vi "Position_TOTAL_R20.vi"(5 "Distance Between \nCameras  (*unit)":sgl=2.5) -> (12 "dX, dY\nLeft Cam":cluster{"X":sgl[], "Y":sgl[]}={"X"=[-5.750775, -4.1849813, -3.081379, -2.0098581, 0.0], "Y"=[7.9585915, 7.9595685, 7.960258, 7.960927, 0.0]}, 13 "Position Valid":bool=TRUE, 14 "Left Camera Real Coordinates":cluster{"X":sgl, "Y":sgl}={"X"=7.9602513, "Y"=5.592073}, 16 "dX, dY\nRight Cam":cluster{"X":sgl[], "Y":sgl[]}={"X"=[-7.3032045, -5.737411, -4.6338086, -3.5622878, -1.5524296], "Y"=[7.2714148, 7.2723923, 7.2730813, 7.273751, -0.68717635]}, 18 "Robot Coordinates":cluster{"X":sgl, "Y":sgl}={"X"=7.616663, "Y"=6.3682876}, 19 "Orietnation\n(current)":sgl=-23.843685 format="%#_13g")   [LabVIEW 2015]
uses:
  <vilib>/Analysis/NI_AALPro.lvlib
  <vilib>/myRIO/Instrument Drivers/Onboard IO/DIO/DIO.lvlib
  <vilib>/Analysis/coordinate.llb/2D Cartesian Coordinate Rotation (Array).vi
  <vilib>/Instr/_visa.llb/VISA Configure Serial Port (Instr).vi
panel:
  out "Current Cam State - L":T1(ring)
  out "Valid Beacon Sets_":bool[](array[boolean])=[TRUE, TRUE, TRUE, TRUE, FALSE]
  in  "Distance Threshold\nRef Triangles (*unit)":sgl=30.0
  out "dA2 4":sgl=9.6935425 format="%#_13g"
  out "dA2 2":sgl=9.6935425 format="%#_13g"
  out "dA2 3":sgl=9.6935425 format="%#_13g"
  out "Current Cam State - R":T1(ring)
  out "Beacon Scales - Left":sgl[](array[numeric])=[76.306, 116.841255, 157.35043, 195.67218, 0.0]
  out "Beacon Scales - Right":sgl[](array[numeric])=[76.306, 116.841255, 157.35043, 195.67218, 0.0]
  in  "New Orientation \nThreshold":sgl=10.0
  in  "Moving Average\nWindow Length":u8=5
  out "Current Recovery State -L":enum16{"Generic Sweep", "Recovery Search"}(ring)=enum."Recovery Search"
  out "Current Move Delta - L 2":u16
  out "Next Recovery State - Left":enum16{"Generic Sweep", "Recovery Search"}(ring)=enum."Recovery Search"
  out "Next Recovery State - Right":enum16{"Generic Sweep", "Recovery Search"}(ring)=enum."Recovery Search"
  out "Current Recovery State - Right":enum16{"Generic Sweep", "Recovery Search"}(ring)=enum."Recovery Search"
  in  "Initial Recovery State  - Right":enum16{"Generic Sweep", "Recovery Search"}(ring)=enum."Recovery Search"
  in  "Initial Recovery State - L":enum16{"Generic Sweep", "Recovery Search"}(ring)=enum."Recovery Search"
  out "Next Tracking State - Right":enum16{"Track", "Reactive Predict", ""}(ring)
  out "Current Tracking State - Right 2":enum16{"Track", "Reactive Predict", ""}(ring)
  in  "Initial Tracking State - Right":enum16{"Track", "Reactive Predict", ""}(ring)
  out "Last Track Angle - R":sgl=98.61328
  out "Next Tracking State - Left":enum16{"Track", "Reactive Predict", ""}(ring)
  in  "Initial Tracking State - Left":enum16{"Track", "Reactive Predict", ""}(ring)
  out "Current Tracking State - Left":enum16{"Track", "Reactive Predict", ""}(ring)
  in  "Timeout to \nEnable Reactive Predict":u16=5
  out "Tracking Timeout\nCount - R":i32
  in  "Tracking Timeout\nThreshold":i32=10
  out "Tracking Timeout\nCount - L":i32
  in  "Search Direction - in - Right":bool=TRUE
  out "Next Main State - Right":T2(ring)=enum."Tracking"
  in  "Recovery Search\nDirection - R":bool
  out "Recovery Mode Count in Right":i32
  out "Frames Processed\nCount - in Right":i32
  out "Recovery Search\nmove Count - Right":u16
  out "Recovery Search\nAttempt Count - Right":u16
  in  "Mounting Offset - Right":sgl=45.0
  in  "Tracking Angle - Right":sgl=98.60307
  in  "Current Servo Position\n- Right":u16
  out "New Data  Flag\nRight Servo":bool
  in  "Track Angle Valid  - Right":bool=TRUE
  out "Current Main State - Right":T2(ring)=enum."Tracking"
  in  "Initial Main State- Right":T2(ring)
  in  "Recovery Search\nDirection - L 2":bool
  in  "Max Recovery Count\n(Recovery Search) 2":u16
  in  "Max Recovery\nSearch Attempts 2":u16
  in  "Image Lock - Right 2":bool
  out "Last Track Angle - L":sgl=87.24609
  in  "Recovery Search\nDirection - L":bool=TRUE
  out "Next Main State - Left":T2(ring)=enum."Tracking"
  out "Current Move Delta - L":u16
  in  "Max Recovery Count\n(Recovery Search)":u16=10
  in  "Max Recovery\nSearch Attempts":u16=3
  out "Recovery Search\nAttempt Count - in - L":u16
  out "Recovery Search\nmove Count - in - L":u16
  in  "Image Lock - Right":bool=TRUE
  out "Recovery Mode Count - in Left":u16
  in  "Middle Beacon\nCoordinates":cluster{"X":sgl, "Y":sgl}={"X"=0.0, "Y"=2.5}
  in  "Min Num Frames\nper Search":i32=2
  in  "Wait Tick Threshold":i32=10
  out "Frames Processed\nCount - in -L":i32
  in  "Maximum Move \nServo Threshold":i16=300
  in  "Minimum Delta \nServo Threshold":i16=3
  in  "Mounting Offset - Left":sgl=-45.0
  in  "Search Step Size":u16=50
  in  "Search Direction - in - L":bool
  in  "Current Servo Position\n- Left":u16
  in  "Tracking Angle - Left":sgl=87.25689
  out "New Data  Flag\nLeft Servo":bool
  in  "Track Angle Valid - Left":bool=TRUE
  in  "Image Lock - Left":bool=TRUE
  in  "Initial Main State - Left":T2(ring)
  out "Current Main State - Left":T2(ring)=enum."Tracking"
  in  "Position Calc\nTimer":u32=100 caption="Position Calc Timer"
  in  "Fetch Input\n(mSec)":u32=20 caption="Update Camera Input\n(mSec)"
  out "Right Data\nInput Flag\n- Internal":bool=TRUE
  in  "Position Calc\nReady":bool
  out "This Servo \nAngle - Right":sgl=98.90625
  in  "Beacon Angles -R":sgl[](array[numeric])=[111.28093, 105.355774, 98.60307, 92.04714, 103.90625]
  in  "Beacon Angles - L":sgl[](array[numeric])=[101.98467, 94.59042, 87.25689, 80.30646, 91.66016]
  in  "Valid Angles -R":bool[](array[boolean])=[TRUE, TRUE, TRUE, TRUE, FALSE]
  in  "Valid Angles - L":bool[](array[boolean])=[TRUE, TRUE, TRUE, TRUE, FALSE]
  out "Left Data\nInput Flag\n- Internal":bool
  in  "Check Shared Var Timer":u32=50 caption="Main Loop\n Timer (ms)"
  out "Left_Flag 2":bool
  out "Right_Flag 2":bool
  out "Beacons Found\n- Left (Bool Array) 2":bool[](array[boolean])=[TRUE, TRUE, TRUE, TRUE, FALSE]
  out "LEFT Beacon Coord - X px (IN) 2":sgl[](array[numeric])=[76.306, 116.841255, 157.35043, 195.67218, 0.0]
  out "LEFT Beacon Position - Y px (IN) 2":sgl[](array[numeric])=[154.30304, 148.59094, 148.39949, 146.94655, 0.0]
  out "This Servo \nAngle - Left":sgl=86.66016
  in  "Compliance Slope":u8=128
  out "deltaMoveServo\n- R":i16
  out "Move Respond - R":bool
  out "Move Respond - L":bool
  out "Last Position":cluster{"X":sgl, "Y":sgl}={"X"=7.6261, "Y"=6.350474}
  out "Last Orientation":sgl=-23.876373
  in  "Distance\nBetween Beacons \n- Tolerance":sgl=0.35 format="%#_13g"
  in  "Distance\nBetween Beacons":sgl=1.0 format="%#_13g"
  out "dT":dbl=143.499
  out "Position Valid\nHistory":bool[](array[boolean])=[TRUE, FALSE, FALSE, TRUE, TRUE, FALSE, TRUE, TRUE, TRUE, TRUE, TRUE, TRUE, FALSE, TRUE, FALSE]
  out "Orientation\nHistory":sgl[](array[numeric])=[-23.876373, 0.0, 0.0, -23.938759, -24.0458, 0.0, -23.14014, -22.504314, -22.596928, -22.90728, -23.237453, -23.75214, 0.0, -23.808718, 0.0]
  out "Robot Coordinates\nHistory":cluster{sgl, sgl}[](array[cluster])=[{7.6261, 6.350474}, {0.0, 0.0}, {0.0, 0.0}, {7.63815, 6.33973}, {7.6316156, 6.322055}, {0.0, 0.0}, {7.6863523, 6.2558875}, {7.688662, 6.2228284}, {7.6736236, 6.2455945}, {7.6880507, 6.2819676}, {7.6893277, 6.3140097}, {7.668109, 6.3330927}, {0.0, 0.0}, {7.6506357, 6.3142757}, {0.0, 0.0}]
  in  "New Position \nThreshold":sgl=2.5
  out "Orientation Avgd":sgl=-23.876373
  in  "History Size":u8=15
  in  "Max Y (arena)":sgl=15.0
  in  "Max X (arena)":sgl=35.0
  in  "New Position\nWeight":sgl=0.5 format="%#_13g"
  in  "Max Std Dev (3)":sgl=0.2 format="%#_13g"
  in  "Max Std Dev (4)":sgl=0.2 format="%#_13g"
  out "Post Filtering\n- Valid Beacons":bool[](array[boolean])=[FALSE, TRUE, TRUE, TRUE, FALSE]
  out "Robot Coordinates - Avgd":cluster{"X":sgl, "Y":sgl}={"X"=7.6261, "Y"=6.350474}
  out "Real Position in Course 2":cluster{"X":dbl[], "Y":dbl[]}(graph)={"X"=[7.626100046018056], "Y"=[6.35047366782369]}
  out "Position \nLock Status":bool=TRUE
  out "Right Camera Real Coordinate":cluster{"X":sgl, "Y":sgl}={"X"=7.2730746, "Y"=7.1445026}
  out "deltaMoveServo\n- L":i16
  in  "Search Step Size\n(deg)":sgl=15.0 format="%#_13g"
  out "Beacons Found\n- Right (Bool Array)":bool[](array[boolean])=[TRUE, TRUE, TRUE, TRUE, FALSE]
  out "RIGHT Beacon Position - Y px (IN)":sgl[](array[numeric])=[153.02994, 149.48933, 150.4864, 150.33003, 0.0]
  out "RIGHT Beacon Coord - X px (IN)":sgl[](array[numeric])=[91.3685, 123.99656, 161.27843, 197.4523, 0.0]
  in  "Right Servo\nID":string="\u0001"
  in  "Servo Comm\nWait Time - (ms)":i32
  in  "Left Servo\nID":string="\u0000"
  out "dT - Comm Loop":u32=19
  in  "Servo Comm\nLoop Time (ms)":i32=20
  in  "close comms":bool
  in  "Max Read\nTx Attempts":u8=3
  in  "Max Write\nTx Attempts":u8=3
  out "Current R (10bit)":u16=696
  out "Servo Moving - R":bool
  out "Servo Moving - L":bool
  out "Current L (10bit)":u16=347
  in  "SERVO ENABLE":bool=TRUE
  out "Move Servo - L":bool
  out "Move Servo - R":bool
  in  "Servo Goal Position\n - Right":u16=695
  in  "Move Servo\nThreshold (deg)":sgl=2.0 format="%#_13g"
  in  "Servo Algorithm\nCycle Time(ms)":i32=25
  in  "Servo Goal Position\n - Left":u16=349
  in  "Current Angle\n - Left (internal)":sgl=86.66016
  in  "Current Angle\n - Right (internal)":sgl=98.90625
  in  "stop":bool
  in  "Num of Beacons (Total)":i8=5
  out "Angle to Pixel Ratios":T3={"Angle to Pixel\nRatio - Horizontal"=0.18125, "Angle to Pixel\nRatio - Vertical"=0.1875} {"Angle to Pixel\nRatio - Vertical" format="%#_13g"; "Angle to Pixel\nRatio - Horizontal" format="%#_13g"}
  in  "Cam AOV Vertical (deg)":sgl=45.0
  in  "Cam AOV Horizontal (deg)":sgl=58.0
  in  "Image Height (px)":sgl=240.0
  in  "Image Width (px)":sgl=320.0
  out "Beacon Coordinates - Left Image":T4={"Beacon Position - X px"=[76.306, 116.841255, 157.35043, 195.67218, 0.0], "Beacon Position - Y px"=[154.30304, 148.59094, 148.39949, 146.94655, 0.0]}
  out "Beacon Coordinates - Right Image":T4={"Beacon Position - X px"=[91.3685, 123.99656, 161.27843, 197.4523, 0.0], "Beacon Position - Y px"=[153.02994, 149.48933, 150.4864, 150.33003, 0.0]}
  out "Distance to LBF":sgl[](array[numeric])=[0.024284193, 0.015691843, 0.008273765, 0.028971607, 0.03291407]
  out "Local Coordinates - Calculated":cluster{sgl[], sgl[]}(graph)={[-2.0384164, -0.70265853, 0.4090246, 1.3811935, 0.0], [9.602626, 8.751521, 8.536832, 8.085801, 0.0]}
  out "Local Coordinates - Rotated":cluster{dbl[], dbl[]}(graph)={[1.5524295802029098, -5.750774735805926, -4.1849814062260675, -3.0813788557258652, -2.009858210562305, 0.0], [0.6871763361707266, 7.9585912385832795, 7.959568450875426, 7.960257859242679, 7.960927027680405, 0.0]}
  out "All Object Coordinates \n- Local - Rotated":cluster{"X":sgl[], "Y":sgl[]}={"X"=[1.5524296, -5.750775, -4.1849813, -3.081379, -2.0098581, 0.0], "Y"=[0.68717635, 7.9585915, 7.9595685, 7.960258, 7.960927, 0.0]}
  out "Local Coordinates - Normalized":cluster{sgl[], dbl[]}(graph)={[1.6977187, -2.0372734, -0.60508364, 0.4043527, 1.3844445, 0.0], [0.0, 9.605212211608887, 8.972328186035156, 8.526259422302246, 8.093157768249512, 0.0]}
  in  "Max Std Dev (5)":sgl=0.2 format="%#_13g"
  out "All Object Coordinates \n- Local":cluster{"X":sgl[], "Y":sgl[]}={"X"=[1.6977187, -2.0372734, -0.60508364, 0.4043527, 1.3844445, 0.0], "Y"=[0.0, 9.605212, 8.972328, 8.526259, 8.093158, 0.0]}
  out "LOCAL\nBeacon Coordinates\nRelative to Robot":cluster{"dX_beacon":sgl[], "dY_beacon":sgl[]}={"dX_beacon"=[-2.0384164, -0.70265853, 0.4090246, 1.3811935, 0.0], "dY_beacon"=[9.602626, 8.751521, 8.536832, 8.085801, 0.0]}
  in  "Real Beacon\n - Coordinates":cluster{"X":dbl[], "Y":dbl[]}={"X"=[0.0, 0.0, 0.0, 0.0, 0.0, 0.0], "Y"=[0.5, 1.5, 2.5, 3.5, 4.5, 0.0]}
  # "POSITION CALCULATION VARIABLES"
  # "OUTPUT VALUES"
  # "CONFIG VALUES"
  # "FILTER CONFIG VALUES"
  # "FEEDBACK INPUT VALUES"
  # "INPUT VALUES"
  # "INTERMEDIATE VALUES"
  # "IMAGE TO ANGLE VARIABLES"
  # "VISION PROCESSEING INPUTS"
  # "Use moving average for previous orientation thresholds"
  # "INPUTS"
  # "CONFIG"
  # "OUTPUT VALUES"
  # "*********************"
  # "unfiltered"
  # "NEW FILTER VALS"
  # "Inter Beacon Distance Filtering"
  # "SERVO CONTROL VARIABLES"
  # "SERVO CONTROL VARIABLES"
  # "CONFIG"
  # "SHARED VARIABLE INPUTS"
  # "LOCAL VARIABLE INPUTS"
  # "INTERNRAL VARIABLES"
  # "SEARCH ROUTINE VARIABLES"
  # "MISC"
  # "SERVO IDs"
  # "CONTROL DELAYS"
  # "COMM LOOP DELAY"
  # "COMM PROTOCOL"
  # "SETTINGS"
  # "Make function of distance^^"
  # "**** only left side starts search\nat previously known good angle"
  # "LEFT SERVO"
  # "RIGHT SERVO"
  # "Main State Machine"
  # "Recovery State Machine"
  # "Current Track Angle Inputs"
  # "Servo Status Inputs"
  # "Main State Machine Inputs"
  # "Recovery State Machine Inputs"
  # "Current Track Angle Inputs"
  # "Servo Status Inputs"
  # "Recovery State Machine Feedback"
  # "Tracking State Machine Inputs"
  # "Tracking State Machine Inputs"
  # "NOTE: Must be 1 bigger than amount of beacons"
  # "NOTE: Must be 1 bigger than amount of beacons"
types:
  T1 = enum16{"Super Close Range", "Short Range", "Long Range"}
  T2 = enum16{"Start Up Search", "Tracking", "Recovery Mode", ""}
  T3 = cluster{"Angle to Pixel\nRatio - Horizontal":sgl, "Angle to Pixel\nRatio - Vertical":sgl}
  T4 = cluster{"Beacon Position - X px":sgl[], "Beacon Position - Y px":sgl[]}
  T5 = cluster{"Tracking Coordinates":cluster{"X":dbl, "Y":dbl}, "Current Valid":bool, "Current State - Out":enum16{"Sub - 2", "Sub - 3", "Sub - 4", "Normal - 5"}}
  T6 = enum16{"Sub - 2", "Sub - 3", "Sub - 4", "Normal - 5"}
  T7 = cluster{"Array of Double":dbl[], "Array of Double":dbl[]}
  T8 = typedef "DIO.lvlib/DIO Reference.ctl" = cluster{"myRIO Reference":T9, "DIO Channels List":T13}
  T9 = typedef "myRIO Generic Hardware Reference.ctl" = cluster{"myRIO Model":T10, "myRIO Hardware Reference":T11}
  T10 = typedef "Hardware Version Enum.ctl" = enum16{"Unknown", "myRIO-1900", "myRIO-1950", "roboRIO"}
  T11 = typedef "myRIO v1.0 Reference.ctl" = cluster{"Generic FPGA Reference":T12, "Allow multiple opens":bool}
  T12 = typedef "Generic FPGA Reference.ctl" = refnum<k20>
  T13 = typedef "DIO Channels List.ctl" = T14[]
  T14 = typedef "DIO Channels Enum.ctl" = enum16{"Not Connected", "C/DIO0", "C/DIO1", "C/DIO2", "C/DIO3", "C/DIO4", "C/DIO5", "C/DIO6", "C/DIO7", "A/DIO0", "A/DIO1", "A/DIO2", "A/DIO3", "A/DIO4", "A/DIO5", "A/DIO6", "A/DIO7", "A/DIO8", "A/DIO9", "A/DIO10", "A/DIO11", "A/DIO12", "A/DIO13", "A/DIO14", "A/DIO15", "B/DIO0", "B/DIO1", "B/DIO2", "B/DIO3", "B/DIO4", "B/DIO5", "B/DIO6", "B/DIO7", "B/DIO8", "B/DIO9", "B/DIO10", "B/DIO11", "B/DIO12", "B/DIO13", "B/DIO14", "B/DIO15", "LED0", "LED1", "LED2", "LED3", "Button0", "DIO/DIO0", "DIO/DIO1", "DIO/DIO2", "DIO/DIO3", "DIO/DIO4", "DIO/DIO5", "DIO/DIO6", "DIO/DIO7", "DIO/DIO8", "DIO/DIO9", "SPI/CS0", "SPI/CS1", "SPI/CS2", "SPI/CS3", "LED RADIO (Green)", "LED RADIO (Red)", "LED COMM (Green)", "LED COMM (Red)", "LED MODE (Green)", "LED MODE (Red)"}
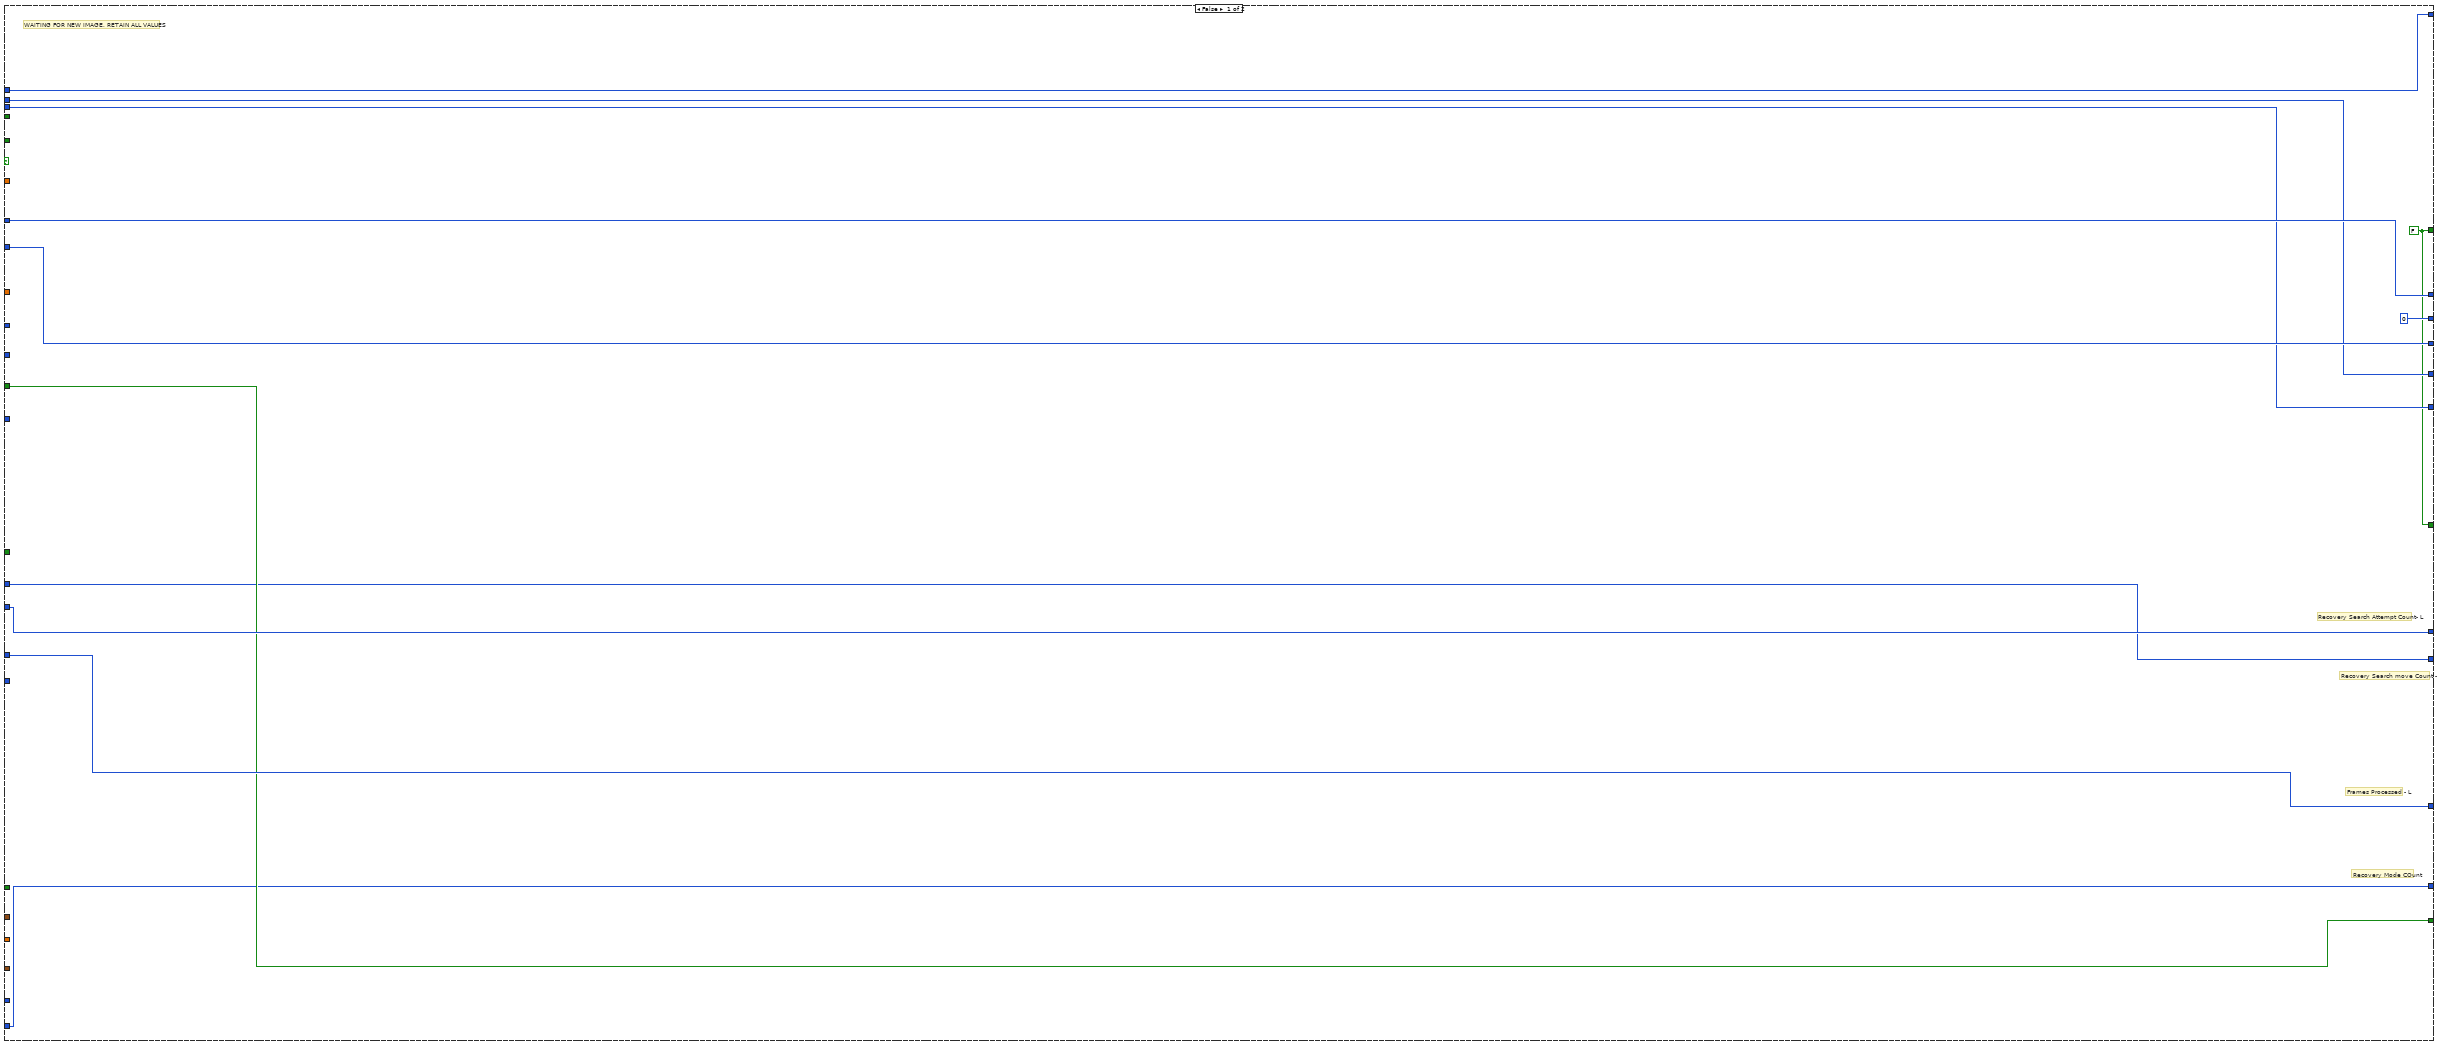
[diagram p2: hidden frame]
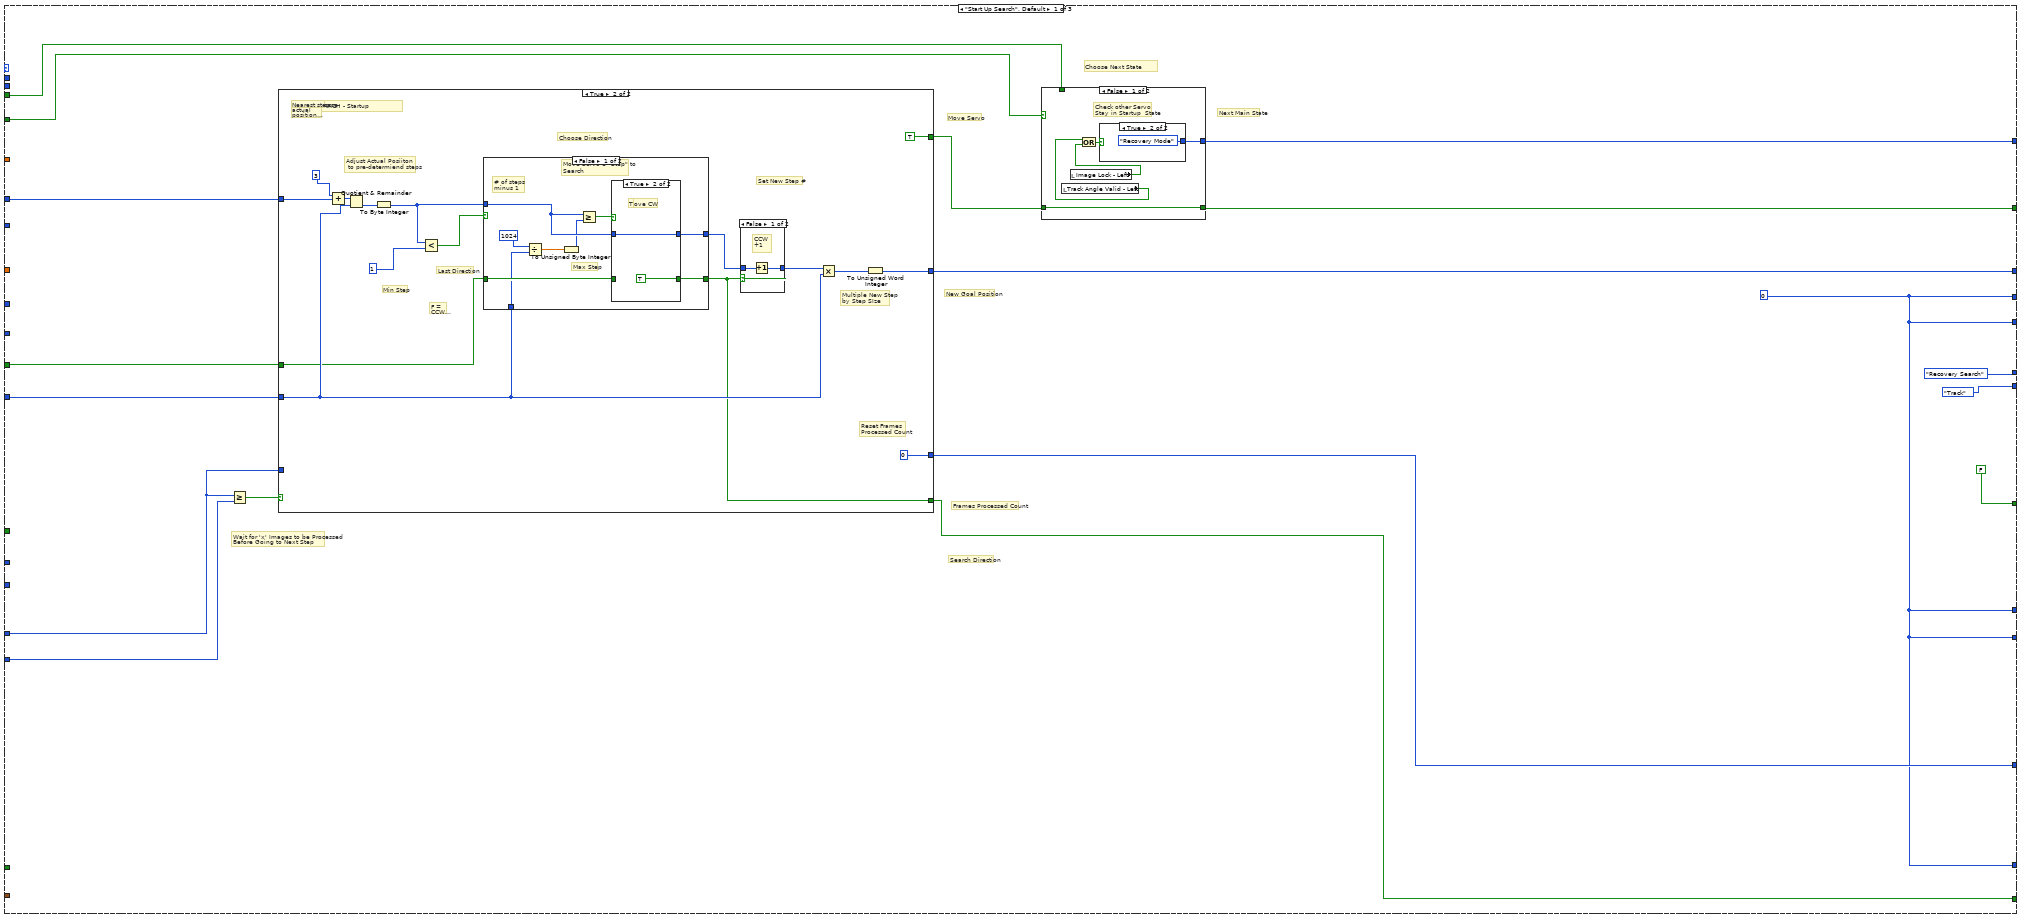
[diagram p3: hidden frame]
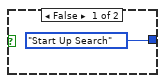
[diagram p4: hidden frame]
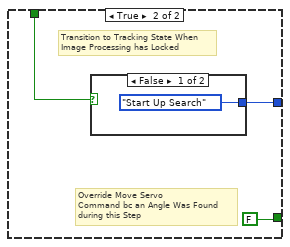
[diagram p5: hidden frame]
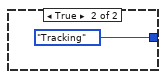
[diagram p6: hidden frame]
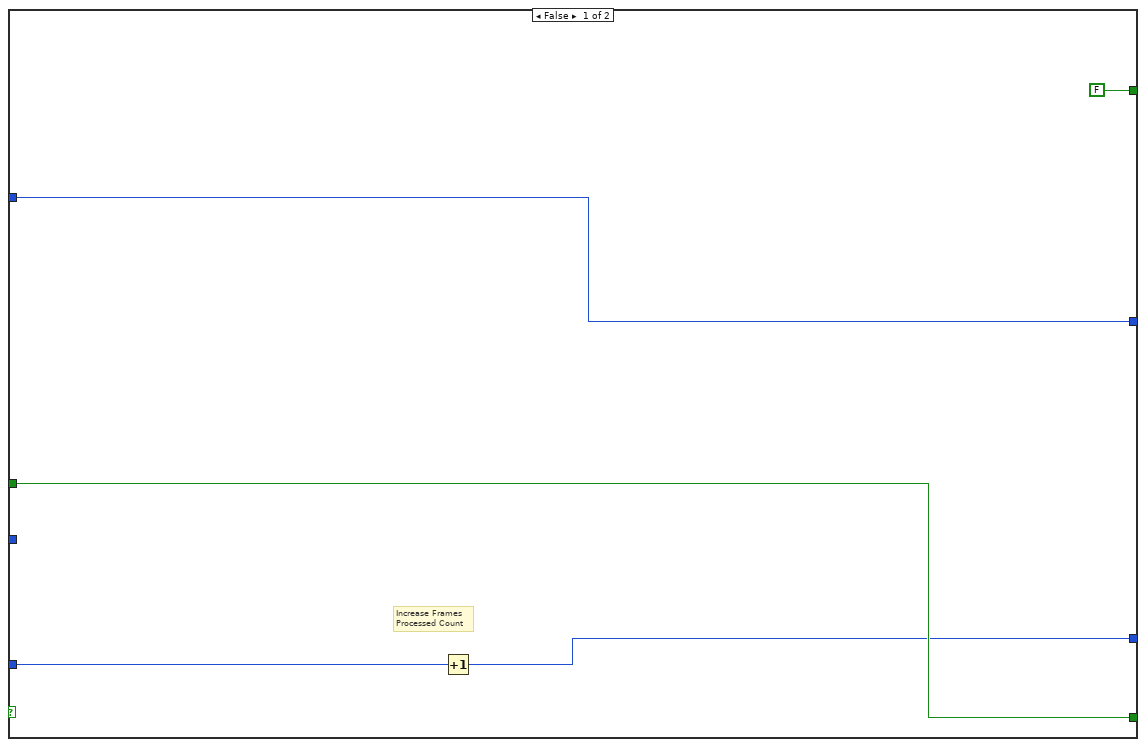
[diagram p7: hidden frame]
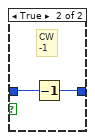
[diagram p8: hidden frame]
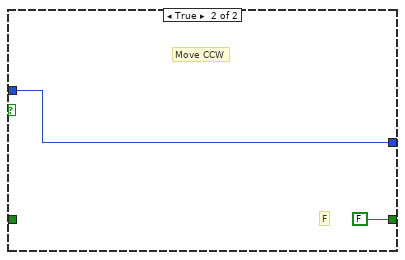
[diagram p10: hidden frame]
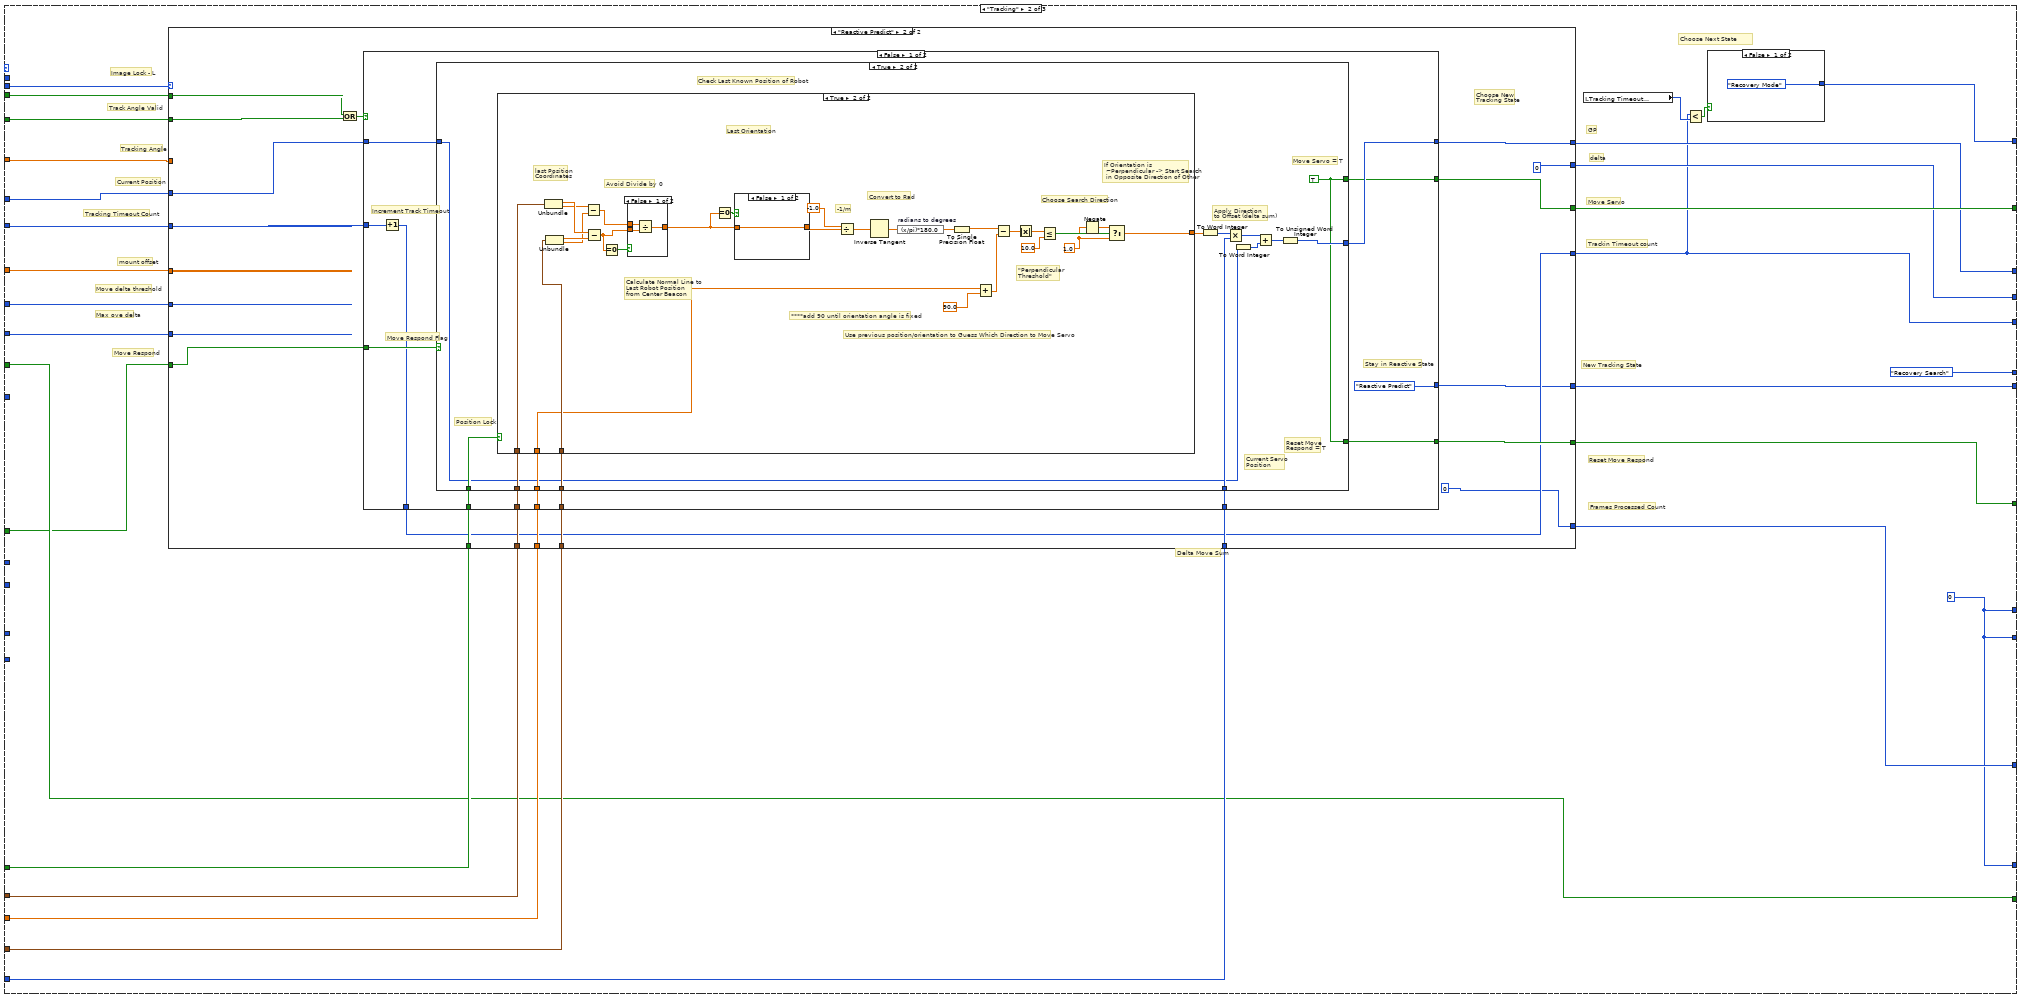
[diagram p11: hidden frame]
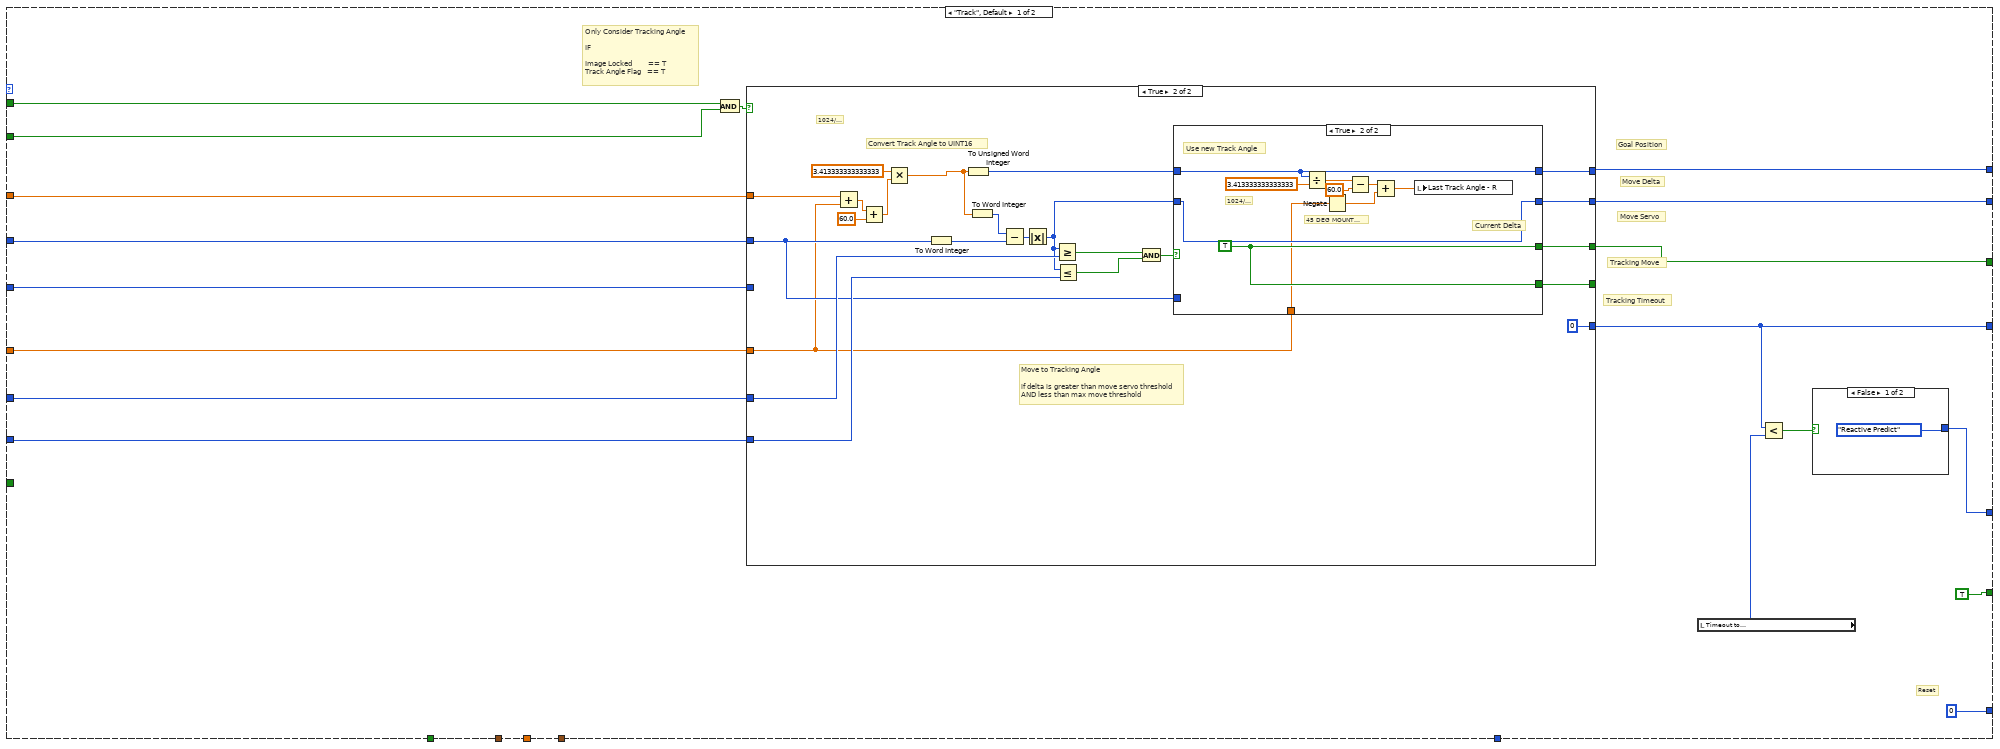
[diagram p12: hidden frame]
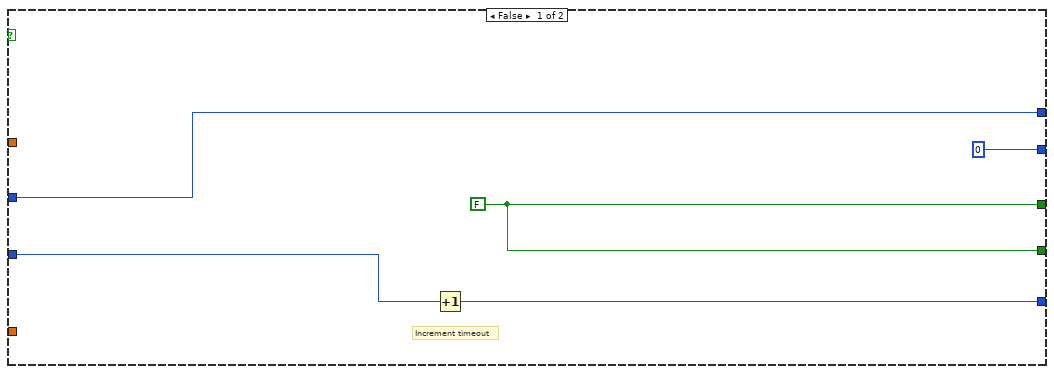
[diagram p13: hidden frame]
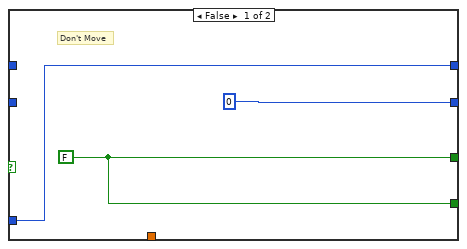
[diagram p14: hidden frame]
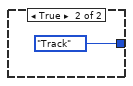
[diagram p15: hidden frame]
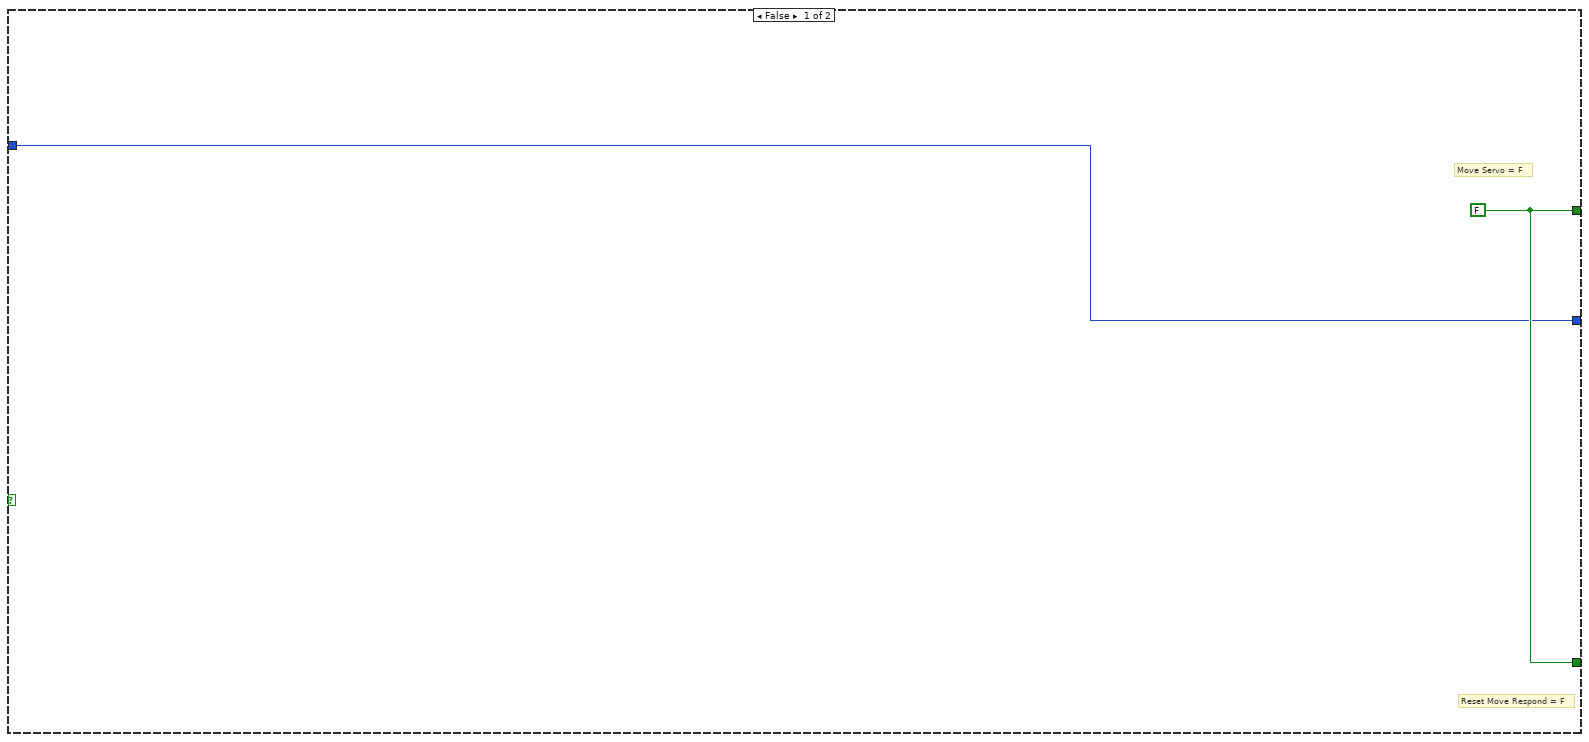
[diagram p16: hidden frame]
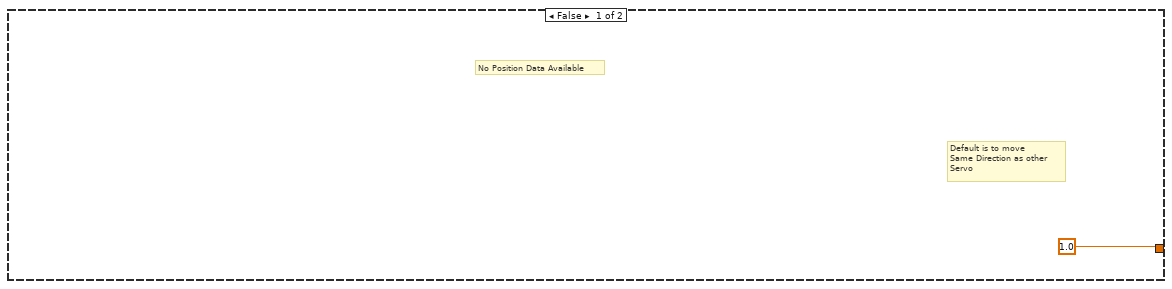
[diagram p17: hidden frame]
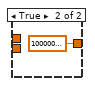
[diagram p18: hidden frame]
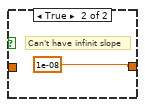
[diagram p19: hidden frame]
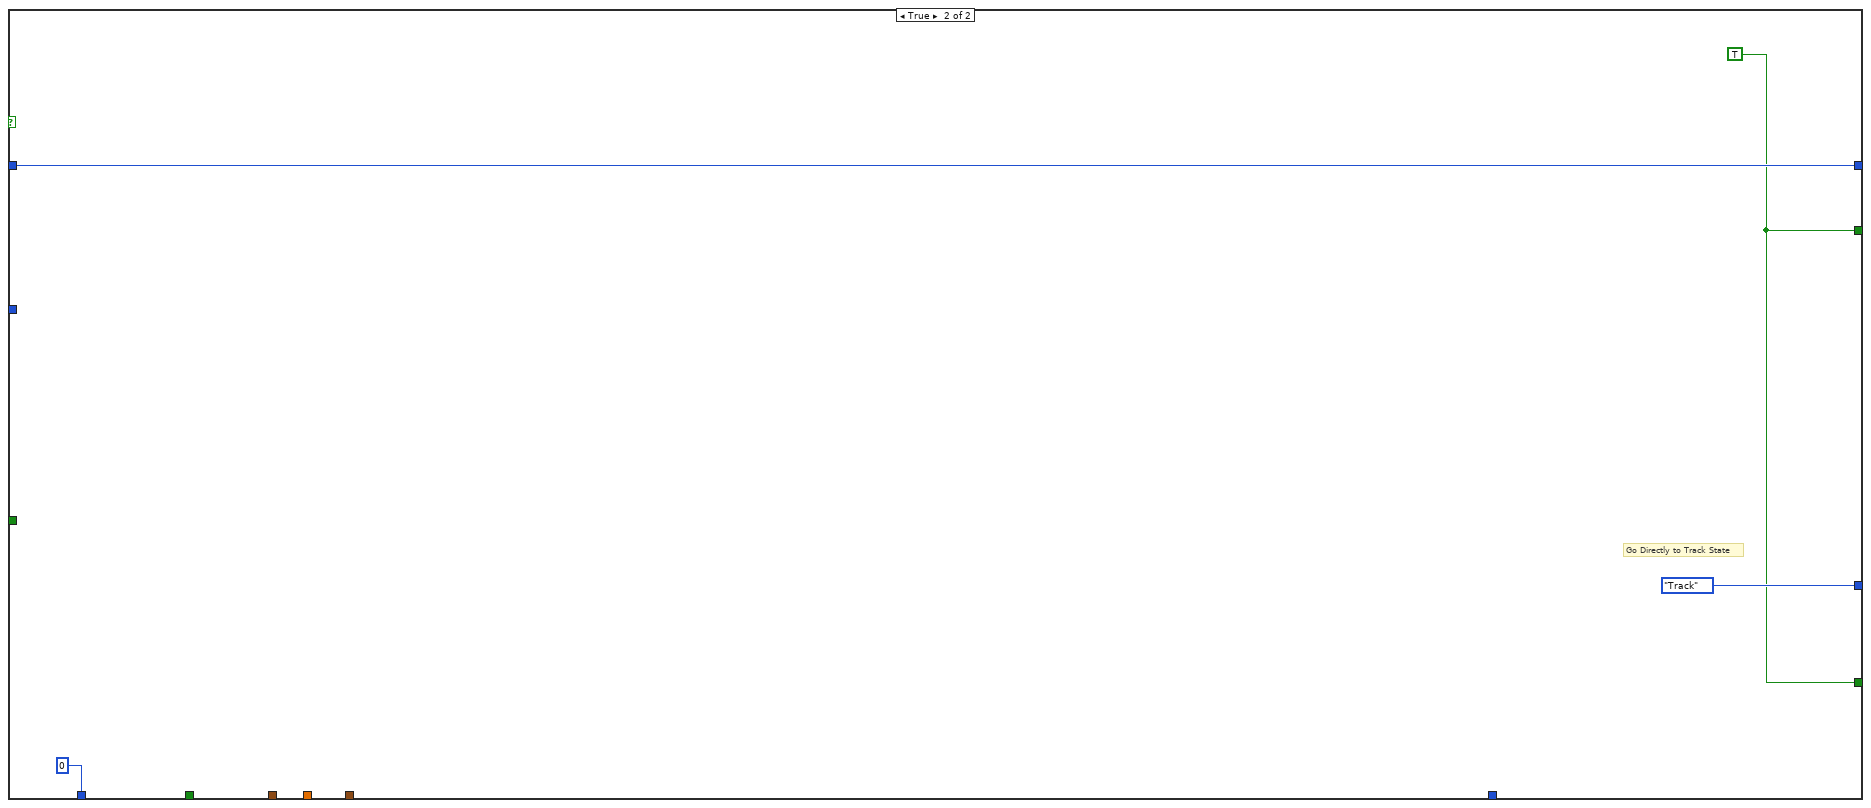
[diagram p20: hidden frame]
diagram:
  (unwired) enum16{"Generic Sweep", "Recovery Search"}."Recovery Search"
  w12 = 0 ("Frames Processed\nCount - in")
  w13 = 0 ("Frames Processed\nCount - in")
  w2 = FALSE
  w34 = sgl 0.0
  # "SERVO CONTROL FLAGS"
  # "***"
  # "Next Tracking State"
  # "Tracking Timeout Count"
  # "Search Direction - L"
  # "Next Recovery State"
  # "Move Respond"
  # "Recovery Mode Count - L"
  # "Delta Move Sum - L"
  # "Wait Tick Count - L"
  # "Frames Processed - L"
  # "Recovery Search move Count - L"
  # "Recovery Search Attempt Count- L"
  # "Next Main State"
  # "Search Direction - L"
  # "Next Recovery State"
  # "INPUTS - Local vars"
  # "Recovery Mode Count - L"
  # "Delta Move Sum - L"
  # "Frames Processed\nLeft"
  # "Move Respond - R"
  # "Initial Search Direction\n- Right"
  # "Move Respond"
  # "Recovery Mode Count - L"
  # "Delta Move Sum - L"
  # "Wait Tick Count - L"
  # "Frames Processed - L"
  # "Recovery Search move Count - L"
  # "Recovery Search Attempt Count- L"
  # "Next Main State"
  # "Settings -- Update in a slow loop"
  # "Recovery Mode Count - L"
  # "Delta Move Sum - L"
  # "Frames Processed\nLeft"
  # "Move Respond - L"
  # "Replace these with\nconstants"
  # "Initial Search Direction\n- Left"
  # "Read Inputs when Available"
  # "# of Physical Beacons"
  # "Right Data Internal Falg"
  # "Left Data Internal Falg"
  # "Initialize Shift Arrays"
  # "Robot Position (cluster)\nShift Array"
  # "Robot Position (cluster)\nShift Array"
  # "Position Valid Shift Array"
  # "Orientation Shift Array"
  # "Position Valid Shift Array"
  # "Orientation Shift Array"
  # "Servo Communication (to Servo- UART))"
  # "Internal Local Variables"
  # "Servo Control Logic"
  # "Local Variables"
  # "Images to Robot Position Calculation Process"
  # "SERVO MOTOR CONTROL"
  # "SERVO MOTOR CONTROL"
  n1 = Divide(x="Cam AOV Horizontal (deg)", y="Image Width (px)") -> (x/y=w25:sgl)
  n2 = Divide(x="Cam AOV Vertical (deg)", y="Image Height (px)") -> (x/y=w26:sgl)
  n3 = Bundle(w25, w26) -> (w20:cluster{sgl, sgl})  [unwired: 1 in]
  "Angle to Pixel Ratios" <- w20
  n4 = disable-structure shown="Disabled" {
    frame Disabled {
      # "Always Read Incoming Flags & Store"
      n5 = while {
        tunnel: "Check Shared Var Timer" -> [w46]
        stop <- FALSE stop-if-true
        n6 = shared-variable "myRIO-1900\\Lib1.lvlib\\RIGHT_FLAG"() -> (→"Right_Flag 2":bool)  [unwired: 1 in, 1 out]
        n7 = shared-variable "myRIO-1900\\Lib1.lvlib\\Left_Flag"() -> (→"Left_Flag 2":bool)  [unwired: 1 in, 1 out]
        n8 = call "Wait8"("Count(mSec)"=w46) -> ()  [unwired: 1 out]
      }
    }
    frame Enabled {
    }
  }
  n9 = while {
    shift-right: [w55] -> _
    shift-left: w2 -> [w60]
    shift-right: [w54] -> _
    shift-left: w2 -> [w58]
    tunnel: w20 -> [w56]
    tunnel: "Num of Beacons (Total)" -> [w57]
    stop <- FALSE stop-if-true
    # "Wait for Both Internal Flags"
    n10 = call "Wait6"("Count(mSec)"="Fetch Input\n(mSec)") -> ()  [unwired: 1 out]
    n11 = shared-variable "RT myRIO Target - Overlord\\Localization_Variables_r0.lvlib\\RIGHT_FLAG"() -> (w51:bool)  [unwired: 1 in, 1 out]
    n12 = shared-variable "RT myRIO Target - Overlord\\Localization_Variables_r0.lvlib\\Left_Flag"() -> (w52:bool)  [unwired: 1 in, 1 out]
    n13 = case shown="True" w51 {
      tunnel: w57 -> [_ w79]
      tunnel: w56 -> [_ w77]
      tunnel: [w61 w67] -> w49
      tunnel: w58 -> [w61 _]
      frame False {
        # "Don't Update Servo Position\nbc we're waiting on new Data to\ncome in and the servo position\nwas set at the previous set of data"
      }
      frame True {
        w67 = TRUE
        # "Store Values"
        # "Raise Internal Flag"
        # "If New Data Available"
        # "From Shift Reg"
        # "Perforrm Indivudual Angle Calculation"
        # "Pull Down Individual Flag"
        n14 = shared-variable "RT myRIO Target - Overlord\\Localization_Variables_r0.lvlib\\RIGHT_BEACON_X_array"() -> (w73:dbl[])  [unwired: 1 in, 1 out]
        "RIGHT Beacon Coord - X px (IN)" <- w73
        n15 = shared-variable "RT myRIO Target - Overlord\\Localization_Variables_r0.lvlib\\Image Lock - R"() -> (w68:bool)  [unwired: 1 in, 1 out]
        n16 = shared-variable "RT myRIO Target - Overlord\\Localization_Variables_r0.lvlib\\RIGHT_BEACON_Scales"() -> (→"Beacon Scales - Right":sgl[])  [unwired: 1 in, 1 out]
        n17 = shared-variable "RT myRIO Target - Overlord\\Localization_Variables_r0.lvlib\\Info - Right"() -> (w65:T5)  [unwired: 1 in, 1 out]
        n18 = shared-variable "RT myRIO Target - Overlord\\Localization_Variables_r0.lvlib\\RIGHT_BEACON_Y_array"() -> (w72:dbl[])  [unwired: 1 in, 1 out]
        "RIGHT Beacon Position - Y px (IN)" <- w72
        n19 = shared-variable "RT myRIO Target - Overlord\\Localization_Variables_r0.lvlib\\RIGHT_BEACON_BOOL_array"() -> (w71:bool[])  [unwired: 1 in, 1 out]
        "Beacons Found\n- Right (Bool Array)" <- w71
        n20 = Unbundle By Name(w65) -> ("Tracking Coordinates"=w64:cluster{"X":dbl, "Y":dbl}, "Current Valid"=w63:bool, "Current State - Out"=→"Current Cam State - R":T6)
        n21 = local write "Image Lock - Right"(w68) -> ()
        n22 = Bundle("Array of Double"=w73, "Array of Double"=w72) -> (w70:T7)  [unwired: 1 in]
        "Beacon Coordinates - Right Image" <- w70
        n23 = shared-variable "RT myRIO Target - Overlord\\Localization_Variables_r0.lvlib\\Right Servo Angle_Image"() -> (w69:dbl)  [unwired: 1 in, 1 out]
        "This Servo \nAngle - Right" <- w69
        n24 = shared-variable "RT myRIO Target - Overlord\\Localization_Variables_r0.lvlib\\RIGHT_FLAG"(FALSE) -> ()  [unwired: 1 in, 1 out]
        n25 = feedback #1() -> (w81:sgl[])  [unwired: 1 in]
        n26 = feedback #2() -> (w80:bool[])  [unwired: 1 in]
        n27 = call "Angle Calc_Individual Process R4.vi"("Angle to Pixel Ratios"=w77, "Previous Angles"=w81, "Num of Beacons"=w79, "Beacon Coordinates - Image"=w70, "Current Servo Angle"=w69, "Beacons Found (Bool Array)"=w71, "Previous Valid Angles"=w80, "Tracking Coordinates"=w64) -> ("Servo Goal Angle"=w76:sgl, "Valid Beacons (Bool Array)\nPosition Calc"=w75:bool[], "Angle Of Beacons \nRelative to Robot"=w74:sgl[])  [unwired: 4 in, 1 out]
        n28 = feedback-in #1(w74) -> ()
        n29 = feedback-in #2(w75) -> ()
        n30 = local write "Beacon Angles -R"(w74) -> ()
        n31 = local write "Tracking Angle - Right"(w76) -> ()
        n32 = local write "Valid Angles -R"(w75) -> ()
        n33 = local write "Track Angle Valid  - Right"(w63) -> ()
        n34 = local write "New Data  Flag\nRight Servo"(w67) -> ()
      }
    }
    "Right Data\nInput Flag\n- Internal" <- w49
    n35 = case shown="True" w52 {
      tunnel: [w82 w88] -> w48
      tunnel: w60 -> [w82 _]
      tunnel: w56 -> [_ w92]
      tunnel: w57 -> [_ w91]
      frame False {
        # "Don't Update Servo Position\nbc we're waiting on new Data to\ncome in and the servo position\nwas set at the previous set of data"
      }
      frame True {
        w88 = TRUE
        # "Store Values"
        # "Raise Internal Flag"
        # "If New Data Available"
        # "Perforrm Indivudual Angle Calculation"
        # "Pull Down Individual Flag"
        n36 = shared-variable ".\\Localization_Variables_r0.lvlib\\LEFT_BEACON_X_array"() -> (w98:dbl[])  [unwired: 1 in, 1 out]
        "LEFT Beacon Coord - X px (IN) 2" <- w98
        n37 = shared-variable "RT myRIO Target - Overlord\\Localization_Variables_r0.lvlib\\LEFT_BEACON_Scales"() -> (→"Beacon Scales - Left":sgl[])  [unwired: 1 in, 1 out]
        n38 = shared-variable "RT myRIO Target - Overlord\\Localization_Variables_r0.lvlib\\LEFT_BEACON_Y_array"() -> (w99:dbl[])  [unwired: 1 in, 1 out]
        "LEFT Beacon Position - Y px (IN) 2" <- w99
        n39 = shared-variable "RT myRIO Target - Overlord\\Localization_Variables_r0.lvlib\\LEFT_BEACON_BOOL_array"() -> (w100:bool[])  [unwired: 1 in, 1 out]
        "Beacons Found\n- Left (Bool Array) 2" <- w100
        n40 = shared-variable "RT myRIO Target - Overlord\\Localization_Variables_r0.lvlib\\Image Lock - L"() -> (w89:bool)  [unwired: 1 in, 1 out]
        n41 = shared-variable "RT myRIO Target - Overlord\\Localization_Variables_r0.lvlib\\Info - Left"() -> (w85:T5)  [unwired: 1 in, 1 out]
        n42 = Unbundle By Name(w85) -> ("Tracking Coordinates"=w84:cluster{"X":dbl, "Y":dbl}, "Current Valid"=w83:bool, "Current State - Out"=→"Current Cam State - L":T6)
        n43 = local write "Image Lock - Left"(w89) -> ()
        n44 = Bundle("Array of Double"=w98, "Array of Double"=w99) -> (w96:T7)  [unwired: 1 in]
        "Beacon Coordinates - Left Image" <- w96
        n45 = shared-variable "RT myRIO Target - Overlord\\Localization_Variables_r0.lvlib\\Left Servo Angle_Image"() -> (w90:dbl)  [unwired: 1 in, 1 out]
        "This Servo \nAngle - Left" <- w90
        n46 = shared-variable "RT myRIO Target - Overlord\\Localization_Variables_r0.lvlib\\Left_Flag"(FALSE) -> ()  [unwired: 1 in, 1 out]
        n47 = feedback #3() -> (w102:sgl[])  [unwired: 1 in]
        n48 = feedback #4() -> (w101:bool[])  [unwired: 1 in]
        n49 = call "Angle Calc_Individual Process R4.vi"("Angle to Pixel Ratios"=w92, "Previous Angles"=w102, "Num of Beacons"=w91, "Beacon Coordinates - Image"=w96, "Current Servo Angle"=w90, "Beacons Found (Bool Array)"=w100, "Previous Valid Angles"=w101, "Tracking Coordinates"=w84) -> ("Servo Goal Angle"=w95:sgl, "Valid Beacons (Bool Array)\nPosition Calc"=w94:bool[], "Angle Of Beacons \nRelative to Robot"=w93:sgl[])  [unwired: 4 in, 1 out]
        n50 = feedback-in #3(w93) -> ()
        n51 = feedback-in #4(w94) -> ()
        n52 = local write "Beacon Angles - L"(w93) -> ()
        n53 = local write "Valid Angles - L"(w94) -> ()
        n54 = local write "Tracking Angle - Left"(w95) -> ()
        n55 = local write "Track Angle Valid - Left"(w83) -> ()
        n56 = local write "New Data  Flag\nLeft Servo"(w88) -> ()
      }
    }
    "Left Data\nInput Flag\n- Internal" <- w48
    n57 = And(x=w48, y=w49) -> (x .and. y?=w59:bool)
    n58 = case shown="True" w59 {
      selector: w59 -> [_ w105]
      tunnel: w48 -> [w104 _]
      tunnel: [w104 w106] -> w55
      tunnel: [w103 w106] -> w54
      tunnel: w49 -> [w103 _]
      frame False {
      }
      frame True {
        w106 = FALSE
        # "Reset Internal Data Flags"
        # "Position Data\nReady Enabled"
        n59 = local write "Position Calc\nReady"(w105) -> ()
      }
    }
  }
  n60 = Bundle(w34, w34) -> (w37:cluster{sgl, sgl})  [unwired: 1 in]
  n61 = Initialize Array(w34, "History Size") -> (w32:sgl[])
  n62 = Initialize Array(w37, "History Size") -> (w33:cluster{sgl, sgl}[])
  n63 = Initialize Array(FALSE, "History Size") -> (w31:bool[])
  n64 = call "Tick Count4"() -> ("Tick Count(uSec)"=w30:u32)
  n65 = while {
    shift-right: [w117] -> _
    shift-left: w32 -> [w114]
    shift-right: [w116] -> _
    shift-left: w31 -> [w115]
    shift-right: [w118] -> _
    shift-left: w33 -> [w109]
    shift-right: [w110] -> _
    shift-left: w30 -> [w111]
    stop <- "stop" stop-if-true
    n66 = call "Wait5"("Count(mSec)"="Position Calc\nTimer") -> ()  [unwired: 1 out]
    n67 = case shown="True" "Position Calc\nReady" {
      selector: "Position Calc\nReady" -> [_ w160]
      tunnel: w109 -> [_ w183]
      tunnel: w109 -> [w127 w177]
      tunnel: w114 -> [w129 w176]
      tunnel: w115 -> [w128 w175]
      tunnel: [w129 w182] -> w117
      tunnel: [w128 w180] -> w116
      tunnel: [w127 w181] -> w118
      tunnel: w115 -> [_ w174]
      tunnel: w114 -> [_ w173]
      tunnel: [w126 w167] -> w112
      tunnel: w111 -> [_ w167]
      tunnel: [FALSE TRUE] -> w113
      tunnel: w109 -> [_ w162]
      frame False {
        n68 = call "Tick Count5"() -> ("Tick Count(uSec)"=w126:u32)
      }
      frame True {
        w138 = T1."Long Range" ("Current Cam State - R")
        # "At least 2+ Avaialbe"
        # "***********do for both"
        # "sTATE"
        # "CALCULATE AVERAGE ORIENTATION"
        # "Update Outputs\nif Current Calc is Invalid\n(shouldn't matter)"
        # "Estimate Orienation Based on Previous Position"
        # "****# of previous in history that must be true\nin order for position to be considered \"locked\""
        # "New Position is Valid if both \nOrientation and Positions\nis within range of previous"
        # "Robot Position\n Shift Array"
        # "Position Valid Shift Array"
        # "Orientation Shift Array"
        # "Orientation Value"
        # "Shift & Insert Current Position Valid"
        # "Position Valid\n(orientation)"
        # "Position Valid\n(position)"
        # "Update Shift Registers"
        # "Shift & Insert Current Calculated Orientation"
        # "Shift & Insert Current Robot Position"
        # "UPDATE FINAL OUTPUT\n VALUES"
        n69 = Not(x=w160) -> (.not. x?=w161:bool)
        n70 = local read "Num of Beacons (Total)"() -> (w145:i8)
        n71 = local write "Position Calc\nReady"(w161) -> ()
        n72 = local read "Current Cam State - L"() -> (w139:T1)
        n73 = local read "Current Cam State - R"() -> (w137:T1)
        n74 = local read "Beacon Scales - Left"() -> (w151:sgl[])
        n75 = local read "Beacon Scales - Right"() -> (w154:sgl[])
        n76 = Equal?(x=w139, y=w138) -> (x = y?=w135:bool)
        n77 = Equal?(x=w137, y=w138) -> (x = y?=w134:bool)
        n78 = And(x=w135, y=w134) -> (x .and. y?=w136:bool)
        n79 = case shown="False" w136 {
          tunnel: "Beacon Angles - L" -> [w494 w619]
          tunnel: w145 -> [w493 w607]
          tunnel: w151 -> [w492 _]
          tunnel: "Beacon Angles -R" -> [w491 w618]
          tunnel: w154 -> [w490 _]
          tunnel: "Valid Angles -R" -> [w489 w623]
          tunnel: "Valid Angles - L" -> [w488 w624]
          tunnel: "Distance Between \nCameras  (*unit)" -> [w487 w620]
          tunnel: [w486 w602] -> w144
          tunnel: [w485 w601] -> w147
          tunnel: [w484 w600] -> w146
          frame False {
            # "System is not in NORMAL (long range) Mode"
            # "Estimate Distance for each Available Beacon Angle\nPER Camera, indivduallly"
            n80 = for {
              N: w493 -> [_]
              tunnel: w488 -> [w499] mode=indexing
              tunnel: w494 -> [w508] mode=indexing
              tunnel: w492 -> [w509] mode=indexing
              tunnel: w489 -> [w498] mode=indexing
              tunnel: w491 -> [w507] mode=indexing
              tunnel: w490 -> [w506] mode=indexing
              tunnel: w487 -> [w505]
              tunnel: [w497] -> w485 mode=indexing
              tunnel: [w496] -> w484 mode=indexing
              tunnel: [w495] -> w486 mode=indexing
              # "dY"
              # "dX"
              # "Valid"
              # "If Both Cameras are using Same Beacon Data,\nAverage the 2 independently esitmated positions"
              # "dY"
              # "dX"
              # "dY"
              # "dX"
              n81 = case shown="True" w499 {
                tunnel: w508 -> [_ w586]
                tunnel: [w573 w577] -> w503
                tunnel: [w573 w578] -> w502
                tunnel: w509 -> [_ w576]
                frame False {
                  w573 = sgl 0.0
                  # "Current Data Set Was Not Valid\nFill with 0\nWill not be used later"
                }
                frame True {
                  # "Estimate Distance"
                  # "Negate dX if A2>90"
                  # "Find LOCAL Coordinate of Each Beacon"
                  # "Current - Valid Data Set"
                  n82 = call "Scaling and Mapping"("Signals"=w576) -> ("Scaled Signals"=w575:dynamicdata)  [unwired: 9 in, 1 out]
                  n83 = To Single Precision Float(number=w575) -> (single precision float=w574:sgl)
                  n84 = Less?(x=w586, y=sgl 90.0) -> (x < y?=w588:bool)
                  n85 = case shown="False" w588 {
                    tunnel: w586 -> [w595 w597]
                    tunnel: [w593 w598] -> w585
                    tunnel: [FALSE TRUE] -> w580
                    frame False {
                      # "Negative Y"
                      # "A2 is > 90"
                      n86 = Subtract(x=w595, y=sgl 90.0) -> (x-y=w593:sgl)
                    }
                    frame True {
                      # "Positive Y"
                      # "A2 is < 90"
                      n87 = Subtract(x=sgl 90.0, y=w597) -> (x-y=w598:sgl)
                    }
                  }
                  "dA2 2" <- w585
                  n88 = expression code="(x/180.0)*pi" "degrees to radians"(w585) -> (w583:sgl)
                  n89 = expression code="(x/180.0)*pi" "degrees to radians"(w585) -> (w584:sgl)
                  n90 = Cosine(x=w583) -> (cos(x)=w581:sgl)
                  n91 = Sine(x=w584) -> (sin(x)=w582:sgl)
                  n92 = Multiply(x=w574, y=w581) -> (x*y=w578:sgl)
                  n93 = Multiply(x=w574, y=w582) -> (x*y=w579:sgl)
                  n94 = case shown="True" w580 {
                    tunnel: w579 -> [w590 w591]
                    tunnel: [w589 w591] -> w577
                    frame False {
                      n95 = Negate(x=w590) -> (-x=w589:sgl)
                    }
                    frame True {
                    }
                  }
                }
              }
              n96 = case shown="True" w498 {
                tunnel: w507 -> [_ w559]
                tunnel: [w544 w546] -> w501
                tunnel: [w544 w545] -> w500
                tunnel: w506 -> [_ w551]
                tunnel: w505 -> [_ w548]
                frame False {
                  w544 = sgl 0.0
                  # "Current Data Set Was Not Valid\nFill with 0\nWill not be used later"
                }
                frame True {
                  # "Add delta for\nRIGHT camera ONLY"
                  # "Estimate Distance"
                  # "Negate dX if A2>90"
                  # "Find LOCAL Coordinate of Each Beacon"
                  # "Current - Valid Data Set"
                  n97 = call "Scaling and Mapping2"("Signals"=w551) -> ("Scaled Signals"=w550:dynamicdata)  [unwired: 9 in, 1 out]
                  n98 = To Single Precision Float(number=w550) -> (single precision float=w549:sgl)
                  n99 = Less?(x=w559, y=sgl 90.0) -> (x < y?=w561:bool)
                  n100 = case shown="False" w561 {
                    tunnel: w559 -> [w568 w570]
                    tunnel: [w566 w571] -> w558
                    tunnel: [FALSE TRUE] -> w553
                    frame False {
                      # "Negative Y"
                      # "A2 is > 90"
                      n101 = Subtract(x=w568, y=sgl 90.0) -> (x-y=w566:sgl)
                    }
                    frame True {
                      # "Positive Y"
                      # "A2 is < 90"
                      n102 = Subtract(x=sgl 90.0, y=w570) -> (x-y=w571:sgl)
                    }
                  }
                  "dA2 3" <- w558
                  n103 = expression code="(x/180.0)*pi" "degrees to radians"(w558) -> (w556:sgl)
                  n104 = expression code="(x/180.0)*pi" "degrees to radians"(w558) -> (w557:sgl)
                  n105 = Cosine(x=w556) -> (cos(x)=w554:sgl)
                  n106 = Sine(x=w557) -> (sin(x)=w555:sgl)
                  n107 = Multiply(x=w549, y=w554) -> (x*y=w545:sgl)
                  n108 = Multiply(x=w549, y=w555) -> (x*y=w552:sgl)
                  n109 = case shown="True" w553 {
                    tunnel: w552 -> [w563 w564]
                    tunnel: [w562 w564] -> w547
                    frame False {
                      n110 = Negate(x=w563) -> (-x=w562:sgl)
                    }
                    frame True {
                    }
                  }
                  n111 = Add(x=w548, y=w547) -> (x+y=w546:sgl)
                }
              }
              n112 = And(x=w499, y=w498) -> (x .and. y?=w504:bool)
              n113 = case shown="False" w504 {
                tunnel: w503 -> [w517 w543]
                tunnel: w502 -> [w514 w542]
                tunnel: w501 -> [w516 w541]
                tunnel: w500 -> [w515 w540]
                tunnel: [w512 w536] -> w497
                tunnel: [w511 w535] -> w496
                tunnel: w499 -> [w513 _]
                tunnel: w498 -> [w518 _]
                tunnel: [w510 TRUE] -> w495
                frame False {
                  n114 = Exclusive Or(1:w518, 2:w513) -> (0:w519:bool)
                  n115 = case shown="True" w519 {
                    tunnel: w517 -> [_ w527]
                    tunnel: w516 -> [_ w524]
                    tunnel: w515 -> [_ w523]
                    tunnel: w514 -> [_ w525]
                    tunnel: w513 -> [_ w529]
                    tunnel: [w520 w528] -> w512
                    tunnel: [w520 w526] -> w511
                    tunnel: [FALSE TRUE] -> w510
                    frame False {
                      w520 = sgl 0.0
                      # "None are valid,"
                    }
                    frame True {
                      # "Only 1 beacon is valid,\nUse the valid beacon"
                      n116 = case shown="False" w529 {
                        tunnel: [w531 w533] -> w528
                        tunnel: w527 -> [_ w533]
                        tunnel: [w530 w532] -> w526
                        tunnel: w525 -> [_ w532]
                        tunnel: w524 -> [w531 _]
                        tunnel: w523 -> [w530 _]
                        frame False {
                          # "Left is invalid,\nRight MUST be valid"
                        }
                        frame True {
                          # "Left is Valid"
                        }
                      }
                    }
                  }
                }
                frame True {
                  w537 = sgl 2.0 ("y")
                  # "Both are Valid"
                  n117 = Add(x=w543, y=w541) -> (x+y=w538:sgl)
                  n118 = Add(x=w542, y=w540) -> (x+y=w539:sgl)
                  n119 = Divide(x=w539, y=w537) -> (x/y=w535:sgl)
                  n120 = Divide(x=w538, y=w537) -> (x/y=w536:sgl)
                }
              }
            }
          }
          frame True {
            # "dY"
            # "dX"
            # "Valid"
            # "Find Local Coordinates"
            # "Valid COunt"
            # "Make sure 2+ Data Sets are Still available"
            # "Check 1st element\nwith rest of elements"
            # "Make Sure all Pointed \nIn Same Direction"
            # "For Each Valid Beacon\nCalculate Distance from Each Camera to Each Beacon"
            # "Find Common Beacons\nAmong Cameras"
            # "Currently will only\ncalculate position if 2+ \nbeacons are available \nfrom both cameras"
            # "System is in Normal (long range) State"
            n121 = And(x=w624, y=w623) -> (x .and. y?=w628:bool[])
            "Valid Beacon Sets_" <- w628
            n122 = Boolean To (0,1)(Boolean=w628) -> (0, 1=w625:i16[])
            n123 = Add Array Elements(numeric array=w625) -> (sum=w626:i16)
            n124 = Greater?(x=w626, y=1) -> (0:w622:bool)
            n125 = for {
              N: w607 -> [_]
              tunnel: w622 -> [w689]
              tunnel: w619 -> [w688] mode=indexing
              tunnel: w618 -> [w687] mode=indexing
              tunnel: w620 -> [w686]
              tunnel: "Distance Threshold\nRef Triangles (*unit)" -> [w685]
              tunnel: [w684] -> w605 mode=indexing
              tunnel: [w683] -> _ mode=indexing
              tunnel: [w682] -> w604 mode=indexing
              tunnel: [w681] -> _ mode=indexing
              tunnel: [w680] -> w606 mode=indexing
              tunnel: [w679] -> w613 mode=indexing
              n126 = case shown="True" w689 {
                tunnel: w688 -> [w694 w704]
                tunnel: w687 -> [w693 w703]
                tunnel: w686 -> [_ w695]
                tunnel: w685 -> [_ w696]
                tunnel: [w694 w702] -> w684
                tunnel: [w693 w701] -> w683
                tunnel: [FALSE w700] -> w682
                tunnel: [w691 w699] -> w681
                tunnel: [w691 w698] -> w680
                tunnel: [0 w697] -> w679
                frame False {
                  w691 = sgl 1.0
                }
                frame True {
                  # "Build Reference Triangle"
                  n127 = call "Position Calc_Build Reference Triangle_R1.vi"("A2_in"=w704, "A3_in"=w703, "S1 (Length Between\n Cameras - inches)"=w695, "Distance\nThreshold"=w696) -> ("S2"=w699:sgl, "S3"=w698:sgl, "Direction"=w697:i8, "A2"=w702:sgl, "A3"=w701:sgl, "Accept"=w700:bool)  [unwired: 6 in]
                }
              }
            }
            n128 = for {
              N: w607 -> [_]
              tunnel: w604 -> [w674] mode=indexing
              tunnel: w613 -> [w678] mode=indexing
              tunnel: [w678] -> w615 mode=indexing if=w674
              shift-right: [w677] -> w609
              shift-left: 0 -> [w675]
              # "Only add to array\nif valid distance"
              n129 = Increment(x=w675) -> (x+1=w676:i32)
              n130 = Select(t=w676, s=w674, f=w675) -> (s? t:f=w677:i32)
            }
            n131 = Index Array(array=w615, index=0) -> (element=w616:i32)
            n132 = Equal?(x=w615, y=w616) -> (x = y?=w617:bool[])
            n133 = And Array Elements(Boolean array=w617) -> (logical AND=w611:bool)
            n134 = Greater?(x=w609, y=1) -> (0:w610:bool)
            n135 = And(x=w611, y=w610) -> (x .and. y?=w603:bool)
            n136 = case shown="True" w603 {
              tunnel: w607 -> [w631 w640]
              tunnel: w606 -> [_ w639]
              tunnel: w605 -> [_ w638]
              tunnel: w604 -> [_ w637]
              tunnel: [w630 w636] -> w602
              tunnel: [w629 w635] -> w601
              tunnel: [w629 w634] -> w600
              frame False {
                # "Build Array for False"
                n137 = for {
                  N: w631 -> [_]
                  tunnel: [sgl 0.0] -> w629 mode=indexing
                  tunnel: [FALSE] -> w630 mode=indexing
                }
              }
              frame True {
                n138 = for {
                  N: w640 -> [_]
                  tunnel: w638 -> [w646] mode=indexing
                  tunnel: w639 -> [w645] mode=indexing
                  tunnel: [w644] -> w635 mode=indexing
                  tunnel: [w643] -> w634 mode=indexing
                  tunnel: [w642] -> w636 mode=indexing
                  tunnel: w637 -> [w641] mode=indexing
                  n139 = case shown="True" w641 {
                    selector: w641 -> [w648 w652]
                    tunnel: w646 -> [_ w660]
                    tunnel: [w647 w650] -> w644
                    tunnel: [w647 w651] -> w643
                    tunnel: w645 -> [_ w649]
                    tunnel: [w648 w652] -> w642
                    frame False {
                      w647 = sgl 0.0
                      # "Current Data Set Was Not Valid\nFill with 0\nWill not be used later"
                    }
                    frame True {
                      # "dY"
                      # "dX"
                      # "Negate dX if A2>90"
                      # "Find LOCAL Coordinate of Each Beacon"
                      # "Current - Valid Data Set"
                      n140 = Less?(x=w660, y=sgl 90.0) -> (x < y?=w662:bool)
                      n141 = case shown="False" w662 {
                        tunnel: w660 -> [w669 w671]
                        tunnel: [w667 w672] -> w659
                        tunnel: [FALSE TRUE] -> w654
                        frame False {
                          # "Negative Y"
                          # "A2 is > 90"
                          n142 = Subtract(x=w669, y=sgl 90.0) -> (x-y=w667:sgl)
                        }
                        frame True {
                          # "Positive Y"
                          # "A2 is < 90"
                          n143 = Subtract(x=sgl 90.0, y=w671) -> (x-y=w672:sgl)
                        }
                      }
                      "dA2 4" <- w659
                      n144 = expression code="(x/180.0)*pi" "degrees to radians"(w659) -> (w657:sgl)
                      n145 = expression code="(x/180.0)*pi" "degrees to radians"(w659) -> (w658:sgl)
                      n146 = Cosine(x=w657) -> (cos(x)=w655:sgl)
                      n147 = Sine(x=w658) -> (sin(x)=w656:sgl)
                      n148 = Multiply(x=w649, y=w655) -> (x*y=w651:sgl)
                      n149 = Multiply(x=w649, y=w656) -> (x*y=w653:sgl)
                      n150 = case shown="True" w654 {
                        tunnel: w653 -> [w664 w665]
                        tunnel: [w663 w665] -> w650
                        frame False {
                          n151 = Negate(x=w664) -> (-x=w663:sgl)
                        }
                        frame True {
                        }
                      }
                    }
                  }
                }
              }
            }
          }
        }
        n152 = Boolean To (0,1)(Boolean=w144) -> (0, 1=w143:i16[])
        n153 = Add Array Elements(numeric array=w143) -> (sum=w142:i16)
        n154 = Greater?(x=w142, y=i16 1) -> (0:w140:bool)
        n155 = case shown="True" w140 {
          tunnel: w183 -> [_ w269]
          tunnel: [0.0 ("f") w268] -> w179
          tunnel: [w186 w267] -> w178
          tunnel: w174 -> [_ w266]
          tunnel: w173 -> [_ w265]
          tunnel: [FALSE w264] -> w165
          tunnel: [FALSE w263] -> w164
          tunnel: w162 -> [_ w262]
          tunnel: [sgl 0.0 w260] -> w155
          tunnel: "Distance Between \nCameras  (*unit)" -> [_ w194]
          tunnel: w147 -> [_ w193]
          tunnel: w146 -> [_ w192]
          tunnel: w144 -> [_ w191]
          tunnel: w145 -> [_ w190]
          frame False {
            w185 = 0.0 ("f")
            n156 = Bundle("f"=w185, "f"=w185) -> (w186:cluster{"f":dbl, "f":dbl})  [unwired: 1 in]
          }
          frame True {
            w232 = sgl 2.0
            w249 = 0
            # "Only Apply This Filtering \nif 3 or More Beacons Still Valid"
            # "Orientation Value"
            # "Orientation Valid"
            # "Y (current)"
            # "X (current)"
            # "Number of Valid\nPrevious Orientations"
            # "Position Valid Shift Array"
            # "More than 1 Previous\nValid Positions"
            # "More than\n2previous position\navailable"
            # "Choose Beacon Set\nwith Lowest Std Dev"
            # "Y value cannot be negative"
            # "Find New # Of Valid Beacons"
            # "Adjust/Normalize\nLocal Beacon Positions\nusing Line of Best fit"
            # "# Valid\nData Sets"
            # "cam, y"
            # "cam, x"
            # "Calculate dX and dY\nfor right cam"
            # "Average dX and dY from each (valid) beacon to find position of each camera\n\nthen average all  positions for each camera find center between"
            # "Convert Slope\nto Radians"
            # "*rotate CCW in rad"
            # "Rotate Coordinate\n System by Slope"
            n157 = Boolean To (0,1)(Boolean=w266) -> (0, 1=w216:i16[])
            n158 = Add Array Elements(numeric array=w216) -> (sum=w209:i16)
            n159 = Greater?(x=w209, y=2) -> (0:w210:bool)
            n160 = Bundle(w193, w192) -> (→"LOCAL\nBeacon Coordinates\nRelative to Robot" →"Local Coordinates - Calculated":cluster{sgl[], sgl[]})  [unwired: 1 in]
            n161 = call "Coordinate_Outlier_Filtering_R2.vi"("Num of Beacons"=w190, "Max Std Dev(all 5)"="Max Std Dev (5)", "X in"=w193, "Valid Data\nSets in"=w191, "Y in"=w192, "Max Std Dev( 4 )"="Max Std Dev (4)", "Max Std Dev (3)"="Max Std Dev (3)") -> ("Y out"=w205:sgl[], "X out"=w206:sgl[], "Valid Beacons\nout"=w203:bool[], "Slope out"=w213:dbl)  [unwired: 3 in, 2 out]
            n162 = Inverse Tangent(1:w213) -> (0:w228:dbl)
            n163 = expression code="(x/pi)*180.0" "radians to degrees"(w228) -> (w212:dbl)
            n164 = Boolean To (0,1)(Boolean=w203) -> (0, 1=w202:i16[])
            n165 = To Single Precision Float(number=w212) -> (single precision float=w260:sgl)
            n166 = case shown="True" w210 {
              tunnel: w266 -> [_ w302]
              tunnel: [w279 w289] -> w263
              tunnel: w265 -> [_ w292]
              tunnel: w260 -> [w280 w285]
              tunnel: [w278 w290] -> w268
              tunnel: w262 -> [_ _]
              frame False {
                # "Since no history available,\ncheck that current is with 0-360"
                # "Use Current Orientation bc \nPrevious are not available"
                # "New Position\nValid"
                n167 = In Range and Coerce(upper limit=sgl 360.0, x=w280, lower limit=sgl -360.0 ("upper limit")) -> (In Range?=w279:bool)  [unwired: 1 out]
                n168 = Select(t=w280, s=w279, f=sgl 0.0) -> (s? t:f=w278:sgl)
              }
              frame True {
                # "Moving Average Out"
                # "Valid Position Ccount\n(up to 2)"
                # "Only Calculate MOving Avg\nif xx% of previous positions were valid"
                n169 = Initialize Array(u8 0, "Moving Average\nWindow Length") -> (w298:u8[])
                n170 = local read "History Size"() -> (w299:u8)
                n171 = while {
                  shift-right: [w327] -> w293
                  shift-left: w298 -> [w329]
                  tunnel: w302 -> [w335] mode=indexing
                  shift-right: [w333] -> w287
                  shift-left: u8 0 -> [w336]
                  tunnel: w299 -> [w334]
                  tunnel: "Moving Average\nWindow Length" -> [w326]
                  i -> [w328]
                  stop <- w330 stop-if-true
                  # "Grab Last 2 Valid Position Indexes"
                  n172 = case shown="True" w335 {
                    tunnel: w336 -> [w338 w340]
                    tunnel: [w338 w343] -> w333
                    tunnel: w329 -> [w337 w342]
                    tunnel: w328 -> [_ w341]
                    tunnel: [w337 w339] -> w327
                    frame False {
                    }
                    frame True {
                      # "Update Index\nto use"
                      # "Increment\nValid Count"
                      n173 = Replace Array Subset(array=w342, new element=w341, index=w340) -> (w339:u8[])
                      n174 = Increment(x=w340) -> (x+1=w343:u8)
                    }
                  }
                  n175 = Greater?(x=w328, y=w334) -> (0:w331:bool)
                  n176 = Greater Or Equal?(x=w333, y=w326) -> (x >= y?=w332:bool)
                  n177 = Or(x=w332, y=w331) -> (x .or. y?=w330:bool)
                }
                n178 = for {
                  N: w287 -> [_]
                  shift-right: [w325] -> w296
                  shift-left: 0.0 -> [w324]
                  tunnel: w293 -> [w323] mode=indexing
                  tunnel: w292 -> [w321]
                  # "Fetch Last Valid Values\nand Sum"
                  n179 = Index Array(array=w321, index=w323) -> (element=w322:sgl)
                  n180 = Add(x=w322, y=w324) -> (x+y=w325:dbl)
                }
                n181 = Increment(x=w287) -> (x+1=w284:u8)
                n182 = Add(x=w285, y=w296) -> (x+y=w286:dbl)
                n183 = To Double Precision Float(number=w284) -> (double precision float=w295:dbl)
                n184 = Divide(x=w286, y=w295) -> (x/y=w291:dbl)
                n185 = Greater Than 0?(x=w284) -> (x > 0?=w288:bool)
                n186 = case shown="True" w288 {
                  tunnel: w291 -> [w305 w311]
                  tunnel: w293 -> [_ w318]
                  tunnel: w292 -> [_ w317]
                  tunnel: [w304 w310] -> w290
                  tunnel: [w303 w313] -> w289
                  frame False {
                    # "No Pevious is Available to Compare\ncheck that current is real angle"
                    n187 = In Range and Coerce(upper limit=sgl 360.0, x=w305, lower limit=sgl -360.0 ("upper limit")) -> (In Range?=w303:bool)  [unwired: 1 out]
                    n188 = Select(t=w305, s=w303, f=sgl 0.0) -> (s? t:f=w304:dbl)
                  }
                  frame True {
                    # "Calculate New, Weighted\nOrientation"
                    # "Check That New Value\nis within Range of Old\n(avg)"
                    # "(X1 - X2)^2"
                    # "Previous"
                    # "Pevious is Available to Compare"
                    n189 = Index Array(array=w318, index=u8 0) -> (element=w319:u8)
                    n190 = Index Array(array=w317, index=w319) -> (element=w316:sgl)
                    n191 = Subtract(x=w316, y=w311) -> (x-y=w315:dbl)
                    n192 = Absolute Value(x=w315) -> (abs(x)=w314:dbl)
                    n193 = Less Or Equal?(x=w314, y="New Orientation \nThreshold") -> (x <= y?=w313:bool)
                    n194 = Select(t=w311, s=w313, f=sgl 0.0) -> (s? t:f=w310:dbl)
                  }
                }
              }
            }
            n195 = Add Array Elements(numeric array=w202) -> (sum=w201:i16)
            n196 = Greater?(x=w201, y=i16 2) -> (0:w199:bool)
            n197 = case shown="True" w199 {
              tunnel: w190 -> [_ w277]
              tunnel: w203 -> [w270 w276]
              tunnel: w206 -> [_ w275]
              tunnel: w205 -> [_ w274]
              tunnel: [w270 w273] -> w204
              tunnel: "Distance\nBetween Beacons" -> [_ w272]
              tunnel: "Distance\nBetween Beacons \n- Tolerance" -> [_ w271]
              frame False {
                # "Don't apply filtering,\nnot enough data points"
              }
              frame True {
                # "This will filter beacons if they are calculate to be \ntoo close to each other. The beacon(s) that is\n discarded is chosen based distance between each/every\nbeacon,. Capable of filtering as long as 1/2 of sample\nset has uniform distances (between beacons)."
                # "Validate Distance Between\nEach Beacon"
                n198 = call "Beacon_Filtering_Inter_Beacon_Distance_R1.vi"("Num of Beacons"=w277, "Inter Beacon\nReal Distance"=w272, "X in"=w275, "Inter Beacon\ndelta Threshold"=w271, "Y in"=w274, "Valid Data\nSets in"=w276) -> ("Beacons Valid - Out"=w273:bool[])  [unwired: 9 in]
              }
            }
            "Post Filtering\n- Valid Beacons" <- w204
            n199 = Increment(x=w190) -> (x+1=w250:i8)
            n200 = for {
              N: w250 -> [_]
              tunnel: [w474] -> w251 mode=indexing
              tunnel: w206 -> [w470]
              tunnel: w205 -> [w473]
              tunnel: [w472] -> w252 mode=indexing
              tunnel: w194 -> [w469]
              i -> [w471]
              # "Build Array's of Coordinates\nFor All Objects"
              n201 = Greater Than 0?(x=w471) -> (x > 0?=w475:bool)
              n202 = case shown="True" w475 {
                tunnel: [w477 w483] -> w474
                tunnel: w470 -> [w480 _]
                tunnel: w473 -> [w479 _]
                tunnel: [w476 0.0] -> w472
                tunnel: w471 -> [w481 _]
                tunnel: w469 -> [_ w483]
                frame True {
                  # "Rest of Array is\nBeacon Coordinates"
                  n203 = Decrement(x=w481) -> (x-1=w478:i32)
                  n204 = Index Array(array=w480, index=w478) -> (element=w477:sgl)
                  n205 = Index Array(array=w479, index=w478) -> (element=w476:sgl)
                }
                frame False {
                  # "First object is the\nother Camera\n\nthis coordinate\nis simply:\nx = 0\ny = distance btween cams"
                }
              }
            }
            n206 = Bundle(w251, w252) -> (→"All Object Coordinates \n- Local" →"Local Coordinates - Normalized":cluster{sgl[], dbl[]})  [unwired: 1 in]
            n207 = expression code="(x/180.0)*pi" "degrees to radians"(w268) -> (w211:dbl)
            n208 = call-poly <vilib>:"2D Cartesian Coordinate Rotation.vi"("theta"=w211, "Y"=w252, "X"=w251) -> ("Y Out"=w229:dbl[], "X Out"=w230:dbl[])  [unwired: 6 in, 1 out]
            n209 = Bundle("X Out"=w230, "Y Out"=w229) -> (→"All Object Coordinates \n- Local - Rotated" →"Local Coordinates - Rotated":cluster{"X Out":dbl[], "Y Out":dbl[]})  [unwired: 1 in]
            n210 = Index Array(array=w229, index=w249) -> (element=w225:dbl)
            n211 = Index Array(array=w230, index=w249) -> (element=w248:dbl)
            n212 = for {
              N: w190 -> [_]
              tunnel: w229 -> [w465]
              tunnel: w230 -> [w466]
              tunnel: w248 -> [w464]
              tunnel: w225 -> [w463]
              tunnel: [w462] -> w222 mode=indexing
              tunnel: [w461] -> w221 mode=indexing
              tunnel: [w460] -> w196 mode=indexing
              tunnel: [w459] -> w223 mode=indexing
              i -> [w468]
              n213 = Increment(x=w468) -> (x+1=w467:i32)
              n214 = Index Array(array=w465, index=w467) -> (element=w459:dbl)
              n215 = Index Array(array=w466, index=w467) -> (element=w460:dbl)
              n216 = Subtract(x=w459, y=w463) -> (x-y=w461:dbl)
              n217 = Subtract(x=w460, y=w464) -> (x-y=w462:dbl)
            }
            n218 = Bundle(w222, w221) -> (→"dX, dY\nRight Cam":cluster{dbl[], dbl[]})  [unwired: 1 in]
            n219 = Bundle(w196, w223) -> (→"dX, dY\nLeft Cam":cluster{dbl[], dbl[]})  [unwired: 1 in]
            n220 = Unbundle("Real Beacon\n - Coordinates") -> ("X"=w246:dbl[], "Y"=w226:dbl[])
            n221 = Boolean To (0,1)(Boolean=w204) -> (0, 1=w224:i16[])
            n222 = for {
              N: w190 -> [_]
              tunnel: w204 -> [w445] mode=indexing
              tunnel: w246 -> [w442] mode=indexing
              tunnel: w226 -> [w441] mode=indexing
              tunnel: w196 -> [w444] mode=indexing
              tunnel: w223 -> [w440] mode=indexing
              tunnel: w222 -> [w443] mode=indexing
              tunnel: w221 -> [w439] mode=indexing
              tunnel: [w438] -> w245 mode=indexing
              tunnel: [w437] -> w244 mode=indexing
              tunnel: [w436] -> w243 mode=indexing
              tunnel: [w435] -> w242 mode=indexing
              n223 = case shown="True" w445 {
                tunnel: w444 -> [_ w458]
                tunnel: w443 -> [_ w457]
                tunnel: w442 -> [_ w448]
                tunnel: w441 -> [_ w447]
                tunnel: w440 -> [_ w456]
                tunnel: w439 -> [_ w449]
                tunnel: [w446 w454] -> w438
                tunnel: [w446 w453] -> w437
                tunnel: [w446 w452] -> w436
                tunnel: [w446 w451] -> w435
                frame False {
                  w446 = sgl 0.0
                  # "Add Nothing"
                }
                frame True {
                  # "realX = beaconX + dY\nrealY = beaconY + (-dx)"
                  # "Right Cam"
                  # "Left Cam"
                  # "dX = -dX\nSwap dX, dY"
                  # "Translate to Real Coordinates\nOnly Apply for Valid Beacons"
                  n224 = Negate(x=w458) -> (-x=w455:dbl)
                  n225 = Negate(x=w457) -> (-x=w450:dbl)
                  n226 = Add(x=w448, y=w456) -> (x+y=w454:dbl)
                  n227 = Add(x=w447, y=w455) -> (x+y=w453:dbl)
                  n228 = Add(x=w448, y=w449) -> (x+y=w452:dbl)
                  n229 = Add(x=w447, y=w450) -> (x+y=w451:dbl)
                }
              }
            }
            n230 = Add Array Elements(numeric array=w224) -> (sum=w227:i16)
            n231 = Add Array Elements(numeric array=w245) -> (sum=w241:dbl)
            n232 = Add Array Elements(numeric array=w244) -> (sum=w240:dbl)
            n233 = Add Array Elements(numeric array=w243) -> (sum=w239:dbl)
            n234 = Add Array Elements(numeric array=w242) -> (sum=w238:dbl)
            n235 = Divide(x=w241, y=w227) -> (x/y=w237:dbl)
            n236 = Divide(x=w240, y=w227) -> (x/y=w235:dbl)
            n237 = Divide(x=w239, y=w227) -> (x/y=w236:dbl)
            n238 = Divide(x=w238, y=w227) -> (x/y=w234:dbl)
            n239 = Bundle(w237, w235) -> (→"Left Camera Real Coordinates":cluster{dbl, dbl})  [unwired: 1 in]
            n240 = Bundle(w236, w234) -> (→"Right Camera Real Coordinate":cluster{dbl, dbl})  [unwired: 1 in]
            n241 = Add(x=w237, y=w236) -> (x+y=w233:dbl)
            n242 = Add(x=w235, y=w234) -> (x+y=w231:dbl)
            n243 = local read "Moving Average\nWindow Length"() -> (w195:u8)
            n244 = Divide(x=w233, y=w232) -> (x/y=w215:dbl)
            n245 = Divide(x=w231, y=w232) -> (x/y=w214:dbl)
            n246 = case shown="True" w210 {
              tunnel: w266 -> [_ w380]
              tunnel: w209 -> [_ _]
              tunnel: w215 -> [w348 w358]
              tunnel: [w349 w371] -> w264
              tunnel: w269 -> [_ w355]
              tunnel: w214 -> [w347 w357]
              tunnel: [w346 w379] -> w267
              tunnel: "Max X (arena)" -> [w345 w370]
              tunnel: "Max Y (arena)" -> [w344 w369]
              tunnel: w195 -> [_ w361]
              frame False {
                # "New Position\nValid"
                # "Since no history available,\ncheck that current is within\nthe bounds of the arena size"
                # "Use Current Position bc \nPrevious are not available"
                n247 = In Range and Coerce(upper limit=w345, x=w348, lower limit=sgl 0.0 ("upper limit")) -> (In Range?=w351:bool)  [unwired: 1 out]
                n248 = In Range and Coerce(upper limit=w344, x=w347, lower limit=sgl 0.0 ("upper limit")) -> (In Range?=w350:bool)  [unwired: 1 out]
                n249 = Bundle(w348, w347) -> (w346:cluster{dbl, dbl})  [unwired: 1 in]
                n250 = And(x=w351, y=w350) -> (x .and. y?=w349:bool)
              }
              frame True {
                w368 = 0.0
                # "If needed, make seperate FOR Loop for \nY only... Using more previous values than X"
                # "New Y"
                # "New X"
                # "Only consider if velocity is\ngreater than certain speed"
                # "Valid Position Ccount\n(up to 2)"
                # "Weighted Robot \nCoordinates"
                # "Position\nValid\n(current)"
                # "Only Calculate MOving Avg\nif xx% of previous positions were valid"
                n251 = Initialize Array(u8 0, w361) -> (w375:u8[])
                n252 = local read "History Size"() -> (w376:u8)
                n253 = while {
                  shift-right: [w419] -> w356
                  shift-left: w375 -> [w421]
                  tunnel: w380 -> [w426] mode=indexing
                  shift-right: [w424] -> w367
                  shift-left: u8 0 -> [w427]
                  tunnel: w376 -> [w425]
                  tunnel: [w418] -> _
                  tunnel: w361 -> [w417]
                  i -> [w420]
                  stop <- w422 stop-if-true
                  # "Grab Last 3 Valid Position Indexes"
                  n254 = case shown="True" w426 {
                    tunnel: w427 -> [w429 w431]
                    tunnel: [w429 w434] -> w424
                    tunnel: w421 -> [w428 w433]
                    tunnel: w420 -> [_ w432]
                    tunnel: [w428 w430] -> w419
                    frame False {
                    }
                    frame True {
                      # "Update Index\nto use"
                      # "Increment\nValid Count"
                      n255 = Replace Array Subset(array=w433, new element=w432, index=w431) -> (w430:u8[])
                      n256 = Increment(x=w431) -> (x+1=w434:u8)
                    }
                  }
                  n257 = Greater?(x=w420, y=w425) -> (0:w423:bool)
                  n258 = Greater Or Equal?(x=w424, y=w417) -> (x >= y?=w418:bool)
                  n259 = Or(x=w418, y=w423) -> (x .or. y?=w422:bool)
                }
                n260 = for {
                  N: w367 -> [_]
                  shift-right: [w389] -> w365
                  shift-left: w368 -> [w388]
                  shift-right: [w387] -> w364
                  shift-left: w368 -> [w386]
                  tunnel: w356 -> [w384] mode=indexing
                  tunnel: w355 -> [w382]
                  # "Fetch Last Valid Values\nand Sum"
                  n261 = Index Array(array=w382, index=w384) -> (element=w383:cluster{sgl, sgl})
                  n262 = Unbundle(w383) -> (w385:sgl, w381:sgl)
                  n263 = Add(x=w381, y=w386) -> (x+y=w387:dbl)
                  n264 = Add(x=w385, y=w388) -> (x+y=w389:dbl)
                }
                n265 = Increment(x=w367) -> (x+1=w354:u8)
                n266 = Add(x=w358, y=w365) -> (x+y=w360:dbl)
                n267 = To Single Precision Float(number=w354) -> (single precision float=w366:sgl)
                n268 = Add(x=w357, y=w364) -> (x+y=w359:dbl)
                n269 = Divide(x=w360, y=w366) -> (x/y=w363:dbl)
                n270 = Divide(x=w359, y=w366) -> (x/y=w362:dbl)
                n271 = Greater Than 0?(x=w354) -> (x > 0?=w374:bool)
                n272 = case shown="True" w374 {
                  tunnel: w363 -> [w394 w401]
                  tunnel: w362 -> [w393 w400]
                  tunnel: w356 -> [_ w413]
                  tunnel: w355 -> [_ w412]
                  tunnel: [w391 w401] -> w373
                  tunnel: [w390 w400] -> w372
                  tunnel: [w395 w402] -> w371
                  tunnel: w370 -> [w397 _]
                  tunnel: w369 -> [w396 _]
                  frame False {
                    w392 = sgl 0.0 ("upper limit")
                    # "Check that within bounds of arena"
                    # "No Pevious is Available to Compare"
                    n273 = In Range and Coerce(upper limit=w397, x=w394, lower limit=w392) -> (In Range?=w399:bool)  [unwired: 1 out]
                    n274 = In Range and Coerce(upper limit=w396, x=w393, lower limit=w392) -> (In Range?=w398:bool)  [unwired: 1 out]
                    n275 = And(x=w399, y=w398) -> (x .and. y?=w395:bool)
                    n276 = Select(t=w394, s=w395, f=w392) -> (s? t:f=w391:dbl)
                    n277 = Select(t=w393, s=w395, f=w392) -> (s? t:f=w390:dbl)
                  }
                  frame True {
                    # "New"
                    # "(Y1 - Y2)^2"
                    # "(X1 - X2)^2"
                    # "Previous"
                    # "Pevious is Available to Compare"
                    n278 = Index Array(array=w413, index=u8 0) -> (element=w415:u8)
                    n279 = Index Array(array=w412, index=w415) -> (element=w414:cluster{sgl, sgl})
                    n280 = Unbundle(w414) -> (w404:sgl, w403:sgl)
                    n281 = Subtract(x=w404, y=w401) -> (x-y=w409:dbl)
                    n282 = Subtract(x=w400, y=w403) -> (x-y=w408:dbl)
                    n283 = Square(x=w409) -> (x^2=w407:dbl)
                    n284 = Square(x=w408) -> (x^2=w406:dbl)
                    n285 = Add(x=w407, y=w406) -> (x+y=w410:dbl)
                    n286 = Square Root(x=w410) -> (sqrt(x)=w405:dbl)
                    n287 = Less Or Equal?(x=w405, y="New Position \nThreshold") -> (x <= y?=w402:bool)
                  }
                }
                n288 = Bundle("upper limit"=w373, "upper limit"=w372) -> (w379:cluster{"upper limit":dbl, "upper limit":dbl})  [unwired: 1 in]
              }
            }
            n289 = Bundle(w215, w214) -> (→"Robot Coordinates":cluster{dbl, dbl})  [unwired: 1 in]
            n290 = Less Than 0?(x=w214) -> ()  [unwired: 1 out]
          }
        }
        "Orietnation\n(current)" <- w155
        n291 = And(x=w165, y=w164) -> (x .and. y?=w168:bool)
        "Position Valid" <- w168
        n292 = Exclusive Or(1:w164, 2:w165) -> (0:w163:bool)
        n293 = case shown="True" w168 {
          tunnel: [w711 w714] -> w131
          tunnel: [w712 w713] -> w133
          tunnel: w179 -> [_ w714]
          tunnel: w178 -> [_ w713]
          tunnel: w163 -> [_ _]
          frame False {
            w711 = sgl 0.0 ("f")
            n294 = Bundle("f"=w711, "f"=w711) -> (w712:cluster{"f":sgl, "f":sgl})  [unwired: 1 in]
          }
          frame True {
            # "For Servos"
            "Last Orientation" <- w714
            "Last Position" <- w713
          }
        }
        "Robot Coordinates - Avgd" <- w133
        "Orientation Avgd" <- w131
        n295 = local read "History Size"() -> (w157:u8)
        n296 = Decrement(x=w157) -> (x-1=w158:u8)
        n297 = for {
          N: w157 -> [_]
          shift-right: [w752] -> w181
          shift-left: w177 -> [w751]
          tunnel: w133 -> [w750]
          tunnel: w158 -> [w749]
          i -> [w748]
          n298 = Subtract(x=w749, y=w748) -> (x-y=w747:i32)
          n299 = Equal To 0?(x=w747) -> (x = 0?=w746:bool)
          n300 = case shown="False" w746 {
            tunnel: w747 -> [w754 w759]
            tunnel: w751 -> [w757 w760]
            tunnel: [w755 w761] -> w752
            tunnel: w750 -> [_ w758]
            frame False {
              n301 = Decrement(x=w754) -> (x-1=w753:i32)
              n302 = Index Array(array=w757, index=w753) -> (element=w756:cluster{sgl, sgl})
              n303 = Replace Array Subset(array=w757, new element=w756, index=w754) -> (w755:cluster{sgl, sgl}[])
            }
            frame True {
              n304 = Replace Array Subset(array=w760, new element=w758, index=w759) -> (w761:cluster{sgl, sgl}[])
            }
          }
        }
        n305 = Decrement(x=w157) -> (x-1=w159:u8)
        n306 = for {
          N: w157 -> [_]
          shift-right: [w736] -> w182
          shift-left: w176 -> [w735]
          tunnel: w131 -> [w734]
          tunnel: w159 -> [w733]
          i -> [w732]
          n307 = Subtract(x=w733, y=w732) -> (x-y=w730:i32)
          n308 = Equal To 0?(x=w730) -> (x = 0?=w731:bool)
          n309 = case shown="False" w731 {
            tunnel: w730 -> [w738 w743]
            tunnel: w735 -> [w741 w744]
            tunnel: [w739 w745] -> w736
            tunnel: w734 -> [_ w742]
            frame False {
              # "Shift"
              n310 = Decrement(x=w738) -> (x-1=w737:i32)
              n311 = Index Array(array=w741, index=w737) -> (element=w740:sgl)
              n312 = Replace Array Subset(array=w741, new element=w740, index=w738) -> (w739:sgl[])
            }
            frame True {
              # "insert new"
              n313 = Replace Array Subset(array=w744, new element=w742, index=w743) -> (w745:sgl[])
            }
          }
        }
        n314 = Decrement(x=w157) -> (x-1=w156:u8)
        n315 = for {
          N: w157 -> [_]
          shift-right: [w721] -> w180
          shift-left: w175 -> [w720]
          tunnel: w168 -> [w719]
          tunnel: w156 -> [w718]
          i -> [w717]
          n316 = Subtract(x=w718, y=w717) -> (x-y=w715:i32)
          n317 = Equal To 0?(x=w715) -> (x = 0?=w716:bool)
          n318 = case shown="False" w716 {
            tunnel: w720 -> [w726 w728]
            tunnel: [w724 w729] -> w721
            tunnel: w719 -> [_ w727]
            tunnel: w715 -> [w722 _]
            frame False {
              n319 = Decrement(x=w722) -> (x-1=w723:i32)
              n320 = Index Array(array=w726, index=w723) -> (element=w725:bool)
              n321 = Replace Array Subset(array=w726, new element=w725, index=w722) -> (w724:bool[])
            }
            frame True {
              n322 = Replace Array Subset(array=w728, new element=w727) -> (w729:bool[])  [unwired: 1 in]
            }
          }
        }
        n323 = Boolean To (0,1)(Boolean=w180) -> (0, 1=w172:i16[])
        n324 = Add Array Elements(numeric array=w172) -> (sum=w170:i16)
        n325 = Greater Or Equal?(x=w170, y=i16 2) -> (x >= y?=→"Position \nLock Status":bool)
        n326 = case shown="True" w168 {
          tunnel: w133 -> [_ w710]
          frame False {
          }
          frame True {
            # "update debug graph\nif current is valid"
            n327 = Unbundle(w710) -> ("upper limit"=w709:dbl, "upper limit"=w708:dbl)
            n328 = Build Array(w708) -> (w706:dbl[])
            n329 = Build Array(w709) -> (w707:dbl[])
            n330 = Bundle(w707, w706) -> (→"Real Position in Course 2":cluster{dbl[], dbl[]})  [unwired: 1 in]
          }
        }
        n331 = Unbundle(w133) -> ("upper limit"=w132:dbl, "upper limit"=w130:dbl)
        n332 = shared-variable "RT myRIO Target - Overlord\\Localization_Variables_r0.lvlib\\loc_x"(w132) -> ()  [unwired: 1 in, 1 out]
        n333 = shared-variable "RT myRIO Target - Overlord\\Localization_Variables_r0.lvlib\\loc_y"(w130) -> ()  [unwired: 1 in, 1 out]
        n334 = shared-variable "RT myRIO Target - Overlord\\Localization_Variables_r0.lvlib\\loc_theta"(w131) -> ()  [unwired: 1 in, 1 out]
      }
    }
    n335 = case shown="True" w113 {
      tunnel: w112 -> [_ w120]
      frame False {
      }
      frame True {
        n336 = call "Tick Count3"() -> ("Tick Count(uSec)"=w121:u32)
        n337 = Subtract(x=w121, y=w120) -> (x-y=w124:u32)
        n338 = Divide(x=w124, y=u32 1000 ("x")) -> (x/y=→"dT":dbl)
      }
    }
    n339 = call "Tick Count6"() -> ("Tick Count(uSec)"=w110:u32)
    "Robot Coordinates\nHistory" <- w109
    "Orientation\nHistory" <- w114
    "Position Valid\nHistory" <- w115
  }
  n340 = disable-structure shown="Enabled" {
    disable-tunnel: [w764 _] -> _
    disable-tunnel: ["Search Step Size\n(deg)" _] -> _
    frame Enabled {
      n341 = Multiply(x=3.413333333333333, y="Search Step Size\n(deg)") -> (x*y=w762:dbl)
      n342 = To Unsigned Word Integer(number=w762) -> (unsigned 16bit integer=w764:u16)
    }
    frame Disabled {
    }
  }
  n343 = Multiply(x="Move Servo\nThreshold (deg)", y=3.413333333333333) -> (x*y=w18:dbl)
  n344 = To Unsigned Word Integer(number=w18) -> ()  [unwired: 1 out]
  n345 = call "Tick Count8"() -> ()  [unwired: 1 out]
  n346 = flat-sequence {
    tunnel: [w768] -> w42
    tunnel: [w767] -> w41
    tunnel: [w772] -> w40
    tunnel: ["Left Servo\nID"] -> w29
    tunnel: ["Right Servo\nID"] -> w28
    tunnel: ["Compliance Slope"] -> w27
    tunnel: [w812] -> w39
    tunnel: [w811] -> w38
    tunnel: w42 -> [w810]
    tunnel: w41 -> [w809]
    tunnel: w40 -> [w808]
    tunnel: w29 -> [w806]
    tunnel: w28 -> [w805]
    tunnel: w27 -> [w804]
    tunnel: w39 -> [w1085]
    tunnel: w38 -> [w1084]
    frame #0 {
      # "BAUD RATE"
      # "Initialize UART and DIO"
      n347 = call-poly "VISA Configure Serial Port"("VISA resource name"=refnum<visa-resource-name> "ASRL1::INSTR", "Enable Termination\nChar (T)"=FALSE ("Enable Termination\nChar (T)"), "baud rate (9600)"=u32 115200) -> ("VISA resource name out"=w768:refnum<visa-resource-name>)  [unwired: 11 in, 1 out]
      n348 = call <vilib>:"Smart Open.vi"("Channel Names"=tag[] ["A/DIO2"]) -> ("DIO Ref Out"=w767:T8)  [unwired: 9 in, 1 out]
      n349 = flat-sequence {
        tunnel: w768 -> [w780]
        tunnel: w767 -> [w779]
        tunnel: "Left Servo\nID" -> [w781]
        tunnel: [w778] -> w769
        tunnel: "Compliance Slope" -> [w777]
        tunnel: "Right Servo\nID" -> [w794]
        tunnel: w769 -> [w793]
        tunnel: "Compliance Slope" -> [w792]
        tunnel: w768 -> [w791]
        tunnel: w767 -> [w790]
        frame #0 {
          w778 = 3
          n350 = while {
            tunnel: w778 -> [w787]
            tunnel: w780 -> [w785]
            tunnel: w779 -> [w784]
            tunnel: w781 -> [w783]
            tunnel: w777 -> [w782]
            i -> [w788]
            stop <- w786 stop-if-true
            n351 = call "Set_Compliance_Slope_R2.vi"("Compliance Slope"=w782, "DIO Ref Out"=w784, "VISA resource name"=w785, "Servo ID"=w783) -> ()  [unwired: 6 in, 2 out]
            n352 = Increment(x=w788) -> (x+1=w789:i32)
            n353 = Greater Or Equal?(x=w789, y=w787) -> (x >= y?=w786:bool)
          }
        }
        frame #1 {
          n354 = while {
            tunnel: w793 -> [w800]
            tunnel: w794 -> [w798]
            tunnel: w791 -> [w797]
            tunnel: w790 -> [w796]
            tunnel: w792 -> [w795]
            i -> [w801]
            stop <- w799 stop-if-true
            n355 = call "Set_Compliance_Slope_R2.vi"("Compliance Slope"=w795, "DIO Ref Out"=w796, "VISA resource name"=w797, "Servo ID"=w798) -> ()  [unwired: 6 in, 2 out]
            n356 = Increment(x=w801) -> (x+1=w802:i32)
            n357 = Greater Or Equal?(x=w802, y=w800) -> (x >= y?=w799:bool)
          }
        }
      }
      n358 = call "Tick Count"() -> ("Tick Count(uSec)"=w772:u32)
    }
    frame #1 {
      # "Service Count"
      n359 = while {
        shift-right: [w815] -> _
        shift-left: w808 -> [w832]
        tunnel: "Max Write\nTx Attempts" -> [w827]
        tunnel: "Max Read\nTx Attempts" -> [w826]
        shift-right: [w822] -> w812
        shift-left: w810 -> [w825]
        shift-right: [w821] -> w811
        shift-left: w809 -> [w824]
        tunnel: w806 -> [w820]
        tunnel: w805 -> [w819]
        tunnel: w804 -> [w818]
        shift-right: [w816] -> _
        shift-left: u16 0 -> [w817]
        stop <- "close comms" stop-if-true
        # "Loop Timer"
        n360 = local read "SERVO ENABLE"() -> (w814:bool)
        n361 = call "Tick Count2"() -> ("Tick Count(uSec)"=w815:u32)
        n362 = Subtract(x=w815, y=w832) -> (x-y=w831:u32)
        n363 = call "Wait4"("Count(mSec)"="Servo Comm\nLoop Time (ms)") -> ()  [unwired: 1 out]
        n364 = Divide(x=w831, y=u32 1000) -> (x/y=→"dT - Comm Loop":dbl)
        n365 = case shown="True" w814 {
          tunnel: w827 -> [_ w841]
          tunnel: w826 -> [_ w872]
          tunnel: w825 -> [w835 w836]
          tunnel: w824 -> [w834 w865]
          tunnel: [w835 w838] -> w822
          tunnel: [w834 w837] -> w821
          tunnel: w820 -> [_ w844]
          tunnel: w819 -> [_ w843]
          tunnel: w818 -> [_ w842]
          tunnel: w817 -> [_ w840]
          tunnel: [u16 100 w839] -> w816
          frame False {
            # "Restart at same value\nUsed to Periodically update \nCompliance Slope"
          }
          frame True {
            n366 = flat-sequence {
              tunnel: [w878] -> w876
              tunnel: [w879] -> w875
              tunnel: [w877] -> w874
              tunnel: w872 -> [w880]
              tunnel: [w882] -> w863
              tunnel: [w881] -> w861
              tunnel: w836 -> [w882]
              tunnel: w865 -> [w881]
              tunnel: w844 -> [w877]
              tunnel: w876 -> [w900]
              tunnel: w875 -> [w901]
              tunnel: w874 -> [w899]
              tunnel: [w899] -> w873
              tunnel: [w898] -> w866
              tunnel: [w897] -> w864
              tunnel: w863 -> [w897]
              tunnel: [w896] -> w862
              tunnel: w861 -> [w896]
              tunnel: w873 -> [w922]
              tunnel: w841 -> [w921]
              tunnel: w866 -> [w916]
              tunnel: w864 -> [w918]
              tunnel: w862 -> [w917]
              tunnel: [w918] -> w859
              tunnel: [w917] -> w857
              tunnel: [w955] -> w860
              tunnel: w859 -> [w955]
              tunnel: [w954] -> w858
              tunnel: w857 -> [w954]
              tunnel: ["Servo Comm\nWait Time - (ms)"] -> w849
              tunnel: w872 -> [w962]
              tunnel: [w961] -> w871
              tunnel: [w960] -> w870
              tunnel: [w956] -> w868
              tunnel: w860 -> [w959]
              tunnel: w858 -> [w958]
              tunnel: [w959] -> w856
              tunnel: [w958] -> w853
              tunnel: [w957] -> w850
              tunnel: w849 -> [w957]
              tunnel: w843 -> [w956]
              tunnel: w871 -> [w982]
              tunnel: w870 -> [w981]
              tunnel: [w980] -> w869
              tunnel: w868 -> [w980]
              tunnel: [w979] -> w867
              tunnel: w856 -> [w978]
              tunnel: [w978] -> w855
              tunnel: [w977] -> w854
              tunnel: w853 -> [w977]
              tunnel: w850 -> [w976]
              tunnel: [w976] -> w848
              tunnel: w869 -> [w1004]
              tunnel: w867 -> [w1002]
              tunnel: w841 -> [w1003]
              tunnel: w855 -> [w1001]
              tunnel: w854 -> [w1000]
              tunnel: [w1001] -> w852
              tunnel: [w1000] -> w851
              tunnel: w848 -> [w997]
              tunnel: [w997] -> w847
              tunnel: w852 -> [w1037]
              tunnel: w851 -> [w1036]
              tunnel: w847 -> [w1035]
              tunnel: [w1037] -> w846
              tunnel: [w1036] -> w845
              tunnel: w846 -> [w1041]
              tunnel: w845 -> [w1040]
              tunnel: w844 -> [w1046]
              tunnel: w843 -> [w1045]
              tunnel: w842 -> [w1044]
              tunnel: w840 -> [w1039]
              tunnel: w841 -> [w1043]
              tunnel: [w1042] -> w839
              tunnel: [w1041] -> w838
              tunnel: [w1040] -> w837
              frame #0 {
                n367 = while {
                  tunnel: [w895] -> w878
                  tunnel: w877 -> [w894]
                  tunnel: [w887] -> w879
                  tunnel: w880 -> [w885]
                  tunnel: w882 -> [w884]
                  tunnel: w881 -> [w883]
                  i -> [w886]
                  stop <- w888 stop-if-true
                  # "Attemp to Read Until\nMax Read Tx Attemps Limit"
                  n368 = call "ReadServo_R3.vi"("DIO Ref In"=w883, "VISA resource name out"=w884, "Servo ID"=w894) -> ("Error"=w891:u8, "Valid Checksum"=w892:bool, "Current Position"=w895:u64)  [unwired: 6 in]
                  n369 = Increment(x=w886) -> (x+1=w889:i32)
                  n370 = Equal To 0?(x=w891) -> (x = 0?=w893:bool)
                  n371 = Greater Or Equal?(x=w889, y=w885) -> (x >= y?=w890:bool)
                  n372 = And(x=w892, y=w893) -> (x .and. y?=w887:bool)
                  n373 = Or(x=w887, y=w890) -> (x .or. y?=w888:bool)
                }
              }
              frame #1 {
                # "Read Position First"
                n374 = local read "Servo Goal Position\n - Left"() -> (w898:u16)
                n375 = case shown="True" w901 {
                  tunnel: w900 -> [_ w906]
                  tunnel: w898 -> [_ w904]
                  frame False {
                  }
                  frame True {
                    # "Convert Received Position to Angle Relative to Robot"
                    # "45 DEG MOUNT OFFSET"
                    # "1024/300"
                    n376 = local write "Current L (10bit)"(w906) -> ()
                    n377 = To Word Integer(number=w906) -> (16bit integer=w910:i16)
                    n378 = To Word Integer(number=w904) -> (16bit integer=w909:i16)
                    n379 = Subtract(x=w909, y=w910) -> (x-y=w908:i16)
                    n380 = Divide(x=w906, y=3.413333333333333) -> (x/y=w914:dbl)
                    n381 = Absolute Value(x=w908) -> (abs(x)=w907:i16)
                    n382 = Subtract(x=w914, y=sgl 60.0) -> (x-y=w912:dbl)
                    n383 = Greater?(x=w907, y=u16 5) -> (0:w903:bool)
                    n384 = Add(x=w912, y=sgl 45.0) -> (x+y=w902:dbl)
                    n385 = local write "Move Servo - L"(w903) -> ()
                    n386 = local write "Servo Moving - L"(w903) -> ()
                    n387 = local write "Current Angle\n - Left (internal)"(w902) -> ()
                    n388 = shared-variable "RT myRIO Target - Overlord\\Localization_Variables_r0.lvlib\\Left Servo Angle_Current"(w902) -> ()  [unwired: 1 in, 1 out]
                  }
                }
              }
              frame #2 {
                n389 = local read "Move Servo - L"() -> (w919:bool)
                n390 = case shown="True" w919 {
                  tunnel: w922 -> [_ w937]
                  tunnel: w916 -> [_ w924]
                  tunnel: [TRUE w935] -> w920
                  tunnel: w921 -> [_ w927]
                  tunnel: w918 -> [_ w926]
                  tunnel: w917 -> [_ w925]
                  frame False {
                    # "Only Send if Current Position is far enough"
                  }
                  frame True {
                    w933 = 1
                    # "High Byte"
                    # "Low Byte"
                    n391 = Type Cast(type="", x=w924) -> (*(type *) &x=w934:string)
                    n392 = local write "Servo Moving - L"(TRUE) -> ()
                    n393 = String Subset(string=w934, offset (0)=1, length (rest)=w933) -> (substring=w929:string)
                    n394 = String Subset(string=w934, offset (0)=0, length (rest)=w933) -> (substring=w928:string)
                    n395 = while {
                      tunnel: w937 -> [w951]
                      tunnel: [w943] -> w935
                      tunnel: w929 -> [w947]
                      tunnel: w928 -> [w946]
                      tunnel: w927 -> [w940]
                      tunnel: w926 -> [w939]
                      tunnel: w925 -> [w938]
                      i -> [w941]
                      stop <- w942 stop-if-true
                      # "Attemp to Write Until\nMax Write Tx Attemps Limit"
                      n396 = call "MoveServo_R3.vi"("DIO Ref Out"=w938, "VISA resource name out"=w939, "GP - Low Byte"=w947, "GP - High Byte"=w946, "Servo ID"=w951) -> ("Valid Checksum"=w948:bool, "Error"=w950:u64)  [unwired: 5 in]
                      n397 = Equal To 0?(x=w950) -> (x = 0?=w949:bool)
                      n398 = And(x=w948, y=w949) -> (x .and. y?=w943:bool)
                      n399 = Increment(x=w941) -> (x+1=w945:i32)
                      n400 = Greater Or Equal?(x=w945, y=w940) -> (x >= y?=w944:bool)
                      n401 = Or(x=w943, y=w944) -> (x .or. y?=w942:bool)
                    }
                  }
                }
                n402 = case shown="True" w920 {
                  frame False {
                  }
                  frame True {
                    # "Update Servo flag"
                    n403 = local write "Move Servo - L"(FALSE) -> ()
                  }
                }
              }
              frame #3 {
                n404 = call "Wait2"("Count(mSec)"="Servo Comm\nWait Time - (ms)") -> ()  [unwired: 1 out]
              }
              frame #4 {
                n405 = while {
                  tunnel: [w975] -> w961
                  tunnel: w956 -> [w974]
                  tunnel: [w967] -> w960
                  tunnel: w962 -> [w965]
                  tunnel: w959 -> [w964]
                  tunnel: w958 -> [w963]
                  i -> [w966]
                  stop <- w968 stop-if-true
                  # "Attemp to Read Until\nMax Read Tx Attemps Limit"
                  n406 = call "ReadServo_R3.vi"("DIO Ref In"=w963, "VISA resource name out"=w964, "Servo ID"=w974) -> ("Error"=w971:u8, "Valid Checksum"=w972:bool, "Current Position"=w975:u64)  [unwired: 6 in]
                  n407 = Increment(x=w966) -> (x+1=w969:i32)
                  n408 = Equal To 0?(x=w971) -> (x = 0?=w973:bool)
                  n409 = Greater Or Equal?(x=w969, y=w965) -> (x >= y?=w970:bool)
                  n410 = And(x=w972, y=w973) -> (x .and. y?=w967:bool)
                  n411 = Or(x=w967, y=w970) -> (x .or. y?=w968:bool)
                }
              }
              frame #5 {
                n412 = local read "Servo Goal Position\n - Right"() -> (w979:u16)
                n413 = case shown="True" w981 {
                  tunnel: w982 -> [_ w986]
                  tunnel: w979 -> [_ w985]
                  frame False {
                    # "Don't update current position"
                  }
                  frame True {
                    # "Convert Received Position to Angle Relative to Robot"
                    # "45 DEG MOUNT OFFSET"
                    # "1024/300"
                    n414 = local write "Current R (10bit)"(w986) -> ()
                    n415 = Divide(x=w986, y=3.413333333333333) -> (x/y=w995:dbl)
                    n416 = Subtract(x=w995, y=sgl 60.0) -> (x-y=w993:dbl)
                    n417 = Subtract(x=w993, y=sgl 45.0) -> (x-y=w983:dbl)
                    n418 = To Word Integer(number=w985) -> (16bit integer=w990:i16)
                    n419 = To Word Integer(number=w986) -> (16bit integer=w991:i16)
                    n420 = shared-variable "RT myRIO Target - Overlord\\Localization_Variables_r0.lvlib\\Right Servo Angle_Current"(w983) -> ()  [unwired: 1 in, 1 out]
                    n421 = local write "Current Angle\n - Right (internal)"(w983) -> ()
                    n422 = Subtract(x=w990, y=w991) -> (x-y=w989:i16)
                    n423 = Absolute Value(x=w989) -> (abs(x)=w988:i16)
                    n424 = Greater?(x=w988, y=u16 5) -> (0:w984:bool)
                    n425 = local write "Move Servo - R"(w984) -> ()
                    n426 = local write "Servo Moving - R"(w984) -> ()
                  }
                }
              }
              frame #6 {
                n427 = local read "Move Servo - R"() -> (w998:bool)
                n428 = case shown="True" w998 {
                  tunnel: w1002 -> [_ w1007]
                  tunnel: w1004 -> [_ w1014]
                  tunnel: [TRUE w1015] -> w999
                  tunnel: w1003 -> [_ w1010]
                  tunnel: w1001 -> [_ w1009]
                  tunnel: w1000 -> [_ w1008]
                  frame False {
                  }
                  frame True {
                    w1017 = 1
                    # "High Byte"
                    # "Low Byte"
                    n429 = Type Cast(type="", x=w1007) -> (*(type *) &x=w1016:string)
                    n430 = local write "Servo Moving - R"(TRUE) -> ()
                    n431 = String Subset(string=w1016, offset (0)=1, length (rest)=w1017) -> (substring=w1013:string)
                    n432 = String Subset(string=w1016, offset (0)=0, length (rest)=w1017) -> (substring=w1012:string)
                    n433 = while {
                      tunnel: [w1026] -> w1015
                      tunnel: w1014 -> [w1031]
                      tunnel: w1013 -> [w1030]
                      tunnel: w1012 -> [w1029]
                      tunnel: w1010 -> [w1024]
                      tunnel: w1009 -> [w1022]
                      tunnel: w1008 -> [w1021]
                      i -> [w1025]
                      stop <- w1023 stop-if-true
                      # "Attemp to Write Until\nMax Write Tx Attemps Limit"
                      n434 = call "MoveServo_R3.vi"("DIO Ref Out"=w1021, "VISA resource name out"=w1022, "GP - Low Byte"=w1030, "GP - High Byte"=w1029, "Servo ID"=w1031) -> ("Valid Checksum"=w1033:bool, "Error"=w1032:u64)  [unwired: 5 in]
                      n435 = Increment(x=w1025) -> (x+1=w1027:i32)
                      n436 = Greater Or Equal?(x=w1027, y=w1024) -> (x >= y?=w1028:bool)
                      n437 = Equal To 0?(x=w1032) -> (x = 0?=w1034:bool)
                      n438 = And(x=w1033, y=w1034) -> (x .and. y?=w1026:bool)
                      n439 = Or(x=w1026, y=w1028) -> (x .or. y?=w1023:bool)
                    }
                  }
                }
                n440 = case shown="True" w999 {
                  frame False {
                  }
                  frame True {
                    # "Update Servo flag"
                    n441 = local write "Move Servo - R"(FALSE) -> ()
                  }
                }
              }
              frame #7 {
                n442 = call "Wait3"("Count(mSec)"=w1035) -> ()  [unwired: 1 out]
              }
              frame #8 {
                # "Increment Service Count"
                # "Update Compliance Slope\nEvery x loops"
                n443 = Equal?(x=w1039, y=u16 1000) -> (x = y?=w1048:bool)
                n444 = case shown="True" w1048 {
                  tunnel: w1044 -> [_ w1058]
                  tunnel: w1041 -> [_ w1057]
                  tunnel: w1040 -> [_ w1056]
                  tunnel: w1041 -> [_ w1055]
                  tunnel: w1040 -> [_ w1054]
                  tunnel: w1046 -> [_ w1053]
                  tunnel: w1045 -> [_ w1052]
                  tunnel: w1039 -> [w1049 _]
                  tunnel: [w1049 u16 0] -> w1047
                  tunnel: w1043 -> [_ w1050]
                  frame False {
                  }
                  frame True {
                    # "Reset Service\nCount"
                    n445 = flat-sequence {
                      tunnel: w1057 -> [w1063]
                      tunnel: w1056 -> [w1062]
                      tunnel: w1053 -> [w1064]
                      tunnel: [w1060] -> w1059
                      tunnel: w1058 -> [w1061]
                      tunnel: w1050 -> [w1060]
                      tunnel: w1052 -> [w1076]
                      tunnel: w1059 -> [w1075]
                      tunnel: w1058 -> [w1074]
                      tunnel: w1055 -> [w1073]
                      tunnel: w1054 -> [w1072]
                      frame #0 {
                        n446 = while {
                          tunnel: w1060 -> [w1071]
                          tunnel: w1063 -> [w1069]
                          tunnel: w1062 -> [w1068]
                          tunnel: w1064 -> [w1067]
                          tunnel: w1061 -> [w1066]
                          i -> [w1065]
                          stop <- w1070 stop-if-true
                          n447 = call "Set_Compliance_Slope_R2.vi"("Compliance Slope"=w1066, "DIO Ref Out"=w1068, "VISA resource name"=w1069, "Servo ID"=w1067) -> ()  [unwired: 6 in, 2 out]
                          n448 = Greater Or Equal?(x=w1065, y=w1071) -> (x >= y?=w1070:bool)
                        }
                      }
                      frame #1 {
                        n449 = while {
                          tunnel: w1075 -> [w1083]
                          tunnel: w1076 -> [w1081]
                          tunnel: w1073 -> [w1080]
                          tunnel: w1072 -> [w1079]
                          tunnel: w1074 -> [w1078]
                          i -> [w1077]
                          stop <- w1082 stop-if-true
                          n450 = call "Set_Compliance_Slope_R2.vi"("Compliance Slope"=w1078, "DIO Ref Out"=w1079, "VISA resource name"=w1080, "Servo ID"=w1081) -> ()  [unwired: 6 in, 2 out]
                          n451 = Greater Or Equal?(x=w1077, y=w1083) -> (x >= y?=w1082:bool)
                        }
                      }
                    }
                  }
                }
                n452 = Increment(x=w1047) -> (x+1=w1042:u16)
              }
            }
          }
        }
      }
    }
    frame #2 {
      n453 = VISA Close(VISA resource name=w1085) -> ()  [unwired: 1 in, 1 out]
      n454 = call <vilib>:"Close.vi"("DIO Ref In"=w1084) -> ()  [unwired: 10 in, 1 out]
    }
  }
  n455 = while {
    stop <- FALSE stop-if-true
    n456 = call "Wait9"("Count(mSec)"=u32 1000) -> ()  [unwired: 1 out]
  }
  n457 = while {
    shift-right: [w1146] -> _
    shift-left: "Initial Main State - Left" -> [w1171]
    shift-right: [w1138] -> _
    shift-left: "Search Direction - in - L" -> [w1165]
    shift-right: [w1137] -> _
    shift-left: FALSE -> [w1164]
    shift-right: [w1140] -> _
    shift-left: w13 -> [w1139]
    shift-right: [w1141] -> _
    shift-left: w13 -> [w1158]
    shift-right: [w1142] -> _
    shift-left: w13 -> [w1163]
    shift-right: [w1143] -> _
    shift-left: w13 -> [w1157]
    shift-right: [w1144] -> _
    shift-left: w13 -> [w1156]
    shift-right: [w1089] -> _
    shift-left: "Search Direction - in - Right" -> [w1113]
    shift-right: [w1134] -> _
    shift-left: FALSE -> [w1111]
    shift-right: [w1135] -> _
    shift-left: w12 -> [w1102]
    shift-right: [w1090] -> _
    shift-left: w12 -> [w1101]
    shift-right: [w1091] -> _
    shift-left: w12 -> [w1108]
    shift-right: [w1092] -> _
    shift-left: w12 -> [w1110]
    shift-right: [w1093] -> _
    shift-left: w12 -> [w1109]
    shift-right: [w1100] -> _
    shift-left: "Initial Main State- Right" -> [w1125]
    shift-right: [w1130] -> _
    shift-left: 0 -> [w1132]
    shift-right: [w1097] -> _
    shift-left: 0 -> [w1117]
    shift-right: [w1129] -> _
    shift-left: "Initial Tracking State - Left" -> [w1131]
    shift-right: [w1095] -> _
    shift-left: "Initial Tracking State - Right" -> [w1123]
    shift-right: [w1096] -> _
    shift-left: "Initial Recovery State  - Right" -> [w1124]
    shift-right: [w1127] -> _
    shift-left: "Initial Recovery State - L" -> [w1128]
    stop <- FALSE stop-if-true
    w1150 = T2."Tracking" ("Next Main State")
    # "Wait for New"
    # "ADD TRACKING TIMEOUT COUNT**********************"
    # "Service Track Angle Flag"
    # "Add Logic to Have Search Directions\nopposite if Both Searching"
    # "REMOVE LAST GOAL POSITION WITH cURRENT"
    # "Go to Current State"
    # "Add Logic to Have Search Directions\nopposite if Both Searching"
    # "Manuallly Reset\nRespond Var"
    # "Manuallly Reset\nRespond Var"
    # "Update Comm Process Variables"
    # "Both Tracking"
    # "Current delta - L"
    # "delta move sum - R"
    # "delta move sum - L"
    # "Current delta - R"
    # "Service Move Respond Variables"
    n458 = local read "Min Num Frames\nper Search"() -> (w1136:i32)
    n459 = local read "Minimum Delta \nServo Threshold"() -> (w1155:i16)
    n460 = local read "Maximum Move \nServo Threshold"() -> (w1154:i16)
    n461 = local read "Middle Beacon\nCoordinates"() -> (w1103:cluster{"X":sgl, "Y":sgl})
    n462 = local read "Position \nLock Status"() -> (w1162:bool)
    n463 = local read "Position \nLock Status"() -> (w1106:bool)
    n464 = local read "Search Step Size"() -> (w1153:u16)
    n465 = local read "Last Orientation"() -> (w1160:sgl)
    n466 = local read "Last Orientation"() -> (w1104:sgl)
    n467 = local read "Last Position"() -> (w1161:cluster{"X":sgl, "Y":sgl})
    n468 = local read "Last Position"() -> (w1105:cluster{"X":sgl, "Y":sgl})
    n469 = local read "Min Num Frames\nper Search"() -> (w1107:i32)
    n470 = call "Wait"("Count(mSec)"="Servo Algorithm\nCycle Time(ms)") -> ()  [unwired: 1 out]
    n471 = local read "Minimum Delta \nServo Threshold"() -> (w1115:i16)
    n472 = local read "Maximum Move \nServo Threshold"() -> (w1114:i16)
    n473 = local read "Search Step Size"() -> (w1112:u16)
    n474 = local read "New Data  Flag\nRight Servo"() -> (w1120:bool)
    n475 = local read "New Data  Flag\nLeft Servo"() -> (w1126:bool)
    n476 = local read "Image Lock - Right"() -> (w1122:bool)
    n477 = local read "Image Lock - Left"() -> (w1170:bool)
    n478 = local read "Tracking Angle - Right"() -> (w1119:sgl)
    n479 = local read "Tracking Angle - Left"() -> (w1168:sgl)
    n480 = local read "Current R (10bit)"() -> (w1118:u16)
    n481 = local read "Current L (10bit)"() -> (w1167:u16)
    n482 = case shown="True" w1120 {
      tunnel: [w1198 w1236] -> w1088
      tunnel: [w1192 w1235] -> w1099
      tunnel: w1125 -> [w1193 w1234]
      tunnel: w1122 -> [_ w1233]
      tunnel: "Track Angle Valid  - Right" -> [_ w1232]
      tunnel: w1119 -> [_ w1231]
      tunnel: w1118 -> [w1198 w1230]
      tunnel: "Mounting Offset - Right" -> [_ w1229]
      tunnel: w1113 -> [w1189 w1228]
      tunnel: w1111 -> [_ w1227]
      tunnel: w1108 -> [w1190 w1226]
      tunnel: w1106 -> [_ w1225]
      tunnel: w1105 -> [_ w1224]
      tunnel: w1104 -> [_ w1223]
      tunnel: w1103 -> [_ w1222]
      tunnel: w1101 -> [w1188 w1221]
      tunnel: w1110 -> [w1187 w1220]
      tunnel: w1109 -> [w1191 w1219]
      tunnel: w1115 -> [_ w1218]
      tunnel: w1114 -> [_ w1217]
      tunnel: w1112 -> [_ w1216]
      tunnel: [0 w1215] -> w1098
      tunnel: [w1193 w1214] -> w1100
      tunnel: [w1192 w1213] -> w1094
      tunnel: [w1191 w1212] -> w1093
      tunnel: [w1187 w1211] -> w1092
      tunnel: [w1190 w1210] -> w1091
      tunnel: [w1188 w1209] -> w1090
      tunnel: w1102 -> [_ w1208]
      tunnel: [w1189 w1207] -> w1089
      tunnel: w1107 -> [_ w1206]
      tunnel: w1117 -> [w1196 w1205]
      tunnel: w1123 -> [w1195 w1204]
      tunnel: [w1196 w1203] -> w1097
      tunnel: [w1195 w1202] -> w1095
      tunnel: w1124 -> [w1194 w1201]
      tunnel: [w1194 w1200] -> w1096
      frame False {
        w1192 = FALSE
        # "Recovery Mode COunt"
        # "Frames Processed - L"
        # "Recovery Search move Count - L"
        # "Recovery Search Attempt Count- L"
        # "WAITING FOR NEW IMAGE, RETAIN ALL VALUES"
      }
      frame True {
        w1238 = u16 1023
        w1241 = u16 0
        # "New Tracking State"
        # "Tracking Timeout Count"
        # "Next Main State"
        # "Next Recovery State"
        # "Reset Respond"
        # "Search Direction"
        # "Recovery Count"
        # "Recovery Search move Count"
        # "Recovery Search Attempt Count"
        # "Frames Processed"
        # "Apply Floor/Ceiling to Goal Position"
        # "Current move Delta"
        # "Service Track Angle Flag"
        # "Move Servo"
        # "Goal Position"
        # "Go to Current State"
        n483 = case shown="\"Recovery Mode\"" w1234 {
          tunnel: w1230 -> [w1260 w1337 w1515]
          tunnel: w1231 -> [_ w1339 _]
          tunnel: w1216 -> [w1259 _ w1510]
          tunnel: w1228 -> [w1258 w1319 w1504]
          tunnel: [w1257 w1335 w1514] -> w1242
          tunnel: [w1255 w1336 w1513] -> w1235
          tunnel: w1232 -> [w1253 w1330 w1491]
          tunnel: [w1252 w1332 w1500] -> w1214
          tunnel: w1233 -> [w1251 w1331 w1490]
          tunnel: w1229 -> [_ w1340 w1511]
          tunnel: w1218 -> [_ w1338 _]
          tunnel: [w1245 w1334 w1495] -> w1215
          tunnel: w1217 -> [_ w1333 _]
          tunnel: w1226 -> [w1250 _ w1505]
          tunnel: [enum16{"Generic Sweep", "Recovery Search"}."Recovery Search" enum16{"Generic Sweep", "Recovery Search"}."Recovery Search" w1512] -> w1200
          tunnel: w1221 -> [_ _ w1509]
          tunnel: w1201 -> [_ _ w1492]
          tunnel: w1227 -> [_ w1316 w1521]
          tunnel: w1208 -> [_ w1321 w1516]
          tunnel: w1223 -> [_ w1323 w1518]
          tunnel: w1224 -> [_ w1324 w1519]
          tunnel: w1225 -> [_ w1325 w1520]
          tunnel: w1222 -> [_ w1322 w1517]
          tunnel: [FALSE w1318 w1493] -> w1213
          tunnel: w1206 -> [w1249 _ w1503]
          tunnel: [w1245 w1313 w1502] -> w1209
          tunnel: [w1245 w1313 w1508] -> w1212
          tunnel: [w1245 w1313 w1507] -> w1211
          tunnel: [w1248 w1314 w1506] -> w1210
          tunnel: w1220 -> [_ _ w1498]
          tunnel: w1219 -> [_ _ w1497]
          tunnel: [w1246 w1319 w1496] -> w1207
          tunnel: w1205 -> [_ w1329 _]
          tunnel: [w1245 w1320 w1495] -> w1203
          tunnel: w1204 -> [_ w1326 _]
          tunnel: [enum16{"Track", "Reactive Predict", ""}."Track" ("Initial Tracking State - Right") w1317 enum16{"Track", "Reactive Predict", ""}."Track" ("Initial Tracking State - Right")] -> w1202
          frame "Start Up Search", Default {
            w1245 = u16 0
            # "Search Direction"
            # "Wait for 'x' Images to be Processed\nBefore Going to Next Step"
            # "Next Main State"
            # "New Goal Position"
            # "Move Servo"
            # "Choose Next State"
            # "Frames Processed Count"
            n484 = Greater Or Equal?(x=w1250, y=w1249) -> (x >= y?=w1256:bool)
            n485 = case shown="True" w1256 {
              tunnel: w1260 -> [w1275 w1287]
              tunnel: w1259 -> [_ w1285]
              tunnel: w1258 -> [w1274 w1284]
              tunnel: [w1275 w1281] -> w1257
              tunnel: [w1273 0] -> w1248
              tunnel: [FALSE TRUE] -> w1254
              tunnel: w1250 -> [w1276 _]
              tunnel: [w1274 w1278] -> w1246
              frame False {
                # "Increase Frames\nProcessed Count"
                n486 = Increment(x=w1276) -> (x+1=w1273:i32)
              }
              frame True {
                # "Reset Frames\nProcessed Count"
                # "SWEEP SEARCH - Startup"
                # "Multiple New Step\nby Step SIze"
                # "F = CCW\nT = CW"
                # "Last Direction"
                # "Min Step"
                # "add 10 in case\nactual position\nis lower than GP"
                # "Set New Step #"
                # "Choose Direction"
                # "Nearest step"
                # "Adjust Actual Posiiton\n to pre-determiend steps"
                # "Move Servo 1 \"Step\" to\nSearch"
                n487 = Add(x=3, y=w1287) -> (x+y=w1293:i32)
                n488 = Quotient & Remainder(x=w1293, y=w1285) -> (floor(x/y)=w1291:i32)  [unwired: 1 out]
                n489 = To Byte Integer(number=w1291) -> (8bit integer=w1282:i8)
                n490 = Less?(x=w1282, y=1) -> (x < y?=w1288:bool)
                n491 = case shown="False" w1288 {
                  tunnel: w1282 -> [w1304 w1312]
                  tunnel: [w1306 FALSE] -> w1278
                  tunnel: [w1305 w1312] -> w1290
                  tunnel: w1284 -> [w1303 _]
                  tunnel: w1285 -> [w1301 _]
                  frame False {
                    # "Max Step"
                    # "# of steps\nminus 1"
                    n492 = Divide(x=1024, y=w1301) -> (x/y=w1298:dbl)
                    n493 = To Unsigned Byte Integer(number=w1298) -> (unsigned 8bit integer=w1299:u8)
                    n494 = Greater Or Equal?(x=w1304, y=w1299) -> (x >= y?=w1300:bool)
                    n495 = case shown="True" w1300 {
                      tunnel: [w1307 TRUE] -> w1306
                      tunnel: [w1308 w1309] -> w1305
                      tunnel: w1304 -> [w1308 w1309]
                      tunnel: w1303 -> [w1307 _]
                      frame False {
                        # "No Need to\nChange Direction"
                      }
                      frame True {
                        # "T"
                        # "Move CW"
                      }
                    }
                  }
                  frame True {
                    # "F"
                    # "Move CCW"
                  }
                }
                n496 = case shown="False" w1278 {
                  tunnel: w1290 -> [w1295 w1296]
                  tunnel: [w1294 w1297] -> w1286
                  frame False {
                    # "CCW\n+1"
                    n497 = Increment(x=w1295) -> (x+1=w1294:i8)
                  }
                  frame True {
                    # "CW\n-1"
                    n498 = Decrement(x=w1296) -> (x-1=w1297:i8)
                  }
                }
                n499 = Multiply(x=w1286, y=w1285) -> (x*y=w1283:u16)
                n500 = To Unsigned Word Integer(number=w1283) -> (unsigned 16bit integer=w1281:u16)
              }
            }
            n501 = case shown="False" w1253 {
              tunnel: [w1264 FALSE] -> w1255
              tunnel: w1254 -> [w1264 _]
              tunnel: [w1265 w1270] -> w1252
              tunnel: w1251 -> [_ w1268]
              frame False {
                # "Check other Servo\nStay in Startup  State"
                n502 = local read "Track Angle Valid - Left"() -> (w1261:bool)
                n503 = local read "Image Lock - Left"() -> (w1262:bool)
                n504 = Or(x=w1261, y=w1262) -> (x .or. y?=w1263:bool)
                n505 = case shown="True" w1263 {
                  tunnel: [T2."Start Up Search" ("Next Main State") T2."Recovery Mode" ("Next Main State")] -> w1265
                  frame False {
                  }
                  frame True {
                  }
                }
              }
              frame True {
                # "Override Move Servo\nCommand bc an Angle Was Found\nduring this Step"
                # "Transition to Tracking State When\nImage Processing has Locked"
                n506 = case shown="False" w1268 {
                  tunnel: [T2."Start Up Search" ("Next Main State") T2."Tracking" ("Next Main State")] -> w1270
                  frame False {
                  }
                  frame True {
                  }
                }
              }
            }
          }
          frame "Tracking" {
            w1313 = 0
            # "Frames Processed Count"
            # "Image Lock - L"
            # "Track Angle Valid"
            # "Tracking Angle"
            # "Tracking Timeout Count"
            # "Max ove delta"
            # "Move delta threshold"
            # "mount offset"
            # "Current Position"
            # "Move Respond"
            # "Trackin Timeout count"
            # "Move Servo"
            # "delta"
            # "GP"
            # "Reset Move Respond"
            # "New Tracking State"
            # "Delta Move Sum"
            # "Choose Next State"
            n507 = case shown="\"Reactive Predict\"" w1326 {
              tunnel: w1340 -> [w1358 _]
              tunnel: w1339 -> [w1357 _]
              tunnel: w1338 -> [w1356 _]
              tunnel: w1337 -> [w1355 w1413]
              tunnel: [w1354 w1411] -> w1336
              tunnel: [w1353 w1419] -> w1335
              tunnel: [w1352 0] -> w1334
              tunnel: w1333 -> [w1351 _]
              tunnel: w1331 -> [w1350 w1403]
              tunnel: w1330 -> [w1349 w1406]
              tunnel: w1329 -> [w1348 w1408]
              tunnel: w1325 -> [_ w1418]
              tunnel: w1324 -> [_ w1417]
              tunnel: w1323 -> [_ w1416]
              tunnel: w1322 -> [_ w1415]
              tunnel: w1316 -> [_ w1414]
              tunnel: w1321 -> [_ w1412]
              tunnel: [TRUE w1409] -> w1318
              tunnel: [w1345 w1407] -> w1320
              tunnel: [w1343 w1405] -> w1317
              tunnel: [0 0] -> w1314
              frame "Track", Default {
                # "Reset"
                # "Tracking Timeout"
                # "Move Delta"
                # "Goal Position"
                # "Tracking Move"
                # "Move Servo"
                # "Only Consider Tracking Angle\n\nIF\n\nImage Locked        == T\nTrack Angle Flag   == T"
                n508 = And(x=w1350, y=w1349) -> (x .and. y?=w1342:bool)
                n509 = case shown="True" w1342 {
                  tunnel: w1358 -> [_ w1364]
                  tunnel: w1357 -> [_ w1382]
                  tunnel: w1356 -> [_ w1379]
                  tunnel: w1355 -> [w1361 w1369]
                  tunnel: [w1361 w1378] -> w1353
                  tunnel: [w1363 w1377] -> w1354
                  tunnel: [w1363 w1376] -> _
                  tunnel: [u16 0 w1375] -> w1352
                  tunnel: w1351 -> [_ w1371]
                  tunnel: w1348 -> [w1360 _]
                  tunnel: [w1359 0] -> w1345
                  frame False {
                    w1363 = FALSE
                    # "Increment timeout"
                    n510 = Increment(x=w1360) -> (x+1=w1359:i32)
                  }
                  frame True {
                    # "Convert Track Angle to UINT16"
                    # "1024/300"
                    # "Move to Tracking Angle \n\nif delta is greater than move servo threshold\nAND less than max move threshold"
                    n511 = Add(x=w1382, y=w1364) -> (x+y=w1385:sgl)
                    n512 = Add(x=w1385, y=sgl 60.0) -> (x+y=w1384:sgl)
                    n513 = Multiply(x=3.413333333333333, y=w1384) -> (x*y=w1365:dbl)
                    n514 = To Word Integer(number=w1369) -> (16bit integer=w1367:i16)
                    n515 = To Unsigned Word Integer(number=w1365) -> (unsigned 16bit integer=w1381:u16)
                    n516 = To Word Integer(number=w1365) -> (16bit integer=w1380:i16)
                    n517 = Subtract(x=w1380, y=w1367) -> (x-y=w1370:i16)
                    n518 = Absolute Value(x=w1370) -> (abs(x)=w1366:i16)
                    n519 = Greater Or Equal?(x=w1366, y=w1379) -> (x >= y?=w1373:bool)
                    n520 = Less Or Equal?(x=w1366, y=w1371) -> (x <= y?=w1372:bool)
                    n521 = And(x=w1373, y=w1372) -> (x .and. y?=w1374:bool)
                    n522 = case shown="True" w1374 {
                      tunnel: w1381 -> [_ w1393]
                      tunnel: [w1388 w1393] -> w1378
                      tunnel: [w1389 w1399] -> w1377
                      tunnel: [w1389 w1399] -> w1376
                      tunnel: w1369 -> [w1388 _]
                      tunnel: w1366 -> [_ w1398]
                      tunnel: [u16 0 w1398] -> w1375
                      tunnel: w1364 -> [_ w1392]
                      frame False {
                        w1389 = FALSE
                        # "Don't Move"
                      }
                      frame True {
                        w1399 = TRUE
                        # "45 DEG MOUNT OFFSET"
                        # "1024/300"
                        # "Current Delta"
                        # "Use new Track Angle"
                        n523 = Divide(x=w1393, y=3.413333333333333) -> (x/y=w1395:dbl)
                        n524 = Negate(x=w1392) -> (-x=w1391:sgl)
                        n525 = Subtract(x=w1395, y=sgl 60.0) -> (x-y=w1397:dbl)
                        n526 = Add(x=w1397, y=w1391) -> (x+y=w1390:dbl)
                        n527 = local write "Last Track Angle - R"(w1390) -> ()
                      }
                    }
                  }
                }
                n528 = local read "Timeout to \nEnable Reactive Predict"() -> (w1346:u16)
                n529 = Less?(x=w1345, y=w1346) -> (x < y?=w1344:bool)
                n530 = case shown="False" w1344 {
                  tunnel: [enum16{"Track", "Reactive Predict", ""}."Reactive Predict" ("Initial Tracking State - Right") enum16{"Track", "Reactive Predict", ""}."Track" ("Initial Tracking State - Right")] -> w1343
                  frame False {
                  }
                  frame True {
                  }
                }
              }
              frame "Reactive Predict" {
                # "Choose New\nTracking State"
                n531 = Or(x=w1403, y=w1406) -> (x .or. y?=w1402:bool)
                n532 = case shown="False" w1402 {
                  tunnel: [w1432 w1484] -> w1419
                  tunnel: w1418 -> [w1431 _]
                  tunnel: w1417 -> [w1430 _]
                  tunnel: w1416 -> [w1429 _]
                  tunnel: w1415 -> [w1428 _]
                  tunnel: w1414 -> [w1427 _]
                  tunnel: w1412 -> [w1426 _]
                  tunnel: [w1425 w1483] -> w1411
                  tunnel: [w1424 w1483] -> w1409
                  tunnel: w1408 -> [w1423 _]
                  tunnel: [w1422 0] -> w1407
                  tunnel: [enum16{"Track", "Reactive Predict", ""}."Reactive Predict" ("Initial Tracking State - Right") enum16{"Track", "Reactive Predict", ""}."Track" ("Initial Tracking State - Right")] -> w1405
                  tunnel: w1413 -> [w1420 w1484]
                  frame False {
                    # "Stay in Reactive State"
                    # "Increment Track Timeout"
                    # "Move Respond Flag"
                    n533 = Increment(x=w1423) -> (x+1=w1422:i32)
                    n534 = case shown="True" w1427 {
                      tunnel: w1431 -> [_ w1447]
                      tunnel: w1430 -> [_ w1446]
                      tunnel: w1429 -> [_ w1445]
                      tunnel: w1428 -> [_ w1444]
                      tunnel: w1426 -> [_ w1441]
                      tunnel: [w1433 w1437] -> w1432
                      tunnel: [w1434 w1436] -> w1425
                      tunnel: [w1434 w1436] -> w1424
                      tunnel: w1420 -> [w1433 w1435]
                      frame False {
                        w1434 = FALSE
                        # "Reset Move Respond = F"
                        # "Move Servo = F"
                      }
                      frame True {
                        w1436 = TRUE
                        # "Position Lock"
                        # "Current Servo\nPosition"
                        # "Reset Move\nRespond = T"
                        # "Move Servo = T"
                        # "Apply Direction \nto Offset (delta sum)"
                        # "Check Last Known Position of Robot"
                        n535 = case shown="True" w1447 {
                          tunnel: w1446 -> [_ w1475]
                          tunnel: w1445 -> [_ w1450]
                          tunnel: w1444 -> [_ w1451]
                          tunnel: [sgl 1.0 ("y") w1449] -> w1443
                          frame False {
                            # "No Position Data Available"
                            # "Default is to move\nSame Direction as other\nServo"
                          }
                          frame True {
                            w1456 = sgl 1.0 ("y")
                            # "Use previous position/orientation to Guess Which Direction to Move Servo"
                            # "Choose Search Direction"
                            # "\"Perpendicular \nThreshold\""
                            # "If Orientation is\n ~Perpendicular -> Start Search\n in Opposite Direction of Other"
                            # "****add 90 until orientation angle is fixed"
                            # "Last Orientation"
                            # "Convert to Rad"
                            # "Avoid Divide by 0"
                            # "-1/m"
                            # "Calculate Normal Line to \nLast Robot Position\nfrom Center Beacon"
                            # "last Position \nCoordinates"
                            n536 = Unbundle(w1475) -> ("X"=w1455:sgl, "Y"=w1454:sgl)
                            n537 = Unbundle(w1451) -> ("X"=w1453:sgl, "Y"=w1452:sgl)
                            n538 = Subtract(x=w1454, y=w1452) -> (x-y=w1471:sgl)
                            n539 = Subtract(x=w1455, y=w1453) -> (x-y=w1469:sgl)
                            n540 = Equal To 0?(x=w1469) -> (x = 0?=w1470:bool)
                            n541 = case shown="False" w1470 {
                              tunnel: w1471 -> [w1478 _]
                              tunnel: w1469 -> [w1477 _]
                              tunnel: [w1476 1000000000000000.0] -> w1468
                              frame False {
                                n542 = Divide(x=w1478, y=w1477) -> (x/y=w1476:sgl)
                              }
                              frame True {
                              }
                            }
                            n543 = Equal To 0?(x=w1468) -> (x = 0?=w1473:bool)
                            n544 = case shown="False" w1473 {
                              tunnel: [w1480 1e-08] -> w1472
                              tunnel: w1468 -> [w1480 _]
                              frame False {
                              }
                              frame True {
                                # "Can't have infinit slope"
                              }
                            }
                            n545 = Divide(x=-1.0, y=w1472) -> (x/y=w1467:dbl)
                            n546 = Inverse Tangent(1:w1467) -> (0:w1465:dbl)
                            n547 = expression code="(x/pi)*180.0" "radians to degrees"(w1465) -> (w1466:dbl)
                            n548 = To Single Precision Float(number=w1466) -> (single precision float=w1463:sgl)
                            n549 = Add(x=w1450, y=sgl 90.0) -> (x+y=w1462:sgl)
                            n550 = Subtract(x=w1463, y=w1462) -> (x-y=w1461:sgl)
                            n551 = Absolute Value(x=w1461) -> (abs(x)=w1460:sgl)
                            n552 = Less Or Equal?(x=w1460, y=sgl 10.0) -> (x <= y?=w1458:bool)
                            n553 = Negate(x=w1456) -> (-x=w1457:sgl)
                            n554 = Select(t=w1457, s=w1458, f=w1456) -> (s? t:f=w1449:sgl)
                          }
                        }
                        n555 = To Word Integer(number=w1443) -> (16bit integer=w1442:i16)
                        n556 = Multiply(x=w1442, y=w1441) -> (x*y=w1440:i32)
                        n557 = To Word Integer(number=w1435) -> (16bit integer=w1439:i16)
                        n558 = Add(x=w1440, y=w1439) -> (x+y=w1438:i32)
                        n559 = To Unsigned Word Integer(number=w1438) -> (unsigned 16bit integer=w1437:u16)
                      }
                    }
                  }
                  frame True {
                    w1483 = TRUE
                    # "Go Directly to Track State"
                  }
                }
              }
            }
            n560 = local read "Tracking Timeout\nThreshold"() -> (w1327:i32)
            n561 = Less?(x=w1320, y=w1327) -> (x < y?=w1328:bool)
            n562 = case shown="False" w1328 {
              tunnel: [T2."Recovery Mode" ("Next Main State") T2."Tracking" ("Next Main State")] -> w1332
              frame False {
              }
              frame True {
              }
            }
          }
          frame "Recovery Mode" {
            w1495 = u16 0
            # "Increment Recovery Mode Count"
            # "Recovvery Mode\nCount"
            # "Frames Processed"
            # "Choose Next Main State"
            # "Reset recovery count"
            # "Recovery move\nCount"
            # "Recovery Search\nAttempt count"
            # "Move Servo = T"
            # "delta move sum"
            # "Robot Position Valid"
            n563 = local read "Image Lock - Left"() -> (w1499:bool)
            n564 = Or(x=w1490, y=w1491) -> (x .or. y?=w1489:bool)
            n565 = case shown="\"Recovery Search\"" w1492 {
              tunnel: w1521 -> [_ _]
              tunnel: w1520 -> [_ _]
              tunnel: w1519 -> [_ _]
              tunnel: w1518 -> [_ _]
              tunnel: w1517 -> [_ _]
              tunnel: w1516 -> [_ _]
              tunnel: w1515 -> [w1549 w1635]
              tunnel: [w1541 w1633] -> w1514
              tunnel: [w1538 w1627] -> w1513
              tunnel: [FALSE FALSE] -> w1493
              tunnel: [w1543 w1624] -> w1512
              tunnel: w1509 -> [w1547 _]
              tunnel: w1511 -> [w1550 _]
              tunnel: w1510 -> [w1548 w1630]
              tunnel: [w1540 w1623] -> w1507
              tunnel: [w1539 w1623] -> w1508
              tunnel: w1499 -> [w1537 _]
              tunnel: [w1528 w1634] -> w1506
              tunnel: w1505 -> [w1526 w1618]
              tunnel: w1504 -> [w1531 w1631]
              tunnel: w1503 -> [w1527 w1629]
              tunnel: w1490 -> [_ _]
              tunnel: w1491 -> [_ w1626]
              tunnel: [FALSE w1625] -> w1501
              tunnel: w1498 -> [w1535 _]
              tunnel: w1497 -> [w1534 _]
              tunnel: [w1531 w1622] -> w1496
              frame "Recovery Search" {
                # "Wait for 2 Images to be Processed\nBefore Going to Next Step"
                # "Choose Next Reovery State"
                # "Recovery Search \nAttempt Count"
                # "Move Servo"
                # "Goal Position"
                # "Recovery Search\nmove Count"
                # "Attempt Recovery Search if Other Servo has Valid Angle"
                n566 = local read "Last Track Angle - L"() -> (w1530:sgl)
                n567 = Greater Or Equal?(x=w1526, y=w1527) -> (x >= y?=w1529:bool)
                n568 = case shown="True" w1529 {
                  tunnel: w1550 -> [_ w1570]
                  tunnel: [w1555 w1569] -> w1539
                  tunnel: w1549 -> [w1558 w1568]
                  tunnel: w1548 -> [_ w1567]
                  tunnel: [w1556 w1566] -> w1540
                  tunnel: [w1558 w1565] -> w1541
                  tunnel: [FALSE w1564] -> w1538
                  tunnel: w1535 -> [w1556 w1563]
                  tunnel: w1534 -> [w1555 w1562]
                  tunnel: w1537 -> [_ w1561]
                  tunnel: w1530 -> [_ w1560]
                  tunnel: [w1553 0 ("Frames Processed\nCount - in")] -> w1528
                  tunnel: w1526 -> [w1554 _]
                  frame False {
                    # "Increment Frames Processed"
                    # "WAIT"
                    n569 = Increment(x=w1554) -> (x+1=w1553:i32)
                  }
                  frame True {
                    n570 = case shown="True" w1561 {
                      tunnel: w1560 -> [_ w1583]
                      tunnel: w1563 -> [w1571 w1579]
                      tunnel: w1570 -> [_ w1584]
                      tunnel: [w1574 w1582] -> w1565
                      tunnel: [w1572 w1581] -> w1569
                      tunnel: w1562 -> [w1572 w1580]
                      tunnel: w1568 -> [w1574 w1578]
                      tunnel: w1567 -> [_ w1577]
                      tunnel: [FALSE TRUE] -> w1564
                      tunnel: [w1571 w1575] -> w1566
                      frame False {
                        # "Don't Move bc Other Servo Doesn't Have Image Lock"
                      }
                      frame True {
                        # "Move Servo = T"
                        n571 = Greater Than 0?(x=w1579) -> (x > 0?=w1585:bool)
                        n572 = case shown="False" w1585 {
                          tunnel: w1584 -> [w1592 _]
                          tunnel: w1583 -> [w1586 _]
                          tunnel: [w1591 w1602] -> w1582
                          tunnel: [w1589 w1608] -> w1581
                          tunnel: w1580 -> [w1590 w1608]
                          tunnel: w1579 -> [w1588 w1605]
                          tunnel: [w1587 w1607] -> w1575
                          tunnel: w1578 -> [_ w1603]
                          tunnel: w1577 -> [_ w1600]
                          frame False {
                            # "Increment move count to transition\nto Pan mode"
                            # "Increment Recovery Search Attempt Count"
                            # "1024/300"
                            # "Move Parallel to Other Servo"
                            n573 = Increment(x=w1590) -> (x+1=w1589:i32)
                            n574 = Add(x=w1586, y=w1592) -> (x+y=w1598:sgl)
                            n575 = Add(x=w1598, y=sgl 60.0) -> (x+y=w1597:sgl)
                            n576 = Multiply(x=3.413333333333333, y=w1597) -> (x*y=w1595:dbl)
                            n577 = Add(x=0.5, y=w1595) -> (x+y=w1593:dbl)
                            n578 = To Unsigned Word Integer(number=w1593) -> (unsigned 16bit integer=w1591:u16)
                            n579 = Increment(x=w1588) -> (x+1=w1587:i32)
                          }
                          frame True {
                            # "Apply Direction"
                            # "Step SIze"
                            # "Current Position"
                            # "Attempt to Pan in Steps Towards other Servo"
                            # "Could be same or function of \nregular search step size"
                            # "Max # of Pan\nMoves"
                            # "Pan Towards Other Servo"
                            n580 = Greater Or Equal?(x=w1605, y=u16 20) -> (x >= y?=w1606:bool)
                            n581 = case shown="False" w1606 {
                              tunnel: w1605 -> [w1616 _]
                              tunnel: [w1615 u16 0] -> w1607
                              frame False {
                                # "Increment Pan Count"
                                n582 = Increment(x=w1616) -> (x+1=w1615:i32)
                              }
                              frame True {
                                # "Reset move count"
                              }
                            }
                            n583 = local read "Recovery Search\nDirection - R"() -> (w1601:bool)
                            n584 = case shown="False" w1601 {
                              tunnel: w1603 -> [w1610 w1614]
                              tunnel: w1600 -> [w1611 w1613]
                              tunnel: [w1609 w1612] -> w1602
                              frame False {
                                # "CCW"
                                n585 = Add(x=w1610, y=w1611) -> (x+y=w1609:u16)
                              }
                              frame True {
                                # "CW"
                                n586 = Subtract(x=w1614, y=w1613) -> (x-y=w1612:u16)
                              }
                            }
                          }
                        }
                      }
                    }
                  }
                }
                n587 = local read "Max Recovery Count\n(Recovery Search)"() -> (w1532:u16)
                n588 = local read "Max Recovery\nSearch Attempts"() -> (w1533:u16)
                n589 = Less Or Equal?(x=w1539, y=w1533) -> (x <= y?=w1545:bool)
                n590 = Less Or Equal?(x=w1547, y=w1532) -> (x <= y?=w1546:bool)
                n591 = And(x=w1545, y=w1546) -> (x .and. y?=w1544:bool)
                n592 = case shown="True" w1544 {
                  tunnel: [enum16{"Generic Sweep", "Recovery Search"}."Generic Sweep" enum16{"Generic Sweep", "Recovery Search"}."Recovery Search"] -> w1543
                  frame False {
                  }
                  frame True {
                  }
                }
              }
              frame "Generic Sweep" {
                w1623 = u16 0
                # "Angle Valid?"
                # "Choose Next Recovery State"
                # "Wait for 2 Images to be Processed\nBefore Going to Next Step"
                # "New Goal Position"
                # "Move Servo"
                # "Frames Processed Count"
                n593 = Greater Or Equal?(x=w1618, y=w1629) -> (x >= y?=w1636:bool)
                n594 = case shown="True" w1636 {
                  tunnel: w1635 -> [w1652 w1664]
                  tunnel: w1630 -> [_ w1662]
                  tunnel: w1631 -> [w1651 w1661]
                  tunnel: [w1652 w1658] -> w1633
                  tunnel: [w1650 0] -> w1634
                  tunnel: [FALSE TRUE] -> w1628
                  tunnel: w1618 -> [w1653 _]
                  tunnel: [w1651 w1655] -> w1622
                  frame False {
                    # "Increment Frames Processed"
                    n595 = Increment(x=w1653) -> (x+1=w1650:i32)
                  }
                  frame True {
                    # "Reset Frames\nProcessed Count"
                    # "SWEEP SEARCH - Startup"
                    # "Multiple New Step\nby Step SIze"
                    # "F = CCW\nT = CW"
                    # "Last Direction"
                    # "Min Step"
                    # "add 10 in case\nactual position\nis lower than GP"
                    # "Set New Step #"
                    # "Choose Direction"
                    # "Nearest step"
                    # "Adjust Actual Posiiton\n to pre-determiend steps"
                    # "Move Servo 1 \"Step\" to\nSearch"
                    n596 = Add(x=5, y=w1664) -> (x+y=w1670:i32)
                    n597 = Quotient & Remainder(x=w1670, y=w1662) -> (floor(x/y)=w1668:i32)  [unwired: 1 out]
                    n598 = To Byte Integer(number=w1668) -> (8bit integer=w1659:i8)
                    n599 = Less?(x=w1659, y=1) -> (x < y?=w1665:bool)
                    n600 = case shown="False" w1665 {
                      tunnel: w1659 -> [w1681 w1689]
                      tunnel: [w1683 FALSE] -> w1655
                      tunnel: [w1682 w1689] -> w1667
                      tunnel: w1661 -> [w1680 _]
                      tunnel: w1662 -> [w1678 _]
                      frame False {
                        # "Max Step"
                        # "# of steps\nminus 1"
                        n601 = Divide(x=1024, y=w1678) -> (x/y=w1675:dbl)
                        n602 = To Unsigned Byte Integer(number=w1675) -> (unsigned 8bit integer=w1676:u8)
                        n603 = Greater Or Equal?(x=w1681, y=w1676) -> (x >= y?=w1677:bool)
                        n604 = case shown="True" w1677 {
                          tunnel: [w1684 TRUE] -> w1683
                          tunnel: [w1685 w1686] -> w1682
                          tunnel: w1681 -> [w1685 w1686]
                          tunnel: w1680 -> [w1684 _]
                          frame False {
                            # "No Need to\nChange Direction"
                          }
                          frame True {
                            # "T"
                            # "Move CW"
                          }
                        }
                      }
                      frame True {
                        # "F"
                        # "Move CCW"
                      }
                    }
                    n605 = case shown="True" w1655 {
                      tunnel: w1667 -> [w1672 w1673]
                      tunnel: [w1671 w1674] -> w1663
                      frame False {
                        # "CCW\n+1"
                        n606 = Increment(x=w1672) -> (x+1=w1671:i8)
                      }
                      frame True {
                        # "CW\n-1"
                        n607 = Decrement(x=w1673) -> (x-1=w1674:i8)
                      }
                    }
                    n608 = Multiply(x=w1663, y=w1662) -> (x*y=w1660:u16)
                    n609 = To Unsigned Word Integer(number=w1660) -> (unsigned 16bit integer=w1658:u16)
                  }
                }
                n610 = local read "Track Angle Valid - Left"() -> (w1621:bool)
                n611 = local read "Image Lock - Left"() -> (w1620:bool)
                n612 = Or(x=w1620, y=w1621) -> (x .or. y?=w1619:bool)
                n613 = case shown="False" w1626 {
                  tunnel: [w1639 w1649] -> w1627
                  tunnel: w1628 -> [w1640 _]
                  tunnel: [w1641 enum16{"Generic Sweep", "Recovery Search"}."Generic Sweep"] -> w1624
                  tunnel: [w1638 w1649] -> w1625
                  tunnel: w1619 -> [w1637 _]
                  frame False {
                    # "Is other servo tracking?"
                    n614 = case shown="True" w1637 {
                      tunnel: [enum16{"Generic Sweep", "Recovery Search"}."Generic Sweep" enum16{"Generic Sweep", "Recovery Search"}."Recovery Search"] -> w1641
                      tunnel: w1640 -> [w1644 _]
                      tunnel: [w1644 FALSE] -> w1639
                      tunnel: [FALSE TRUE] -> w1638
                      frame False {
                        # "Stay in Sweep"
                      }
                      frame True {
                        # "G o to Recovery Search  State"
                      }
                    }
                  }
                  frame True {
                    w1649 = FALSE
                    # "Override Move Servo\nCommand bc an Angle Was Found\nduring this Step"
                    # "Stay In Sweep\nLet Main State Machine transition\ninto Tracking"
                  }
                }
              }
            }
            n615 = Increment(x=w1509) -> (x+1=w1488:i32)
            n616 = case shown="True" w1501 {
              tunnel: w1488 -> [w1524 _]
              tunnel: [w1524 0] -> w1502
              frame False {
              }
              frame True {
              }
            }
            n617 = case shown="False" w1489 {
              tunnel: [T2."Recovery Mode" ("Next Main State") T2."Tracking" ("Next Main State")] -> w1500
              frame False {
              }
              frame True {
              }
            }
          }
        }
        "Current Move Delta - L 2" <- w1215
        n618 = Less?(x=w1242, y=w1241) -> (x < y?=w1240:bool)
        n619 = local write "New Data  Flag\nRight Servo"(FALSE) -> ()
        n620 = Select(t=w1241, s=w1240, f=w1242) -> (s? t:f=w1237:u16)
        n621 = Greater?(x=w1237, y=w1238) -> (0:w1239:bool)
        n622 = Select(t=w1238, s=w1239, f=w1237) -> (s? t:f=w1236:u16)
      }
    }
    "Next Main State - Right" <- w1100
    "Next Tracking State - Right" <- w1095
    "Next Recovery State - Right" <- w1096
    n623 = case shown="True" w1126 {
      tunnel: [w1701 w1739] -> w1173
      tunnel: [w1695 w1738] -> w1172
      tunnel: w1171 -> [w1696 w1737]
      tunnel: w1170 -> [_ w1736]
      tunnel: "Track Angle Valid - Left" -> [_ w1735]
      tunnel: w1168 -> [_ w1734]
      tunnel: w1167 -> [w1701 w1733]
      tunnel: "Mounting Offset - Left" -> [_ w1732]
      tunnel: w1165 -> [w1692 w1731]
      tunnel: w1164 -> [_ w1730]
      tunnel: w1163 -> [w1693 w1729]
      tunnel: w1162 -> [_ w1728]
      tunnel: w1161 -> [_ w1727]
      tunnel: w1160 -> [_ w1726]
      tunnel: "Middle Beacon\nCoordinates" -> [_ w1725]
      tunnel: w1158 -> [w1691 w1724]
      tunnel: w1157 -> [w1690 w1723]
      tunnel: w1156 -> [w1694 w1722]
      tunnel: w1155 -> [_ w1721]
      tunnel: w1154 -> [_ w1720]
      tunnel: w1153 -> [_ w1719]
      tunnel: [0 w1718] -> w1147
      tunnel: [w1696 w1717] -> w1146
      tunnel: [w1695 w1716] -> w1145
      tunnel: [w1694 w1715] -> w1144
      tunnel: [w1690 w1714] -> w1143
      tunnel: [w1693 w1713] -> w1142
      tunnel: [w1691 w1712] -> w1141
      tunnel: w1139 -> [_ w1711]
      tunnel: [w1692 w1710] -> w1138
      tunnel: w1136 -> [_ w1709]
      tunnel: w1132 -> [w1699 w1708]
      tunnel: w1131 -> [w1698 w1707]
      tunnel: [w1699 w1706] -> w1130
      tunnel: [w1698 w1705] -> w1129
      tunnel: w1128 -> [w1697 w1704]
      tunnel: [w1697 w1703] -> w1127
      frame False {
        w1695 = FALSE
        # "Recovery Mode COunt"
        # "Frames Processed - L"
        # "Recovery Search move Count - L"
        # "Recovery Search Attempt Count- L"
        # "WAITING FOR NEW IMAGE, RETAIN ALL VALUES"
      }
      frame True {
        w1741 = u16 1023
        w1744 = u16 0
        # "New Tracking State"
        # "Tracking Timeout Count"
        # "Next Main State"
        # "Next Recovery State"
        # "Reset Respond"
        # "Search Direction"
        # "Recovery Count"
        # "Recovery Search move Count"
        # "Recovery Search Attempt Count"
        # "Frames Processed"
        # "Apply Floor/Ceiling to Goal Position"
        # "Current move Delta"
        # "Service Track Angle Flag"
        # "Move Servo"
        # "Goal Position"
        # "Go to Current State"
        n624 = case shown="\"Recovery Mode\"" w1737 {
          tunnel: w1733 -> [w1763 w1840 w2018]
          tunnel: w1734 -> [_ w1842 _]
          tunnel: w1719 -> [w1762 _ w2013]
          tunnel: w1731 -> [w1761 w1822 w2007]
          tunnel: [w1760 w1838 w2017] -> w1745
          tunnel: [w1758 w1839 w2016] -> w1738
          tunnel: w1735 -> [w1756 w1833 w1994]
          tunnel: [w1755 w1835 w2003] -> w1717
          tunnel: w1736 -> [w1754 w1834 w1993]
          tunnel: w1732 -> [_ w1843 w2014]
          tunnel: w1721 -> [_ w1841 _]
          tunnel: [w1748 w1837 w1998] -> w1718
          tunnel: w1720 -> [_ w1836 _]
          tunnel: w1729 -> [w1753 _ w2008]
          tunnel: [enum16{"Generic Sweep", "Recovery Search"}."Recovery Search" enum16{"Generic Sweep", "Recovery Search"}."Recovery Search" w2015] -> w1703
          tunnel: w1724 -> [_ _ w2012]
          tunnel: w1704 -> [_ _ w1995]
          tunnel: w1730 -> [_ w1819 w2024]
          tunnel: w1711 -> [_ w1824 w2019]
          tunnel: w1726 -> [_ w1826 w2021]
          tunnel: w1727 -> [_ w1827 w2022]
          tunnel: w1728 -> [_ w1828 w2023]
          tunnel: w1725 -> [_ w1825 w2020]
          tunnel: [FALSE w1821 w1996] -> w1716
          tunnel: w1709 -> [w1752 _ w2006]
          tunnel: [w1748 w1816 w2005] -> w1712
          tunnel: [w1748 w1816 w2011] -> w1715
          tunnel: [w1748 w1816 w2010] -> w1714
          tunnel: [w1751 w1817 w2009] -> w1713
          tunnel: w1723 -> [_ _ w2001]
          tunnel: w1722 -> [_ _ w2000]
          tunnel: [w1749 w1822 w1999] -> w1710
          tunnel: w1708 -> [_ w1832 _]
          tunnel: [w1748 w1823 w1998] -> w1706
          tunnel: w1707 -> [_ w1829 _]
          tunnel: [enum16{"Track", "Reactive Predict", ""}."Track" ("Initial Tracking State - Right") w1820 enum16{"Track", "Reactive Predict", ""}."Track" ("Initial Tracking State - Right")] -> w1705
          frame "Start Up Search", Default {
            w1748 = u16 0
            # "Search Direction"
            # "Wait for 'x' Images to be Processed\nBefore Going to Next Step"
            # "Next Main State"
            # "New Goal Position"
            # "Move Servo"
            # "Choose Next State"
            # "Frames Processed Count"
            n625 = Greater Or Equal?(x=w1753, y=w1752) -> (x >= y?=w1759:bool)
            n626 = case shown="True" w1759 {
              tunnel: w1763 -> [w1778 w1790]
              tunnel: w1762 -> [_ w1788]
              tunnel: w1761 -> [w1777 w1787]
              tunnel: [w1778 w1784] -> w1760
              tunnel: [w1776 0] -> w1751
              tunnel: [FALSE TRUE] -> w1757
              tunnel: w1753 -> [w1779 _]
              tunnel: [w1777 w1781] -> w1749
              frame False {
                # "Increase Frames\nProcessed Count"
                n627 = Increment(x=w1779) -> (x+1=w1776:i32)
              }
              frame True {
                # "Reset Frames\nProcessed Count"
                # "SWEEP SEARCH - Startup"
                # "Multiple New Step\nby Step SIze"
                # "F = CCW\nT = CW"
                # "Last Direction"
                # "Min Step"
                # "add 10 in case\nactual position\nis lower than GP"
                # "Set New Step #"
                # "Choose Direction"
                # "Nearest step"
                # "Adjust Actual Posiiton\n to pre-determiend steps"
                # "Move Servo 1 \"Step\" to\nSearch"
                n628 = Add(x=3, y=w1790) -> (x+y=w1796:i32)
                n629 = Quotient & Remainder(x=w1796, y=w1788) -> (floor(x/y)=w1794:i32)  [unwired: 1 out]
                n630 = To Byte Integer(number=w1794) -> (8bit integer=w1785:i8)
                n631 = Less?(x=w1785, y=1) -> (x < y?=w1791:bool)
                n632 = case shown="False" w1791 {
                  tunnel: w1785 -> [w1807 w1815]
                  tunnel: [w1809 FALSE] -> w1781
                  tunnel: [w1808 w1815] -> w1793
                  tunnel: w1787 -> [w1806 _]
                  tunnel: w1788 -> [w1804 _]
                  frame False {
                    # "Max Step"
                    # "# of steps\nminus 1"
                    n633 = Divide(x=1024, y=w1804) -> (x/y=w1801:dbl)
                    n634 = To Unsigned Byte Integer(number=w1801) -> (unsigned 8bit integer=w1802:u8)
                    n635 = Greater Or Equal?(x=w1807, y=w1802) -> (x >= y?=w1803:bool)
                    n636 = case shown="True" w1803 {
                      tunnel: [w1810 TRUE] -> w1809
                      tunnel: [w1811 w1812] -> w1808
                      tunnel: w1807 -> [w1811 w1812]
                      tunnel: w1806 -> [w1810 _]
                      frame False {
                        # "No Need to\nChange Direction"
                      }
                      frame True {
                        # "T"
                        # "Move CW"
                      }
                    }
                  }
                  frame True {
                    # "F"
                    # "Move CCW"
                  }
                }
                n637 = case shown="False" w1781 {
                  tunnel: w1793 -> [w1798 w1799]
                  tunnel: [w1797 w1800] -> w1789
                  frame False {
                    # "CCW\n+1"
                    n638 = Increment(x=w1798) -> (x+1=w1797:i8)
                  }
                  frame True {
                    # "CW\n-1"
                    n639 = Decrement(x=w1799) -> (x-1=w1800:i8)
                  }
                }
                n640 = Multiply(x=w1789, y=w1788) -> (x*y=w1786:u16)
                n641 = To Unsigned Word Integer(number=w1786) -> (unsigned 16bit integer=w1784:u16)
              }
            }
            n642 = case shown="False" w1756 {
              tunnel: [w1767 FALSE] -> w1758
              tunnel: w1757 -> [w1767 _]
              tunnel: [w1768 w1773] -> w1755
              tunnel: w1754 -> [_ w1771]
              frame False {
                # "Check other Servo\nStay in Startup  State"
                n643 = local read "Track Angle Valid  - Right"() -> (w1764:bool)
                n644 = local read "Image Lock - Right"() -> (w1765:bool)
                n645 = Or(x=w1764, y=w1765) -> (x .or. y?=w1766:bool)
                n646 = case shown="True" w1766 {
                  tunnel: [T2."Start Up Search" ("Next Main State") T2."Recovery Mode" ("Next Main State")] -> w1768
                  frame False {
                  }
                  frame True {
                  }
                }
              }
              frame True {
                # "Override Move Servo\nCommand bc an Angle Was Found\nduring this Step"
                # "Transition to Tracking State When\nImage Processing has Locked"
                n647 = case shown="False" w1771 {
                  tunnel: [T2."Start Up Search" ("Next Main State") T2."Tracking" ("Next Main State")] -> w1773
                  frame False {
                  }
                  frame True {
                  }
                }
              }
            }
          }
          frame "Tracking" {
            w1816 = 0
            # "Frames Processed Count"
            # "Image Lock - L"
            # "Track Angle Valid"
            # "Tracking Angle"
            # "Tracking Timeout Count"
            # "Max ove delta"
            # "Move delta threshold"
            # "mount offset"
            # "Current Position"
            # "Move Respond"
            # "Trackin Timeout count"
            # "Move Servo"
            # "delta"
            # "GP"
            # "Reset Move Respond"
            # "New Tracking State"
            # "Delta Move Sum"
            # "Choose Next State"
            n648 = case shown="\"Track\", Default" w1829 {
              tunnel: w1843 -> [w1861 _]
              tunnel: w1842 -> [w1860 _]
              tunnel: w1841 -> [w1859 _]
              tunnel: w1840 -> [w1858 w1916]
              tunnel: [w1857 w1914] -> w1839
              tunnel: [w1856 w1922] -> w1838
              tunnel: [w1855 0] -> w1837
              tunnel: w1836 -> [w1854 _]
              tunnel: w1834 -> [w1853 w1906]
              tunnel: w1833 -> [w1852 w1909]
              tunnel: w1832 -> [w1851 w1911]
              tunnel: w1828 -> [_ w1921]
              tunnel: w1827 -> [_ w1920]
              tunnel: w1826 -> [_ w1919]
              tunnel: w1825 -> [_ w1918]
              tunnel: w1819 -> [_ w1917]
              tunnel: w1824 -> [_ w1915]
              tunnel: [TRUE w1912] -> w1821
              tunnel: [w1848 w1910] -> w1823
              tunnel: [w1846 w1908] -> w1820
              tunnel: [0 0] -> w1817
              frame "Track", Default {
                # "Reset"
                # "Tracking Timeout"
                # "Move Delta"
                # "Goal Position"
                # "Tracking Move"
                # "Move Servo"
                # "Only Consider Tracking Angle\n\nIF\n\nImage Locked        == T\nTrack Angle Flag   == T"
                n649 = And(x=w1853, y=w1852) -> (x .and. y?=w1845:bool)
                n650 = case shown="True" w1845 {
                  tunnel: w1861 -> [_ w1867]
                  tunnel: w1860 -> [_ w1885]
                  tunnel: w1859 -> [_ w1882]
                  tunnel: w1858 -> [w1864 w1872]
                  tunnel: [w1864 w1881] -> w1856
                  tunnel: [w1866 w1880] -> w1857
                  tunnel: [w1866 w1879] -> _
                  tunnel: [u16 0 w1878] -> w1855
                  tunnel: w1854 -> [_ w1874]
                  tunnel: w1851 -> [w1863 _]
                  tunnel: [w1862 0] -> w1848
                  frame False {
                    w1866 = FALSE
                    # "Increment timeout"
                    n651 = Increment(x=w1863) -> (x+1=w1862:i32)
                  }
                  frame True {
                    # "Convert Track Angle to UINT16"
                    # "1024/300"
                    # "Move to Tracking Angle \n\nif delta is greater than move servo threshold\nAND less than max move threshold"
                    n652 = Add(x=w1885, y=w1867) -> (x+y=w1888:sgl)
                    n653 = Add(x=w1888, y=sgl 60.0) -> (x+y=w1887:sgl)
                    n654 = Multiply(x=3.413333333333333, y=w1887) -> (x*y=w1868:dbl)
                    n655 = To Word Integer(number=w1872) -> (16bit integer=w1870:i16)
                    n656 = To Unsigned Word Integer(number=w1868) -> (unsigned 16bit integer=w1884:u16)
                    n657 = To Word Integer(number=w1868) -> (16bit integer=w1883:i16)
                    n658 = Subtract(x=w1883, y=w1870) -> (x-y=w1873:i16)
                    n659 = Absolute Value(x=w1873) -> (abs(x)=w1869:i16)
                    n660 = Greater Or Equal?(x=w1869, y=w1882) -> (x >= y?=w1876:bool)
                    n661 = Less Or Equal?(x=w1869, y=w1874) -> (x <= y?=w1875:bool)
                    n662 = And(x=w1876, y=w1875) -> (x .and. y?=w1877:bool)
                    n663 = case shown="True" w1877 {
                      tunnel: w1884 -> [_ w1896]
                      tunnel: [w1891 w1896] -> w1881
                      tunnel: [w1892 w1902] -> w1880
                      tunnel: [w1892 w1902] -> w1879
                      tunnel: w1872 -> [w1891 _]
                      tunnel: w1869 -> [_ w1901]
                      tunnel: [u16 0 w1901] -> w1878
                      tunnel: w1867 -> [_ w1895]
                      frame False {
                        w1892 = FALSE
                        # "Don't Move"
                      }
                      frame True {
                        w1902 = TRUE
                        # "45 DEG MOUNT OFFSET"
                        # "1024/300"
                        # "Current Delta"
                        # "Use new Track Angle"
                        n664 = Divide(x=w1896, y=3.413333333333333) -> (x/y=w1898:dbl)
                        n665 = Negate(x=w1895) -> (-x=w1894:sgl)
                        n666 = Subtract(x=w1898, y=sgl 60.0) -> (x-y=w1900:dbl)
                        n667 = Add(x=w1900, y=w1894) -> (x+y=w1893:dbl)
                        n668 = local write "Last Track Angle - L"(w1893) -> ()
                      }
                    }
                  }
                }
                n669 = local read "Timeout to \nEnable Reactive Predict"() -> (w1849:u16)
                n670 = Less?(x=w1848, y=w1849) -> (x < y?=w1847:bool)
                n671 = case shown="True" w1847 {
                  tunnel: [enum16{"Track", "Reactive Predict", ""}."Reactive Predict" ("Initial Tracking State - Right") enum16{"Track", "Reactive Predict", ""}."Track" ("Initial Tracking State - Right")] -> w1846
                  frame False {
                  }
                  frame True {
                  }
                }
              }
              frame "Reactive Predict" {
                # "Choose New\nTracking State"
                n672 = Or(x=w1906, y=w1909) -> (x .or. y?=w1905:bool)
                n673 = case shown="False" w1905 {
                  tunnel: [w1935 w1987] -> w1922
                  tunnel: w1921 -> [w1934 _]
                  tunnel: w1920 -> [w1933 _]
                  tunnel: w1919 -> [w1932 _]
                  tunnel: w1918 -> [w1931 _]
                  tunnel: w1917 -> [w1930 _]
                  tunnel: w1915 -> [w1929 _]
                  tunnel: [w1928 w1986] -> w1914
                  tunnel: [w1927 w1986] -> w1912
                  tunnel: w1911 -> [w1926 _]
                  tunnel: [w1925 0] -> w1910
                  tunnel: [enum16{"Track", "Reactive Predict", ""}."Reactive Predict" ("Initial Tracking State - Right") enum16{"Track", "Reactive Predict", ""}."Track" ("Initial Tracking State - Right")] -> w1908
                  tunnel: w1916 -> [w1923 w1987]
                  frame False {
                    # "Stay in Reactive State"
                    # "Increment Track Timeout"
                    # "Move Respond Flag"
                    n674 = Increment(x=w1926) -> (x+1=w1925:i32)
                    n675 = case shown="True" w1930 {
                      tunnel: w1934 -> [_ w1950]
                      tunnel: w1933 -> [_ w1949]
                      tunnel: w1932 -> [_ w1948]
                      tunnel: w1931 -> [_ w1947]
                      tunnel: w1929 -> [_ w1944]
                      tunnel: [w1936 w1940] -> w1935
                      tunnel: [w1937 w1939] -> w1928
                      tunnel: [w1937 w1939] -> w1927
                      tunnel: w1923 -> [w1936 w1938]
                      frame False {
                        w1937 = FALSE
                        # "Reset Move Respond = F"
                        # "Move Servo = F"
                      }
                      frame True {
                        w1939 = TRUE
                        # "Position Lock"
                        # "Current Servo\nPosition"
                        # "Reset Move\nRespond = T"
                        # "Move Servo = T"
                        # "Apply Direction \nto Offset (delta sum)"
                        # "Check Last Known Position of Robot"
                        n676 = case shown="True" w1950 {
                          tunnel: w1949 -> [_ w1978]
                          tunnel: w1948 -> [_ w1953]
                          tunnel: w1947 -> [_ w1954]
                          tunnel: [sgl 1.0 ("y") w1952] -> w1946
                          frame False {
                            # "No Position Data Available"
                            # "Default is to move\nSame Direction as other\nServo"
                          }
                          frame True {
                            w1959 = sgl 1.0 ("y")
                            # "Use previous position/orientation to Guess Which Direction to Move Servo"
                            # "Choose Search Direction"
                            # "\"Perpendicular \nThreshold\""
                            # "If Orientation is\n ~Perpendicular -> Start Search\n in Opposite Direction of Other"
                            # "****add 90 until orientation angle is fixed"
                            # "Last Orientation"
                            # "Convert to Rad"
                            # "Avoid Divide by 0"
                            # "-1/m"
                            # "Calculate Normal Line to \nLast Robot Position\nfrom Center Beacon"
                            # "last Position \nCoordinates"
                            n677 = Unbundle(w1978) -> ("X"=w1958:sgl, "Y"=w1957:sgl)
                            n678 = Unbundle(w1954) -> ("X"=w1956:sgl, "Y"=w1955:sgl)
                            n679 = Subtract(x=w1957, y=w1955) -> (x-y=w1974:sgl)
                            n680 = Subtract(x=w1958, y=w1956) -> (x-y=w1972:sgl)
                            n681 = Equal To 0?(x=w1972) -> (x = 0?=w1973:bool)
                            n682 = case shown="False" w1973 {
                              tunnel: w1974 -> [w1981 _]
                              tunnel: w1972 -> [w1980 _]
                              tunnel: [w1979 1000000000000000.0] -> w1971
                              frame False {
                                n683 = Divide(x=w1981, y=w1980) -> (x/y=w1979:sgl)
                              }
                              frame True {
                              }
                            }
                            n684 = Equal To 0?(x=w1971) -> (x = 0?=w1976:bool)
                            n685 = case shown="False" w1976 {
                              tunnel: [w1983 1e-08] -> w1975
                              tunnel: w1971 -> [w1983 _]
                              frame False {
                              }
                              frame True {
                                # "Can't have infinit slope"
                              }
                            }
                            n686 = Divide(x=-1.0, y=w1975) -> (x/y=w1970:dbl)
                            n687 = Inverse Tangent(1:w1970) -> (0:w1968:dbl)
                            n688 = expression code="(x/pi)*180.0" "radians to degrees"(w1968) -> (w1969:dbl)
                            n689 = To Single Precision Float(number=w1969) -> (single precision float=w1966:sgl)
                            n690 = Add(x=w1953, y=sgl 90.0) -> (x+y=w1965:sgl)
                            n691 = Subtract(x=w1966, y=w1965) -> (x-y=w1964:sgl)
                            n692 = Absolute Value(x=w1964) -> (abs(x)=w1963:sgl)
                            n693 = Less Or Equal?(x=w1963, y=sgl 10.0) -> (x <= y?=w1961:bool)
                            n694 = Negate(x=w1959) -> (-x=w1960:sgl)
                            n695 = Select(t=w1960, s=w1961, f=w1959) -> (s? t:f=w1952:sgl)
                          }
                        }
                        n696 = To Word Integer(number=w1946) -> (16bit integer=w1945:i16)
                        n697 = Multiply(x=w1945, y=w1944) -> (x*y=w1943:i32)
                        n698 = To Word Integer(number=w1938) -> (16bit integer=w1942:i16)
                        n699 = Add(x=w1943, y=w1942) -> (x+y=w1941:i32)
                        n700 = To Unsigned Word Integer(number=w1941) -> (unsigned 16bit integer=w1940:u16)
                      }
                    }
                  }
                  frame True {
                    w1986 = TRUE
                    # "Go Directly to Track State"
                  }
                }
              }
            }
            n701 = local read "Tracking Timeout\nThreshold"() -> (w1830:i32)
            n702 = Less?(x=w1823, y=w1830) -> (x < y?=w1831:bool)
            n703 = case shown="False" w1831 {
              tunnel: [T2."Recovery Mode" ("Next Main State") T2."Tracking" ("Next Main State")] -> w1835
              frame False {
              }
              frame True {
              }
            }
          }
          frame "Recovery Mode" {
            w1998 = u16 0
            # "***Compltetly resets as of R17, used to just reset to \"Max Recovery Count - 1\""
            # "Increment Recoveyr Mode Count"
            # "Frames Processed"
            # "Choose Next Main State"
            # "Reset recovery count"
            # "Recovery move\nCount"
            # "Recovery Search\nAttempt count"
            # "Move Servo = T"
            # "delta move sum"
            # "Robot Position Valid"
            n704 = local read "Image Lock - Right"() -> (w2002:bool)
            n705 = Or(x=w1993, y=w1994) -> (x .or. y?=w1992:bool)
            n706 = case shown="\"Recovery Search\"" w1995 {
              tunnel: w2024 -> [_ _]
              tunnel: w2023 -> [_ _]
              tunnel: w2022 -> [_ _]
              tunnel: w2021 -> [_ _]
              tunnel: w2020 -> [_ _]
              tunnel: w2019 -> [_ _]
              tunnel: w2018 -> [w2052 w2138]
              tunnel: [w2044 w2136] -> w2017
              tunnel: [w2041 w2130] -> w2016
              tunnel: [FALSE FALSE] -> w1996
              tunnel: [w2046 w2127] -> w2015
              tunnel: w2012 -> [w2050 _]
              tunnel: w2014 -> [w2053 _]
              tunnel: w2013 -> [w2051 w2133]
              tunnel: [w2043 w2126] -> w2010
              tunnel: [w2042 w2126] -> w2011
              tunnel: w2002 -> [w2040 _]
              tunnel: [w2031 w2137] -> w2009
              tunnel: w2008 -> [w2029 w2121]
              tunnel: w2007 -> [w2034 w2134]
              tunnel: w2006 -> [w2030 w2132]
              tunnel: w1993 -> [_ _]
              tunnel: w1994 -> [_ w2129]
              tunnel: [FALSE w2128] -> w2004
              tunnel: w2001 -> [w2038 _]
              tunnel: w2000 -> [w2037 _]
              tunnel: [w2034 w2125] -> w1999
              frame "Recovery Search" {
                # "Wait for 2 Images to be Processed\nBefore Going to Next Step"
                # "Choose Next Reovery State"
                # "Recovery Search \nAttempt Count"
                # "Move Servo"
                # "Goal Position"
                # "Recovery Search\nmove Count"
                # "Attempt Recovery Search if Other Servo has Valid Angle"
                n707 = local read "Last Track Angle - R"() -> (w2033:sgl)
                n708 = Greater Or Equal?(x=w2029, y=w2030) -> (x >= y?=w2032:bool)
                n709 = case shown="True" w2032 {
                  tunnel: w2053 -> [_ w2073]
                  tunnel: [w2058 w2072] -> w2042
                  tunnel: w2052 -> [w2061 w2071]
                  tunnel: w2051 -> [_ w2070]
                  tunnel: [w2059 w2069] -> w2043
                  tunnel: [w2061 w2068] -> w2044
                  tunnel: [FALSE w2067] -> w2041
                  tunnel: w2038 -> [w2059 w2066]
                  tunnel: w2037 -> [w2058 w2065]
                  tunnel: w2040 -> [_ w2064]
                  tunnel: w2033 -> [_ w2063]
                  tunnel: [w2056 0 ("Frames Processed\nCount - in")] -> w2031
                  tunnel: w2029 -> [w2057 _]
                  frame False {
                    # "Increment Frames Processed"
                    # "WAIT"
                    n710 = Increment(x=w2057) -> (x+1=w2056:i32)
                  }
                  frame True {
                    n711 = case shown="True" w2064 {
                      tunnel: w2063 -> [_ w2086]
                      tunnel: w2066 -> [w2074 w2082]
                      tunnel: w2073 -> [_ w2087]
                      tunnel: [w2077 w2085] -> w2068
                      tunnel: [w2075 w2084] -> w2072
                      tunnel: w2065 -> [w2075 w2083]
                      tunnel: w2071 -> [w2077 w2081]
                      tunnel: w2070 -> [_ w2080]
                      tunnel: [FALSE TRUE] -> w2067
                      tunnel: [w2074 w2078] -> w2069
                      frame False {
                        # "Don't Move bc Other Servo Doesn't Have Image Lock"
                      }
                      frame True {
                        # "Move Servo = T"
                        n712 = Greater Than 0?(x=w2082) -> (x > 0?=w2088:bool)
                        n713 = case shown="False" w2088 {
                          tunnel: w2087 -> [w2095 _]
                          tunnel: w2086 -> [w2089 _]
                          tunnel: [w2094 w2105] -> w2085
                          tunnel: [w2092 w2111] -> w2084
                          tunnel: w2083 -> [w2093 w2111]
                          tunnel: w2082 -> [w2091 w2108]
                          tunnel: [w2090 w2110] -> w2078
                          tunnel: w2081 -> [_ w2106]
                          tunnel: w2080 -> [_ w2103]
                          frame False {
                            # "Increment move count to transition\nto Pan mode"
                            # "Increment Recovery Search Attempt Count"
                            # "1024/300"
                            # "Move Parallel to Other Servo"
                            n714 = Increment(x=w2093) -> (x+1=w2092:i32)
                            n715 = Add(x=w2089, y=w2095) -> (x+y=w2101:sgl)
                            n716 = Add(x=w2101, y=sgl 60.0) -> (x+y=w2100:sgl)
                            n717 = Multiply(x=3.413333333333333, y=w2100) -> (x*y=w2098:dbl)
                            n718 = Add(x=0.5, y=w2098) -> (x+y=w2096:dbl)
                            n719 = To Unsigned Word Integer(number=w2096) -> (unsigned 16bit integer=w2094:u16)
                            n720 = Increment(x=w2091) -> (x+1=w2090:i32)
                          }
                          frame True {
                            # "Apply Direction"
                            # "Step SIze"
                            # "Current Position"
                            # "Attempt to Pan in Steps Towards other Servo"
                            # "Could be same or function of \nregular search step size"
                            # "Max # of Pan\nMoves"
                            # "Pan Towards Other Servo"
                            n721 = Greater Or Equal?(x=w2108, y=u16 20) -> (x >= y?=w2109:bool)
                            n722 = case shown="False" w2109 {
                              tunnel: w2108 -> [w2119 _]
                              tunnel: [w2118 u16 0] -> w2110
                              frame False {
                                # "Increment Pan Count"
                                n723 = Increment(x=w2119) -> (x+1=w2118:i32)
                              }
                              frame True {
                                # "Reset move count"
                              }
                            }
                            n724 = local read "Recovery Search\nDirection - L"() -> (w2104:bool)
                            n725 = case shown="False" w2104 {
                              tunnel: w2106 -> [w2113 w2117]
                              tunnel: w2103 -> [w2114 w2116]
                              tunnel: [w2112 w2115] -> w2105
                              frame False {
                                # "CCW"
                                n726 = Add(x=w2113, y=w2114) -> (x+y=w2112:u16)
                              }
                              frame True {
                                # "CW"
                                n727 = Subtract(x=w2117, y=w2116) -> (x-y=w2115:u16)
                              }
                            }
                          }
                        }
                      }
                    }
                  }
                }
                n728 = local read "Max Recovery Count\n(Recovery Search)"() -> (w2035:u16)
                n729 = local read "Max Recovery\nSearch Attempts"() -> (w2036:u16)
                n730 = Less Or Equal?(x=w2042, y=w2036) -> (x <= y?=w2048:bool)
                n731 = Less Or Equal?(x=w2050, y=w2035) -> (x <= y?=w2049:bool)
                n732 = And(x=w2048, y=w2049) -> (x .and. y?=w2047:bool)
                n733 = case shown="True" w2047 {
                  tunnel: [enum16{"Generic Sweep", "Recovery Search"}."Generic Sweep" enum16{"Generic Sweep", "Recovery Search"}."Recovery Search"] -> w2046
                  frame False {
                  }
                  frame True {
                  }
                }
              }
              frame "Generic Sweep" {
                w2126 = u16 0
                # "Angle Valid?"
                # "Choose Next Recovery State"
                # "Wait for 2 Images to be Processed\nBefore Going to Next Step"
                # "New Goal Position"
                # "Move Servo"
                # "Frames Processed Count"
                n734 = Greater Or Equal?(x=w2121, y=w2132) -> (x >= y?=w2139:bool)
                n735 = case shown="True" w2139 {
                  tunnel: w2138 -> [w2155 w2167]
                  tunnel: w2133 -> [_ w2165]
                  tunnel: w2134 -> [w2154 w2164]
                  tunnel: [w2155 w2161] -> w2136
                  tunnel: [w2153 0] -> w2137
                  tunnel: [FALSE TRUE] -> w2131
                  tunnel: w2121 -> [w2156 _]
                  tunnel: [w2154 w2158] -> w2125
                  frame False {
                    # "Increment Frames Processed"
                    n736 = Increment(x=w2156) -> (x+1=w2153:i32)
                  }
                  frame True {
                    # "Reset Frames\nProcessed Count"
                    # "SWEEP SEARCH - Startup"
                    # "Multiple New Step\nby Step SIze"
                    # "F = CCW\nT = CW"
                    # "Last Direction"
                    # "Min Step"
                    # "add 10 in case\nactual position\nis lower than GP"
                    # "Set New Step #"
                    # "Choose Direction"
                    # "Nearest step"
                    # "Adjust Actual Posiiton\n to pre-determiend steps"
                    # "Move Servo 1 \"Step\" to\nSearch"
                    n737 = Add(x=5, y=w2167) -> (x+y=w2173:i32)
                    n738 = Quotient & Remainder(x=w2173, y=w2165) -> (floor(x/y)=w2171:i32)  [unwired: 1 out]
                    n739 = To Byte Integer(number=w2171) -> (8bit integer=w2162:i8)
                    n740 = Less?(x=w2162, y=1) -> (x < y?=w2168:bool)
                    n741 = case shown="False" w2168 {
                      tunnel: w2162 -> [w2184 w2192]
                      tunnel: [w2186 FALSE] -> w2158
                      tunnel: [w2185 w2192] -> w2170
                      tunnel: w2164 -> [w2183 _]
                      tunnel: w2165 -> [w2181 _]
                      frame False {
                        # "Max Step"
                        # "# of steps\nminus 1"
                        n742 = Divide(x=1024, y=w2181) -> (x/y=w2178:dbl)
                        n743 = To Unsigned Byte Integer(number=w2178) -> (unsigned 8bit integer=w2179:u8)
                        n744 = Greater Or Equal?(x=w2184, y=w2179) -> (x >= y?=w2180:bool)
                        n745 = case shown="True" w2180 {
                          tunnel: [w2187 TRUE] -> w2186
                          tunnel: [w2188 w2189] -> w2185
                          tunnel: w2184 -> [w2188 w2189]
                          tunnel: w2183 -> [w2187 _]
                          frame False {
                            # "No Need to\nChange Direction"
                          }
                          frame True {
                            # "T"
                            # "Move CW"
                          }
                        }
                      }
                      frame True {
                        # "F"
                        # "Move CCW"
                      }
                    }
                    n746 = case shown="True" w2158 {
                      tunnel: w2170 -> [w2175 w2176]
                      tunnel: [w2174 w2177] -> w2166
                      frame False {
                        # "CCW\n+1"
                        n747 = Increment(x=w2175) -> (x+1=w2174:i8)
                      }
                      frame True {
                        # "CW\n-1"
                        n748 = Decrement(x=w2176) -> (x-1=w2177:i8)
                      }
                    }
                    n749 = Multiply(x=w2166, y=w2165) -> (x*y=w2163:u16)
                    n750 = To Unsigned Word Integer(number=w2163) -> (unsigned 16bit integer=w2161:u16)
                  }
                }
                n751 = local read "Track Angle Valid  - Right"() -> (w2124:bool)
                n752 = local read "Image Lock - Right"() -> (w2123:bool)
                n753 = Or(x=w2123, y=w2124) -> (x .or. y?=w2122:bool)
                n754 = case shown="False" w2129 {
                  tunnel: [w2142 w2152] -> w2130
                  tunnel: w2131 -> [w2143 _]
                  tunnel: [w2144 enum16{"Generic Sweep", "Recovery Search"}."Generic Sweep"] -> w2127
                  tunnel: [w2141 w2152] -> w2128
                  tunnel: w2122 -> [w2140 _]
                  frame False {
                    # "Is other servo tracking?"
                    n755 = case shown="True" w2140 {
                      tunnel: [enum16{"Generic Sweep", "Recovery Search"}."Generic Sweep" enum16{"Generic Sweep", "Recovery Search"}."Recovery Search"] -> w2144
                      tunnel: w2143 -> [w2147 _]
                      tunnel: [w2147 FALSE] -> w2142
                      tunnel: [FALSE TRUE] -> w2141
                      frame False {
                        # "Stay in Sweep"
                      }
                      frame True {
                        # "G o to Recovery Search  State"
                      }
                    }
                  }
                  frame True {
                    w2152 = FALSE
                    # "Override Move Servo\nCommand bc an Angle Was Found\nduring this Step"
                    # "Stay In Sweep\nLet Main State Machine transition\ninto Tracking"
                  }
                }
              }
            }
            n756 = Increment(x=w2012) -> (x+1=w1991:i32)
            n757 = case shown="True" w2004 {
              tunnel: w1991 -> [w2027 _]
              tunnel: [w2027 0] -> w2005
              frame False {
              }
              frame True {
              }
            }
            n758 = case shown="False" w1992 {
              tunnel: [T2."Recovery Mode" ("Next Main State") T2."Tracking" ("Next Main State")] -> w2003
              frame False {
              }
              frame True {
              }
            }
          }
        }
        "Current Move Delta - L" <- w1718
        n759 = Less?(x=w1745, y=w1744) -> (x < y?=w1743:bool)
        n760 = local write "New Data  Flag\nLeft Servo"(FALSE) -> ()
        n761 = Select(t=w1744, s=w1743, f=w1745) -> (s? t:f=w1740:u16)
        n762 = Greater?(x=w1740, y=w1741) -> (0:w1742:bool)
        n763 = Select(t=w1741, s=w1742, f=w1740) -> (s? t:f=w1739:u16)
      }
    }
    "Next Main State - Left" <- w1146
    "Next Tracking State - Left" <- w1129
    "Next Recovery State - Left" <- w1127
    n764 = flat-sequence {
      tunnel: w1172 -> [w2199]
      tunnel: w1099 -> [w2198]
      tunnel: w1173 -> [w2201]
      tunnel: w1088 -> [w2200]
      tunnel: [w2199] -> w1186
      tunnel: [w2198] -> w1185
      tunnel: w1186 -> [w2207]
      tunnel: [w2206] -> w1181
      tunnel: [w2205] -> w1182
      tunnel: w1185 -> [w2204]
      frame #0 {
        # "Only Update GP if Moving Servo"
        n765 = case shown="True" w2199 {
          tunnel: w2201 -> [_ w2203]
          frame False {
          }
          frame True {
            # "Update Goal Position"
            n766 = local write "Servo Goal Position\n - Left"(w2203) -> ()
          }
        }
        n767 = case shown="True" w2198 {
          tunnel: w2200 -> [_ w2202]
          frame False {
          }
          frame True {
            # "New Direction"
            # "Update Goal Position"
            # "Update Direction"
            n768 = local write "Servo Goal Position\n - Right"(w2202) -> ()
          }
        }
      }
      frame #1 {
        # "Allow Comm Process to Take Down the Flag\nOnly Raise if not already in motion"
        n769 = local read "Servo Moving - R"() -> (w2212:bool)
        n770 = local read "Servo Moving - L"() -> (w2209:bool)
        n771 = local read "Move Servo - L"() -> (w2208:bool)
        n772 = local read "Move Servo - R"() -> (w2215:bool)
        n773 = Not(x=w2212) -> (.not. x?=w2214:bool)
        n774 = Not(x=w2209) -> (.not. x?=w2211:bool)
        n775 = And(x=w2204, y=w2214) -> (x .and. y?=w2213:bool)
        n776 = And(x=w2207, y=w2211) -> (x .and. y?=w2210:bool)
        n777 = case shown="True" w2213 {
          selector: w2213 -> [_ w2217]
          tunnel: [w2216 w2217] -> w2205
          tunnel: w2215 -> [w2216 _]
          frame False {
          }
          frame True {
          }
        }
        n778 = case shown="False" w2210 {
          selector: w2210 -> [_ w2219]
          tunnel: [w2218 w2219] -> w2206
          tunnel: w2208 -> [w2218 _]
          frame False {
          }
          frame True {
          }
        }
        n779 = local write "Move Servo - R"(w2205) -> ()
        n780 = local write "Move Servo - L"(w2206) -> ()
      }
    }
    n781 = local read "Current Main State - Right"() -> (w1151:T2)
    n782 = local read "Current Main State - Left"() -> (w1152:T2)
    n783 = Equal?(x=w1152, y=w1150) -> (x = y?=w1149:bool)
    n784 = Equal?(x=w1151, y=w1150) -> (x = y?=w1148:bool)
    n785 = And(x=w1149, y=w1181) -> (x .and. y?=w1177:bool)
    n786 = And(x=w1182, y=w1148) -> (x .and. y?=w1178:bool)
    n787 = And(x=w1149, y=w1148) -> (x .and. y?=w1176:bool)
    n788 = Exclusive Or(1:w1178, 2:w1177) -> (0:w1175:bool)
    n789 = case shown="True" w1175 {
      tunnel: [w2230 w2251] -> w1183
      tunnel: [w2231 w2250] -> w1179
      tunnel: w1098 -> [_ w2254]
      tunnel: w1139 -> [w2228 w2255]
      tunnel: w1102 -> [w2226 w2253]
      tunnel: [w2229 w2241] -> w1180
      tunnel: [w2227 w2240] -> w1184
      tunnel: w1147 -> [_ w2252]
      tunnel: w1176 -> [w2225 _]
      tunnel: w1177 -> [_ w2251]
      tunnel: w1178 -> [_ w2250]
      frame False {
        n790 = case shown="False" w2225 {
          tunnel: [w2235 w2237] -> w2231
          tunnel: [w2234 w2237] -> w2230
          tunnel: [w2233 w2236] -> w2229
          tunnel: w2228 -> [w2233 _]
          tunnel: [w2232 w2236] -> w2227
          tunnel: w2226 -> [w2232 _]
          frame False {
            # "No Movement\nRetain All Values"
            n791 = local read "Move Respond - L"() -> (w2235:bool)
            n792 = local read "Move Respond - R"() -> (w2234:bool)
          }
          frame True {
            w2236 = i16 0
            w2237 = FALSE
            # "Reset Delta Move sum\nfor both"
            # "F"
            # "Both Moved,\nMake Flags False"
          }
        }
      }
      frame True {
        w2247 = 200 ("y")
        w2238 = -200 ("y")
        # "Add/Clear Sum for \nServo That didn't move"
        # "Update Moving Servo's  Delta Position"
        # "if one Servo Moves, other should \nmove too eventually,\nUsed in Search Process"
        # "Only 1 Servo is Moving Due to Tracking --> Update delta move sum"
        n793 = case shown="True" w2250 {
          tunnel: w2255 -> [_ w2263]
          tunnel: w2254 -> [_ w2262]
          tunnel: [i16 0 w2261] -> w2248
          frame False {
          }
          frame True {
            n794 = Add(x=w2263, y=w2262) -> (x+y=w2261:i32)
          }
        }
        n795 = case shown="True" w2251 {
          tunnel: w2253 -> [_ w2259]
          tunnel: w2252 -> [_ w2258]
          tunnel: [i16 0 w2257] -> w2245
          frame False {
          }
          frame True {
            n796 = Add(x=w2259, y=w2258) -> (x+y=w2257:i32)
          }
        }
        n797 = Greater?(x=w2248, y=w2247) -> (0:w2249:bool)
        n798 = Greater?(x=w2245, y=w2247) -> (0:w2246:bool)
        n799 = Select(t=w2247, s=w2246, f=w2245) -> (s? t:f=w2242:i32)
        n800 = Select(t=w2247, s=w2249, f=w2248) -> (s? t:f=w2243:i32)
        n801 = Greater?(x=w2243, y=w2238) -> (0:w2239:bool)
        n802 = Greater?(x=w2242, y=w2238) -> (0:w2244:bool)
        n803 = Select(t=w2242, s=w2244, f=w2238) -> (s? t:f=w2240:i32)
        n804 = Select(t=w2243, s=w2239, f=w2238) -> (s? t:f=w2241:i32)
      }
    }
    n805 = case shown="True" w1094 {
      selector: w1094 -> [_ w2197]
      tunnel: [w2194 w2196] -> w1134
      tunnel: [w2193 i16 0] -> w1135
      tunnel: w1183 -> [w2194 _]
      tunnel: w1184 -> [w2193 _]
      frame False {
      }
      frame True {
        n806 = Not(x=w2197) -> (.not. x?=w2196:bool)
      }
    }
    "Move Respond - R" <- w1134
    "deltaMoveServo\n- R" <- w1135
    n807 = case shown="False" w1145 {
      selector: w1145 -> [_ w2224]
      tunnel: [w2221 w2223] -> w1137
      tunnel: [w2220 i16 0] -> w1140
      tunnel: w1179 -> [w2221 _]
      tunnel: w1180 -> [w2220 _]
      frame False {
      }
      frame True {
        n808 = Not(x=w2224) -> (.not. x?=w2223:bool)
      }
    }
    "Move Respond - L" <- w1137
    "deltaMoveServo\n- L" <- w1140
    "Current Main State - Left" <- w1171
    "Frames Processed\nCount - in -L" <- w1163
    "Recovery Mode Count - in Left" <- w1158
    "Recovery Search\nmove Count - in - L" <- w1157
    "Recovery Search\nAttempt Count - in - L" <- w1156
    "Current Main State - Right" <- w1125
    "Frames Processed\nCount - in Right" <- w1108
    "Recovery Search\nmove Count - Right" <- w1110
    "Recovery Search\nAttempt Count - Right" <- w1109
    "Recovery Mode Count in Right" <- w1101
    "Tracking Timeout\nCount - L" <- w1132
    "Tracking Timeout\nCount - R" <- w1117
    "Current Tracking State - Left" <- w1131
    "Current Tracking State - Right 2" <- w1123
    "Current Recovery State - Right" <- w1124
    "Current Recovery State -L" <- w1128
  }
